vi "Cascade front panel.vi"() -> ()   [LabVIEW 2016]
uses:
  Cascade-lv16-64/Waterloo DAQ/sdi_12/SDI-12/Sonde Vertical Graph.ctl
  Cascade-lv16-64/Waterloo DAQ/controls/Vertical Chart.ctl
  Cascade-lv16-64/Waterloo DAQ/sdi_12/Groundwater header.ctl
  Cascade-lv16-64/Waterloo DAQ/controls/MCC DAQ Setup.ctl
  Cascade-lv16-64/Waterloo DAQ/controls/Aux Sensor.ctl
  Cascade-lv16-64/Waterloo DAQ/KPRO_2016 subvis/Control 2.ctl
  Cascade-lv16-64/Waterloo DAQ/KPRO_2016 subvis/Graph Controls 2.ctl
  Cascade-lv16-64/Waterloo DAQ/KPRO_2016 subvis/Ik control.ctl
  Cascade-lv16-64/Waterloo DAQ/controls/MCC DAQ Readings.ctl
  Cascade-lv16-64/Waterloo DAQ/controls/Kpro pressure measurement cluster.ctl
  Cascade-lv16-64/Waterloo DAQ/controls/Kpro hydraulic measurement cluster.ctl
  Cascade-lv16-64/Waterloo DAQ/sdi_12/Sonde Value Percent Tol.ctl
  Cascade-lv16-64/Waterloo DAQ/activeXtest/activeXtest 2015 Folder/sample data row cluster.ctl
  Cascade-lv16-64/Waterloo DAQ/activeXtest/activeXtest 2015 Folder/sonde cluster.ctl
  Cascade-lv16-64/Waterloo DAQ/KPRO_2016 subvis/Sensor Physical Measurements.ctl
  Cascade-lv16-64/Waterloo DAQ/KPRO_2016 subvis/SS Control 7.ctl
  <vilib>/Utility/NIReport.llb/NI_report.lvclass
  Cascade-lv16-64/Waterloo DAQ/controls/Action Control 1.ctl
  Cascade-lv16-64/Waterloo DAQ/activeXtest/activeXtest 2015 Folder/sonde cluster from excel.ctl
  <extravilib>/ChannelInstances/One Element Stream-t'Action Control 1.ctl'/Instantiate.vi
  <extravilib>/ChannelInstances/One Element Stream-t'Action Control 1.ctl'/Endpoint.vi
  Cascade-lv16-64/Waterloo DAQ/KPRO_2016 subvis/Kpro Globals.vi
  <vilib>/Utility/file.llb/Write Delimited Spreadsheet (string).vi
  <vilib>/Utility/file.llb/Write Delimited Spreadsheet (DBL).vi
  <vilib>/ULx/Create Channel.llb/ULx Create Channel (AI-Voltage-Basic).vi
  <userlib>/_OpenG.lib/file/file.llb/Build Path - Traditional__ogtk.vi
  <userlib>/_OpenG.lib/file/file.llb/Strip Path - Traditional__ogtk.vi
  Cascade-lv16-64/Waterloo DAQ/KPRO_2016 subvis/Global_SIM_switch.vi
  C:/Program Files (x86)/National Instruments/LabVIEW 2016/vi.lib/ULx/ULx_LV.dll
  Program Files (x86)/National Instruments/LabVIEW 2016/vi.lib/ULx/ULx_LV.dll
  <vilib>/Utility/config.llb/NI_LVConfig.lvlib
  <extravilib>/ChannelInstances/One Element Stream-t'Action Control 1.ctl'.lvlib
panel:
  out "Column of Volume":i32
  in  "Input Variables and Slopes 2":T1={"Total Volume"=0.0, "String Pot Slope"=1.6619999408721924, "Flow Slope"=39.040000915527344, "Up Hole Pressure Slope"=48.27000045776367, "Depth to Water Table"=-0.0, "Atmospheric Pressure"=32.22022530555725, "Reservoir Pressure"=-0.004827000045779073, "Height of Sample Box"=0.0, "DH Pressure Trans Slope"=42.0, "DH Pressure Offset"=0.0, "Up Hole  Pressure Offset"=0.0, "Aux 1 Slope"=1.0, "Aux 2 Slope"=1.0, "Aux 3 Slope"=1.0} {"Aux 3 Slope" format="%.2f"; "Aux 2 Slope" format="%.2f"; "Aux 1 Slope" format="%.2f"; "Up Hole  Pressure Offset" format="%.2f"; "DH Pressure Offset" format="%.2f"; "DH Pressure Trans Slope" format="%.2f"; "Height of Sample Box" format="%.2f"; "Reservoir Pressure" format="%.2f"; "Atmospheric Pressure" format="%.2f"; "Depth to Water Table" format="%.2f"; "Up Hole Pressure Slope" format="%.2f"; "Flow Slope" format="%.2f"; "String Pot Slope" format="%.2f"; "Total Volume" format="%.2f"}
  out "Select Worksheet Index":i32
  out "Number of Sample Sheets":i32
  out "NI_report out":refnum<class "NI_report.lvclass">
  out "Sonde":bool
  out "DAQ":bool
  in  "Create Excel Files":bool
  in  "Depth mode":bool caption="Use \nIncrement"
  in  "Sample Sheet Data Row Cluster 2":T2={"Head\nPressure"=0.0, "Depth"=0.0, "comment "="", "Sonde Data Cluster"={"Cumulative\nVolume (ml)"=100.0, "Specific\nCond (mS)"=2.0, "Dissolved\nOxygen mg/L"=3.0, "pH"=4.0, "ORP"=5.0, "Temp deg C"=26.0, "Salinity"=7.0}, "Aux1"=0.0, "Aux2"=0.0, "Aux3"=0.0} {"Sonde Data Cluster"."Salinity" format="%_3g"; "Sonde Data Cluster"."Temp deg C" format="%_2g"; "Sonde Data Cluster"."ORP" format="%_4g"; "Sonde Data Cluster"."pH" format="%_4g"; "Sonde Data Cluster"."Dissolved\nOxygen mg/L" format="%_4g"; "Sonde Data Cluster"."Specific\nCond (mS)" format="%_4g"; "Sonde Data Cluster"."Cumulative\nVolume (ml)" format="%#_4g"; "Depth" format="%#.3g"; "Head\nPressure" format="%#.4g"}
  in  "Increment Depth":bool
  in  "Finish Tests":bool
  in  "Start KPRO":bool
  out "Current Time (s)":dbl
  in  "stop":bool
  in  "Write Data to Spreadsheet":bool
  in  "Sample Not Collected":bool
  in  "Record Single Sample":bool
  in  "Tab Control":T4(tab)
  out "12V Voltage Monitor":dbl format="%_3f"
  out "Found Quanta Sonde Com Port":refnum<visa-resource-name>
  in  "Data File Directory":path=path "C:/Cascade/Data/Excel Reports"
  out "Quanta Sonde found?":bool
  in  "template file path":path=path "C:/Cascade/templates/Groundwater Profiling Log_empty_labview_template.xlsx"
  in  "Config File Path":path=path "C:/Cascade/Data/config files/DAQ Setup Config.ini"
  in  "Read Configuration File?":bool
  out "H-4191 Adapter found":bool
  in  "Save Configuration File?":bool
  out "Sonde Communication Error Out":errorcluster
  in  "Search for Comm Ports?":bool=TRUE
  in  "USB Serial Port Manual Entry":refnum<visa-resource-name>="COM13"
  in  "Sonde Parameters \nTolerance Limits":T5={"SC %"=10.0, "DO %"=10.0, "pH % "=10.0, "ORP % "=10.0, "Temp % "=10.0, "Salinity %"=10.0} {"Salinity %" format="%_2f%%"; "Temp %" format="%_2f%%"; "ORP %" format="%_2f%%"; "pH %" format="%_2f%%"; "DO %" format="%_2f%%"; "SC %" format="%_2f%%"}
  in  "Sonde Parameters \nInitial Values":T6 {"Salinity Initial" format="%_2f"; "Temp Initial" format="%_2f"; "ORP  Initial" format="%_2f"; "pH Initial" format="%_2f"; "DO Initial" format="%_2f"; "SC Initial" format="%_2f"}
  in  "Header path":path=path "C:/Cascade/templates/Fields for Excel sheets.xlsx"
  out "Sensor  Real \nMeasurements":T7 {"9V Monitor" format="%#.3g"; "Aux 3" format="%#.3g"; "Aux 2" format="%#.3g"; "Aux 1" format="%#.3g"; "String Pot" format="%#.3g"; "Top String Pot" format="%#_4g"; "Downhole Pressure" format="%#_4g"; "Flow" format="%#_4g"; "Uphole Pressure" format="%#_4g"}
  in  "MCC USB-DAQ Setup":T8={"Device Name in InstaCal"="Dev0", "Omega Pressure Sensor"={"DAQ Channel"=2.0, "Input Voltage Range"=1, "Enabled"=TRUE, "Description"="Uphole Pressure"}, "McMillian 102 Flowmeter"={"DAQ Channel"=11.0, "Input Voltage Range"=0, "Enabled"=TRUE, "Description"="Flow"}, "DHT Pressure Sensor"={"DAQ Channel"=3.0, "Input Voltage Range"=1, "Enabled"=TRUE, "Description"="Downhole Pressure"}, "Top String Pot"={"DAQ Channel"=0.0, "Input Voltage Range"=0, "Enabled"=TRUE, "Description"="Top String Pot"}, "String Pot Signal"={"DAQ Channel"=1.0, "Input Voltage Range"=0, "Enabled"=TRUE, "Description"="String Pot"}, "Aux Sensor 1"={"DAQ Channel"=5.0, "Input Voltage Range"=1, "Enabled"=TRUE, "Description"="Aux 1"}, "Aux Sensor 2"={"DAQ Channel"=6.0, "Input Voltage Range"=1, "Enabled"=TRUE, "Description"="Aux 2"}, "Aux Sensor 3"={"DAQ Channel"=7.0, "Input Voltage Range"=1, "Enabled"=TRUE, "Description"="Aux 3"}, "Voltage Monitor"={"DAQ Channel"=8.0, "Input Voltage Range"=0, "Enabled"=TRUE, "Description"="9V Monitor"}} {"Voltage Monitor"."Input Voltage Range" items=["+/-10 V Range", "+/-5 V Range", "+/-2.5V Range", "+/-1.25 V Range", "+/-0.625 V Range", "+/-0.3125 V Range", "+/-0.1562V Range", "+/-0.078125 V Range"]; "Aux Sensor 3"."Input Voltage Range" items=["+/-10 V Range", "+/-5 V Range", "+/-2.5V Range", "+/-1.25 V Range", "+/-0.625 V Range", "+/-0.3125 V Range", "+/-0.1562V Range", "+/-0.078125 V Range"]; "Aux Sensor 2"."Input Voltage Range" items=["+/-10 V Range", "+/-5 V Range", "+/-2.5V Range", "+/-1.25 V Range", "+/-0.625 V Range", "+/-0.3125 V Range", "+/-0.1562V Range", "+/-0.078125 V Range"]; "Aux Sensor 1"."Input Voltage Range" items=["+/-10 V Range", "+/-5 V Range", "+/-2.5V Range", "+/-1.25 V Range", "+/-0.625 V Range", "+/-0.3125 V Range", "+/-0.1562V Range", "+/-0.078125 V Range"]; "String Pot Signal"."Input Voltage Range" items=["+/-10 V Range", "+/-5 V Range", "+/-2.5V Range", "+/-1.25 V Range", "+/-0.625 V Range", "+/-0.3125 V Range", "+/-0.1562V Range", "+/-0.078125 V Range"]; "Top String Pot"."Input Voltage Range" items=["+/-10 V Range", "+/-5 V Range", "+/-2.5V Range", "+/-1.25 V Range", "+/-0.625 V Range", "+/-0.3125 V Range", "+/-0.1562V Range", "+/-0.078125 V Range"]; "DHT Pressure Sensor"."Input Voltage Range" items=["+/-10 V Range", "+/-5 V Range", "+/-2.5V Range", "+/-1.25 V Range", "+/-0.625 V Range", "+/-0.3125 V Range", "+/-0.1562V Range", "+/-0.078125 V Range"]; "McMillian 102 Flowmeter"."Input Voltage Range" items=["+/-10 V Range", "+/-5 V Range", "+/-2.5V Range", "+/-1.25 V Range", "+/-0.625 V Range", "+/-0.3125 V Range", "+/-0.1562V Range", "+/-0.078125 V Range"]; "Omega Pressure Sensor"."Input Voltage Range" items=["+/-10 V Range", "+/-5 V Range", "+/-2.5V Range", "+/-1.25 V Range", "+/-0.625 V Range", "+/-0.3125 V Range", "+/-0.1562V Range", "+/-0.078125 V Range"]}
  out "Rate":dbl=1000.0 caption="Channel\nSample Rate (Hz)"
  out "Number \nof Channels":u16
  in  "DAQ \nData Rate S/s":dbl=3720.0 format="%#_13g"
  out "Descriptions":string[](array[string])
  out "Raw Voltages":dbl[](array[numeric])
  out "9V Voltage Monitor":dbl format="%#_3g"
  in  "Record DAQ Raw Voltages":bool
  out "Sensor Voltage Cluster":T10 {"9V Monitor" format="%#.3g"; "Aux 3" format="%#_3g"; "Aux 2" format="%#.3g"; "Aux 1" format="%#.3g"; "String Pot" format="%#.3g"; "Top String Pot" format="%#_3g"; "Downhole Pressure" format="%#.3g"; "Flow" format="%#_3g"; "Uphole Pressure" format="%-#1.3g"}
  out "Worksheet Names":string[](array[string])
  out "row max value":i32
  out "last occupied cell's name":string
  out "column max value":i32
  in  "Current Sheet":i32=1
  out "Current Sample Sheet":string="Sample 1"
  out "Columns":i32[](array[numeric])
  in  "Clear Groundwater Header Values":bool
  in  "Groundwater Header":T11
  in  "Excel report file path":path=path "C:/Cascade/Data/Excel Reports/Groundwater Profiling Log_ara1.xlsx"
  out "Data Setup Indicator":string
  in  "Start Initialization":bool
  in  "Input Variables and Slopes":T1={"Total Volume"=0.0, "String Pot Slope"=1.6619999408721924, "Flow Slope"=39.040000915527344, "Up Hole Pressure Slope"=48.27000045776367, "Depth to Water Table"=-0.0, "Atmospheric Pressure"=32.22022530555725, "Reservoir Pressure"=-0.004827000045779073, "Height of Sample Box"=0.0, "DH Pressure Trans Slope"=42.0, "DH Pressure Offset"=0.0, "Up Hole  Pressure Offset"=0.0, "Aux 1 Slope"=1.0, "Aux 2 Slope"=1.0, "Aux 3 Slope"=1.0} {"Aux 3 Slope" format="%.2f"; "Aux 2 Slope" format="%.2f"; "Aux 1 Slope" format="%.2f"; "Up Hole  Pressure Offset" format="%.2f"; "DH Pressure Offset" format="%.2f"; "DH Pressure Trans Slope" format="%.2f"; "Height of Sample Box" format="%.2f"; "Reservoir Pressure" format="%.2f"; "Atmospheric Pressure" format="%.2f"; "Depth to Water Table" format="%.2f"; "Up Hole Pressure Slope" format="%.2f"; "Flow Slope" format="%.2f"; "String Pot Slope" format="%.2f"; "Total Volume" format="%.2f"}
  out "Up Hole Pressure Offset":dbl
  out "appended path":path
  out "Down hole Pressure Transducer CSV data  path":path
  in  "Static IK path":path
  in  "Slopes File Path":path=path "C:/Cascade/Data/Output Files/slopes.csv"
  out "Output File Path":path
  out "KPRO SessionOutput File Path":path
  in  "Slopes History File Path":path=path "C:/Cascade/Data/Output Files/slopes.csv"
  out "Sonde Recording Error file":path
  out "IK Recording Error file":path
  out "Sonde Output File Path":path
  out "KPRO Cumulative Output File Path":path
  in  "Temporary Data Files Directory":path=path "C:/Cascade/Data/Output Files"
  in  "Update Sonde":bool
  in  "Sonde Data Array":T13(array[cluster]) {"Salinity"."%" format="%_2f%%"; "Salinity"."Value" format="%_4g"; "Temperature"."%" format="%_2f%%"; "Temperature"."Value" format="%_4g"; "ORP"."%" format="%_2f%%"; "ORP"."Value" format="%_4g"; "pH"."%" format="%_2f%%"; "pH"."Value" format="%_4g"; "Dissolved Oxygen"."%" format="%_2f%%"; "Dissolved Oxygen"."Value" format="%_4g"; "Sp. Conductance"."%" format="%_2f%%"; "Sp. Conductance"."Value" format="%_4g"; "Cumulative\nVolume" format="%#_4g"}
  out "Table Label":string="Data from Sample Sheet %d from Excel File"
  out "Sonde Array Size":i32
  out "Sonde Data Display":T14
  out "Temperature":cluster{"Y":dbl[], "Y":dbl[]}[](graph)
  in  "Record  Sonde Reason":bool
  in  "Select Reasons to Record Data":u16(ring) items=["Per Client Request", "Timed Out", "Sample stopped flowing", "Equipment Issue"]
  out "Sonde Recording Failure Path":path
  in  "Sonde IK Recording Failure Path":path
  out "Recording Reason Sonde array":string[][](array[string])
  out "IK Reason array":string[][](array[string])
  out "SC Reference Calibration Response":T16
  out "DO Reference Calibration Response":T16
  out "Salinity Reference Calibration Response":T16
  out "ORP Reference Calibration Response":T16
  out "pH Reference Calibration Response":T16
  out "pH Zero Calibration Response":T16
  in  "Salinity \nReference":dbl
  in  "SC \nReference":dbl
  in  "DO \nReference":dbl
  in  "ORP Reference":dbl
  in  "pH Reference":dbl
  in  "pH Zero":dbl
  in  "Record  SC Calibration":bool
  in  "Record DO Calibration":bool
  in  "Record Salinity Calibration":bool
  in  "Record ORP Calibration":bool
  in  "Record pH Calibration Reference":bool
  in  "Record pH Calibration Zero":bool
  out "KPRO Finish\nIndicator":bool
  in  "Input Depths \nand Parameters Cluster":T17={"Flow"=0.21081600494384767, "Zeroed \nPressure"=74.74207969932556, "Ik"=0.003788962123473114, "Current Depth"=-100.6, "Feet of Stainless"=40, "Start Depth"=0.0, "Abs Start Depth"=0.0} {"Abs Start Depth" format="%.2f"; "Start Depth" format="%.2f"; "Current Depth" format="%.2f"; "Ik" format="%.2f"; "Zeroed \nPressure" format="%.2f"; "Flow" format="%.2f"}
  out "Zero Pressure\nIndicator":bool
  in  "Zero\nPressure":bool caption="Zero Pressure"
  in  "enable_IKMGS_file":bool
  in  "enable_slug_file":bool
  in  "enable_kpro_file":bool=TRUE
  in  "Simulate AD6B":bool
  out "KPRO Test\nIndicator":bool
  in  "Record DTW File":bool
  in  "Zero In-Line Pressure\n(F = leave as is)":bool=TRUE
  out "Current Session":sgl[][](array[numeric]) format="%.2f"
  in  "KPRO test report header":string[](array[string])=["Time(msecs)", "Uncorrected Depth", "Corrected Depth", "Drive_Rate", "Flow", "Feet_of Stainless", "Up Hole Pressure", "IK", "Corrected Pressure", "Atm Pressure", "Depth to water", "Height of box", "Res_Pressure", "Secs_since_1_JAN_1904", "Depth jumps more than 1_foot", "Down hole Pressure"]
  in  "Depth Cluster":T18
  out "Cumulative_data_from_file":sgl[][](array[numeric]) format="%.2f"
  in  "KPRO test report header 2":string[](array[string])=["Time(msecs)", "Uncorrected Depth", "Corrected Depth", "Drive_Rate", "Flow", "Feet_of Stainless", "Up Hole Pressure", "IK", "Corrected Pressure", "Atm Pressure", "Depth to water", "Height of box", "Res_Pressure", "Secs_since_1_JAN_1904", "Depth jumps more than 1_foot", "Down hole Pressure"]
  out "Cumulative_data_ready":bool
  out "Depth Rate\nft/min":dbl format="%#.2g"
  out "Ik":dbl=0.003788962123473114 caption="Real Time - Depth vs. lk" format="%.2f"
  out "Uphole Pressure":dbl format="%.2f"
  in  "New Depth":dbl
  in  "Update Depth":bool
  in  "Select Entry for IK Log":u16(ring) items=["IK Increase", "IK stayed the Same", "IK decreased"]
  out "Large Depth IK Graph Cluster":T19={[0.003788962123473114, 0.0037174584307500765, 0.0037174584307500765, 0.0037174584307500765, 0.0037174584307500765, 0.003788962123473114], [-100.1, -100.2, -100.3, -100.4, -100.5, -100.6]}
  in  "Culmulative Graph Cluster":T20={"Cumulative - Depth vs. Ik"={[], []}, "Real Time - Depth vs. lk "={[0.003788962123473114, 0.0037174584307500765, 0.0037174584307500765, 0.0037174584307500765, 0.0037174584307500765, 0.003788962123473114], [-100.1, -100.2, -100.3, -100.4, -100.5, -100.6]}, "Cumulative - Depth vs. Drive Rate"={[], []}, "Real Time - Depth vs. Drive Rate"={[0.02036245163917736, 0.125, 0.16666666666666674, 0.16666666666666663, 0.16666666666666663, 0.16666666666666663], [-100.1, -100.2, -100.3, -100.4, -100.5, -100.6]}}
  out "Down hole Pressure":dbl format="%.2f"
  in  "Record IK Reason":bool
  in  "Corrected\n Pressure \nCluster":T21
  out "Flow":dbl format="%#.2g"
  out "Current Depth":sgl=-100.6 format="%.2f"
  out "Current \nDepth (m)":sgl=-30.661383 format="%.2f"
  in  "Read String Pot":bool
  out "Large Depth IK Graph":dbl(graph)
  out "DAQ Error":errorcluster
  out "Initialization Finished":bool=TRUE
  out "Stop":bool
  out "error out":errorcluster
  in  "error in (no error)":errorcluster
  out "producer loop":i32
  out "consumer loop":i32
  out "Active Channel Array":string[](array[string])
  out "delimited string":string
  out "Voltage Range":dbl[](array[numeric])
  out "Stop 2":bool
  out "output cluster":T3 caption="Cluster" {"Salinity" format="%_3g"; "Temp deg C" format="%_2g"; "ORP" format="%_4g"; "pH" format="%_4g"; "Dissolved\nOxygen mg/L" format="%_3g"; "Specific\nCond (mS)" format="%_4g"; "Cumulative\nVolume (ml)" format="%#_4g"}
  out "Serial Number/MISC":string
  out "subarray":string[][](array[string])
  out "Initialization":i32
  in  "Record Continuous Samples":bool
  # "ft. water"
  # "mL/min."
  # "ft. water"
  # "ft."
  # "ft."
  # "Instructions for Sonde Calibration:\n1.  Use the Record Single Point to Record the Data prior to start of\ncalibration procedure to record the initial points to the excel worksheet.\n2.  pH Calibration is a 2 step process:  A pH standard between 6.8 and 7.2 is treated as the “zero”\nand all other values are treated as the “slope”. First calibrate “zero”, then  add a second to calibrate “slope”. \n3.  Specific Conductance:  Wait for the specific conductance readings to stabilize in the calibration solution, which may\nrequire one or two minutes."
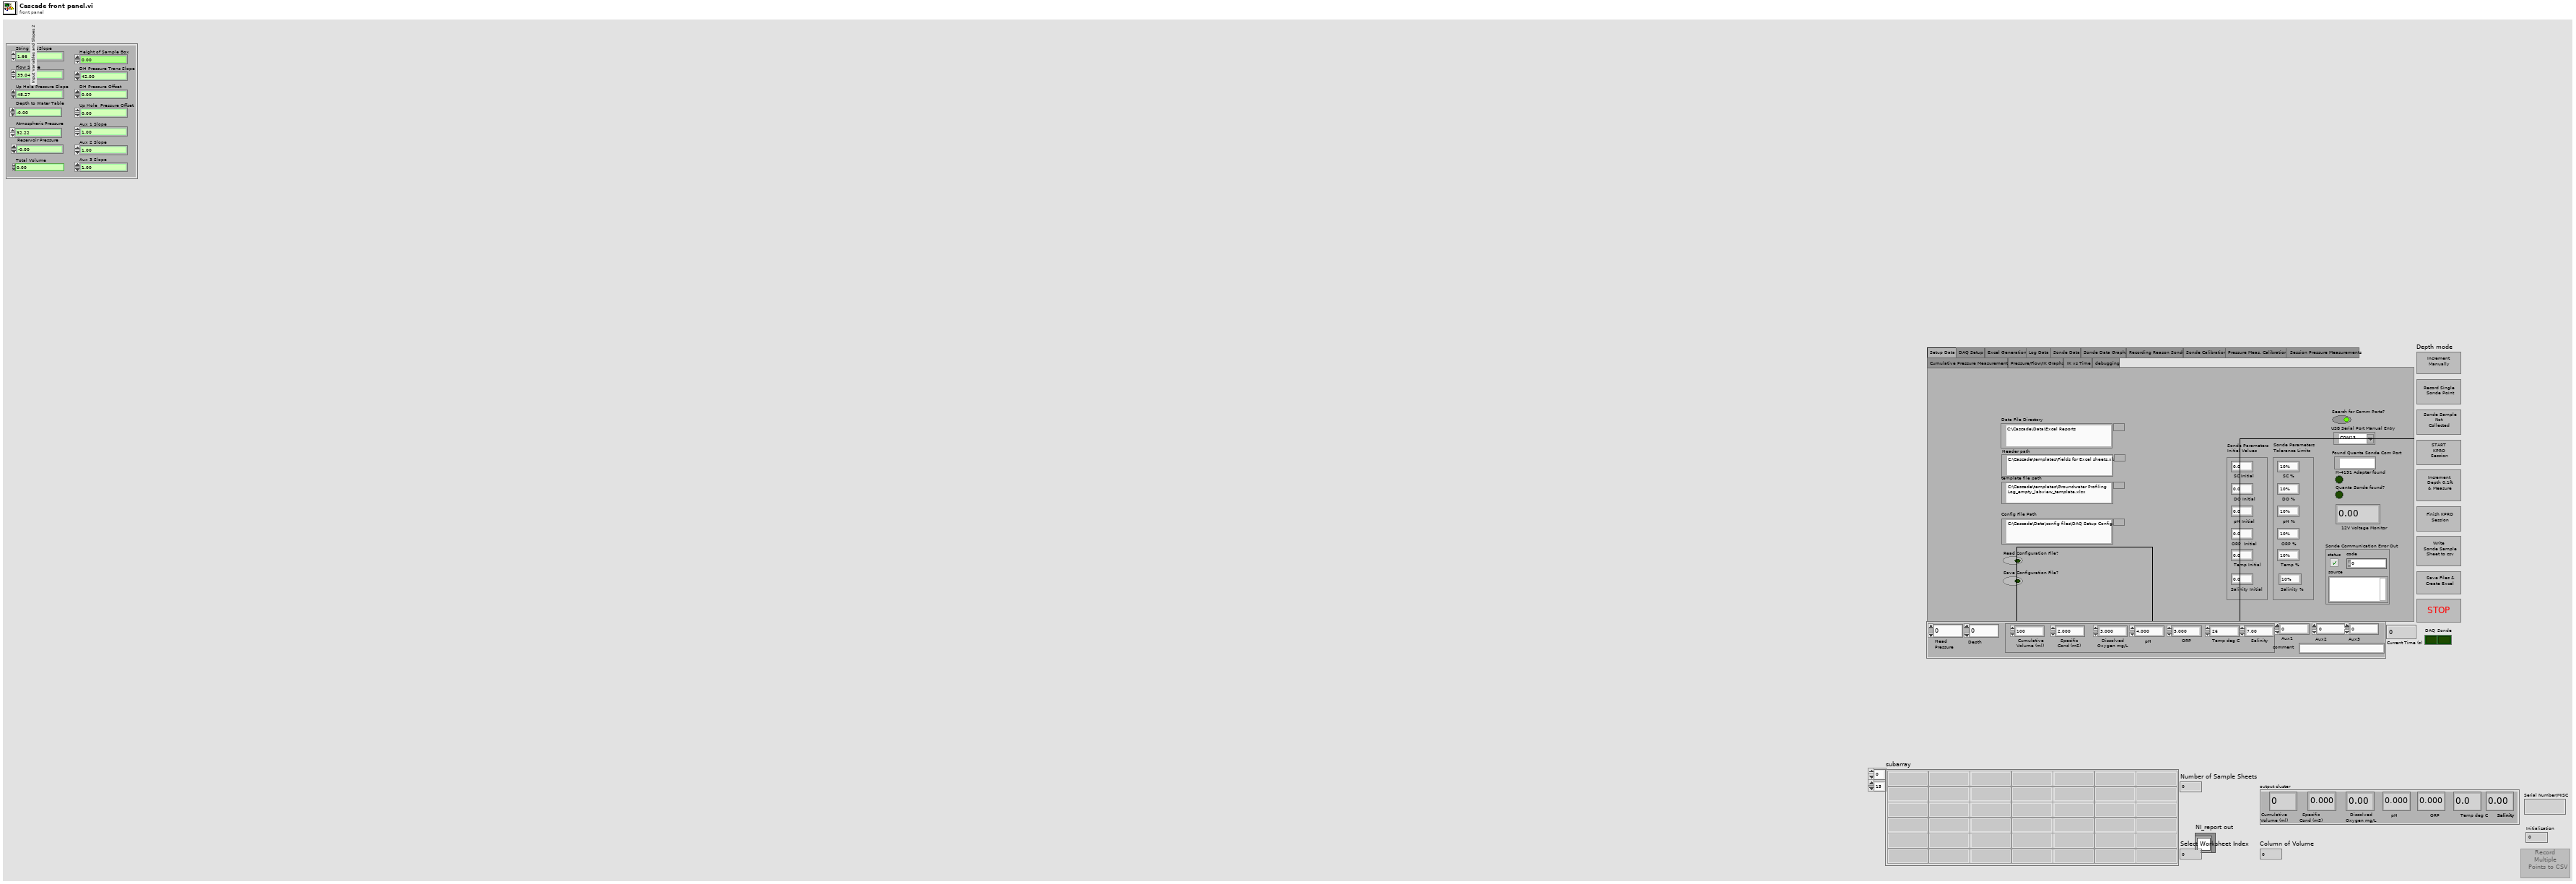
[diagram p1: front panel]
types:
  T1 = typedef "Control 2.ctl" = cluster{"Total Volume":dbl, "String Pot Slope":dbl, "Flow Slope":dbl, "Up Hole Pressure Slope":dbl, "Depth to Water Table":dbl, "Atmospheric Pressure":dbl, "Reservoir Pressure":dbl, "Height of Sample Box":dbl, "DH Pressure Trans Slope":dbl, "DH Pressure Offset":dbl, "Up Hole  Pressure Offset":dbl, "Aux 1 Slope":dbl, "Aux 2 Slope":dbl, "Aux 3 Slope":dbl}
  T2 = typedef "sample data row cluster.ctl" = cluster{"Head\nPressure":dbl, "Depth":dbl, "comment ":string, "Sonde Data Cluster":T3, "Aux1":dbl, "Aux2":dbl, "Aux3":dbl}
  T3 = typedef "sonde cluster.ctl" = cluster{"Cumulative\nVolume (ml)":dbl, "Specific\nCond (mS)":dbl, "Dissolved\nOxygen mg/L":dbl, "pH":dbl, "ORP":dbl, "Temp deg C":dbl, "Salinity":dbl}
  T4 = enum32{"Setup Data", "DAQ Setup", "Excel Generation", "Log Data", "Sonde Data", "Sonde Data Graphs", "Recording Reason Sonde", "Sonde Calibration", "Pressure Meas. Calibration", " Session Pressure Measurements", "Cumulative Pressure Measurements", "Pressure/Flow/IK Graphs", "IK vs Time ", "debugging"}
  T5 = cluster{"SC %":dbl, "DO %":dbl, "pH % ":dbl, "ORP % ":dbl, "Temp % ":dbl, "Salinity %":dbl}
  T6 = cluster{"SC Initial ":dbl, "DO Initial ":dbl, "pH Initial  ":dbl, "ORP  Initial":dbl, "Temp Initial":dbl, "Salinity Initial ":dbl}
  T7 = typedef "Sensor Physical Measurements.ctl" = cluster{"Uphole Pressure":dbl, "Flow":dbl, "Downhole Pressure":dbl, "Top String Pot":dbl, "String Pot":dbl, "Aux 1":dbl, "Aux 2":dbl, "Aux 3":dbl, "9V Monitor":dbl}
  T8 = typedef "MCC DAQ Setup.ctl" = cluster{"Device Name in InstaCal":string, "Omega Pressure Sensor":T9, "McMillian 102 Flowmeter":T9, "DHT Pressure Sensor":T9, "Top String Pot":T9, "String Pot Signal":T9, "Aux Sensor 1":T9, "Aux Sensor 2":T9, "Aux Sensor 3":T9, "Voltage Monitor":T9}
  T9 = typedef "Aux Sensor.ctl" = cluster{"DAQ Channel":dbl, "Input Voltage Range":u16, "Enabled":bool, "Description":string}
  T10 = typedef "MCC DAQ Readings.ctl" = cluster{"Uphole Pressure":dbl, "Flow":dbl, "Downhole Pressure":dbl, "Top String Pot":dbl, "String Pot":dbl, "Aux 1":dbl, "Aux 2":dbl, "Aux 3":dbl, "9V Monitor":dbl}
  T11 = typedef "Groundwater header.ctl" = cluster{"Location":string, "Date Finished":string, "CTS":string, "sampler":string, "Kpro box Serial ":string, "Sonde Serial":string, "Drilling Contractor":string, "Ave Depth to Water":string, "Gas/Peri Pump":string, "Atmospheric Pressure":string, "KPRO N2 Pressure":string, "Gas Drive N2 Pressure":string, "Profile ID":string}
  T12 = typedef "Sonde Value Percent Tol.ctl" = cluster{"Value":dbl, "%":dbl, "Tol.":bool}
  T13 = cluster{"Head":dbl, "Depth":dbl, "Time":string, "Cumulative\nVolume":dbl, "Sp. Conductance":T12, "Dissolved Oxygen":T12, "pH":T12, "ORP":T12, "Temperature":T12, "Salinity":T12, "Final Tol.":bool, "Final":bool, "Time 2":timestamp, "Aux 1":dbl, "Aux 2":dbl, "Aux 3":dbl}[]
  T14 = typedef "Sonde Vertical Graph.ctl" = cluster{"pH":T15, "Conductance":T15, "Salinity":T15, "DO % Saturation":T15, "DO mg/L":T15, "ORP":T15}
  T15 = typedef "Vertical Chart.ctl" = cluster{"Y":dbl[], "Y":dbl[]}[]
  T16 = cluster{"Valid":bool, "Value":dbl, "\nString ":string}
  T17 = typedef "SS Control 7.ctl" = cluster{"Flow":dbl, "Zeroed \nPressure":dbl, "Ik":dbl, "Current Depth":sgl, "Feet of Stainless":i32, "Start Depth":sgl, "Abs Start Depth":sgl}
  T18 = typedef "Kpro hydraulic measurement cluster.ctl" = cluster{"Absolute Depth In":dbl, "Current Absolute Depth":dbl, "First Absolute Depth":dbl, "Previous Relative Depth":dbl, "Current Relative Depth":dbl, "First Relative Depth":dbl, "Last Filed Depth":dbl, "Total Volume In":dbl, "Total Volume Out":dbl, "Current Measurement Time":dbl, "Previous Measurement Time":dbl}
  T19 = typedef "Ik control.ctl" = cluster{dbl[], dbl[]}
  T20 = typedef "Graph Controls 2.ctl" = cluster{"Cumulative - Depth vs. Ik":cluster{dbl[], dbl[]}, "Real Time - Depth vs. lk ":cluster{dbl[], dbl[]}, "Cumulative - Depth vs. Drive Rate":cluster{dbl[], dbl[]}, "Real Time - Depth vs. Drive Rate":cluster{dbl[], dbl[]}}
  T21 = typedef "Kpro pressure measurement cluster.ctl" = cluster{"Up hole Corrected Pressure":dbl, "Down hole Corrected Pressure":dbl}
  T22 = typedef "NI_LVConfig.lvlib/Config Data RefNum.ctl" = refnum<k1>
  T23 = enum8{"Enabled", "Disabled", "Disabled and Grayed Out"}
  T24 = typedef "Action Control 1.ctl" = enum16{"TimeOut", "Continuous  Sonde Data", "Init", "Exit", "Acq. Single Sonde Point", "Write Sonde Sample Sheet", "Acq. DAQ data", "Sample Not Collected", "Record Sonde Reason", "pH Calibration Zero", "pH Calibration Standard", "ORP Calibration Standard", "Salinity Calibration Standard", "DO Calibration Standard", "SC Calibration Standard", "Increment Depth Manually", "Start KPRO Measurements", "Finish KPRO Measurements", "Update Depth", "IK vs Time", "Record IK Reason", "Create Excel Files"}
  T25 = typedef "One Element Stream-t'Action Control 1.ctl'.lvlib/)Channel.ctl" = refnum<queue>
  T26 = typedef "sonde cluster from excel.ctl" = cluster{"Head":dbl, "Depth":dbl, "Time":string, "Cumulative\nVolume":dbl, "Sp. Conductance":T12, "Dissolved Oxygen":T12, "pH":T12, "ORP":T12, "Temperature":T12, "Salinity":T12, "Final Tol.":bool, "Final":bool, "Time 2":timestamp, "Aux 1":dbl, "Aux 2":dbl, "Aux 3":dbl}
  T27 = cluster{"Head":dbl, "Depth":dbl, "Time":string, "Cumulative\nVolume":dbl, "Sp. Conductance":T12, "Dissolved Oxygen":T12, "pH":T12, "ORP":T12, "Temperature":T12, "Salinity":T12, "Final Tol.":bool, "Final":bool, "Time 2":timestamp, "Aux 1":dbl, "Aux 2":dbl, "Aux 3":dbl}
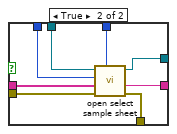
[diagram p2: hidden frame]
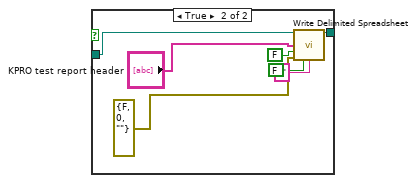
[diagram p9: hidden frame]
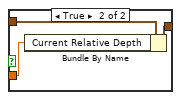
[diagram p11: hidden frame]
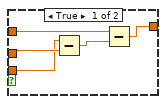
[diagram p12: hidden frame]
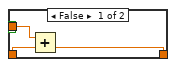
[diagram p18: hidden frame]
diagram:
  # "For calibrate command (XC) on SDI-12 address ‘a’, P is pH, C is specific conductance, S is\nsalinity or TDS, % is DO %Saturation, O is DO mg/L, R is ORP, D is depth, B is\nbarometric pressure, and t is TDS scale factor."
  n1 = flat-sequence {
    tunnel: [w20] -> w5
    tunnel: [w52] -> w7
    tunnel: w5 -> [w52]
    tunnel: [w48] -> w3
    tunnel: [w54] -> w14
    tunnel: w7 -> [w58]
    tunnel: [w54] -> w6
    tunnel: w14 -> [w108]
    tunnel: [w99] -> w12
    tunnel: [w103] -> w11
    tunnel: [w102] -> w8
    tunnel: [w100] -> w9
    tunnel: [w101] -> w10
    tunnel: [w104] -> _
    tunnel: [w106] -> w13
    tunnel: [w109] -> w2
    tunnel: [w110] -> w1
    frame #0 {
      n2 = invoke on="error out" class="Clust (strict)" method="Reinit To Default"(error in="error in (no error)") -> (error out=w18:errorcluster)  [unwired: 2 in, 2 out]
      n3 = flat-sequence {
        tunnel: [w24] -> w20
        tunnel: w18 -> [w23]
        frame #0 {
          n4 = case shown="False" "Read Configuration File?" {
            selector: "Read Configuration File?" -> [_ w31]
            tunnel: [w25 w36] -> w24
            tunnel: w23 -> [w25 w33]
            tunnel: "Config File Path" -> [_ w32]
            frame False {
            }
            frame True {
              n5 = call <vilib>:"Check if File or Folder Exists.vi"("error in (no error)"=w33, "path"=w32) -> ("error out"=w28:errorcluster, "file or folder exists?"=w29:bool, "dup path"=w27:path)  [unwired: 7 in]
              n6 = And(x=w31, y=w29) -> (x .and. y?=w30:bool)
              n7 = control-ref of="This VI"() -> (w34:refnum<vi>)
              n8 = case shown="True" w30 {
                selector: w30 -> [w37 _]
                tunnel: w27 -> [_ w42]
                tunnel: w28 -> [w38 w46]
                tunnel: [w38 w39] -> w35
                tunnel: w34 -> [_ w47]
                frame False {
                  n9 = local write "Read Configuration File?"(w37) -> ()
                }
                frame True {
                  n10 = call <vilib>:"Open Config Data.vi"("error in (no error)"=w46, "create file if necessary (T)"=FALSE, "configuration file path"=w42) -> ("error out"=w44:errorcluster, "refnum"=w45:T22)  [unwired: 6 in, 1 out]
                  n11 = call <userlib>:"Read Panel from INI__ogtk.vi"("error in (no error)"=w44, "VI ref"=w47, "refnum"=w45) -> ("error out"=w40:errorcluster, "refnum out"=w41:T22)  [unwired: 7 in]
                  n12 = call <vilib>:"Close Config Data.vi"("error in (no error)"=w40, "refnum"=w41) -> ("error out"=w39:errorcluster)  [unwired: 8 in, 1 out]
                }
              }
              n13 = call <vilib>:"Clear Errors.vi"("error in (no error)"=w35) -> ("error out"=w26:errorcluster)  [unwired: 5 in, 1 out]
              n14 = Merge Errors(w26) -> (w36:errorcluster)
            }
          }
        }
      }
    }
    frame #1 {
      n15 = invoke on="Current Session" class="Arr (strict)" method="Reinit To Default"() -> ()  [unwired: 3 in, 3 out]
      n16 = control-ref of="Sonde Data Display"() -> ()  [unwired: 1 out]
      n17 = local write "Current Sheet"(1 ("Current Sheet")) -> ()
      n18 = Get Date/Time In Seconds() -> (seconds since 1Jan1904=w48:timestamp)
      n19 = Get Date/Time In Seconds() -> (seconds since 1Jan1904=w49:timestamp)
      n20 = Subtract(x=w48, y=w49) -> (x-y=w50:dbl)
      n21 = To Double Precision Float(number=w50) -> (double precision float=→"Current Time (s)":dbl)
    }
    frame #2 {
      w66 = T23."Enabled" ("Disabled")
      w84 = T23."Disabled and Grayed Out" ("Disabled")
      n22 = invoke on="Current Sheet" class="DigNum (strict)" method="Reinit To Default"(error in=w58) -> (error out=w78:errorcluster)  [unwired: 2 in, 2 out]
      n23 = local write "Initialization Finished"(FALSE ("Initialization Finished")) -> ()
      n24 = invoke on="Sample Not Collected" class="Bool" method="Reinit To Default"(error in=w78) -> (error out=w81:errorcluster)  [unwired: 2 in, 2 out]
      n25 = invoke on="Record Continuous Samples" class="Bool" method="Reinit To Default"(error in=w81) -> (error out=w80:errorcluster)  [unwired: 2 in, 2 out]
      n26 = invoke on="Write Data to Spreadsheet" class="Bool" method="Reinit To Default"(error in=w80) -> (error out=w79:errorcluster)  [unwired: 2 in, 2 out]
      n27 = call "search for Quanta Sonde devices.vi"("VISA resource name"="USB Serial Port Manual Entry", "Search for Comm Ports?"="Search for Comm Ports?", "error in (no error)"=w58) -> ("12V monitor"=w65:dbl, "Com Port with Quanta Sonde devices"=w90:refnum<visa-resource-name>[], "Number of Quanta Sonde devices"=w89:i32, "Serial Number/MISC"=w68:string, "Number of Quanta Sonde devices > 0?"=→"Quanta Sonde found?":bool, "H-4191 Adapter found"=→"H-4191 Adapter found":bool, "Error Out"=w73:errorcluster)  [unwired: 4 in, 2 out]
      "12V Voltage Monitor" <- w65
      "Sonde Communication Error Out" <- w73
      "Serial Number/MISC" <- w68
      n28 = invoke on="Record Single Sample" class="Bool" method="Reinit To Default"(error in=w79) -> (error out=w57:errorcluster)  [unwired: 2 in, 2 out]
      n29 = property on="Record Continuous Samples" class="Bool"(error in=w57, "DisabledEnum"=w84) -> (error out=w85:errorcluster)  [unwired: 1 in, 1 out]
      n30 = local read "Groundwater Header"() -> (w67:T11)
      n31 = Greater Or Equal?(x=w65, y=11.75) -> (x >= y?=→"Sonde":bool)
      n32 = case shown="1" w89 {
        tunnel: w90 -> [_ w97]
        tunnel: [refnum<visa-resource-name> refnum ("RS232 Port Out") w95] -> w88
        frame 0, Default {
        }
        frame 1 {
          n33 = Index Array(array=w97, index=0) -> (element=w95:refnum<visa-resource-name>)
        }
      }
      "Found Quanta Sonde Com Port" <- w88
      n34 = property on="Record Single Sample" class="Bool"(error in=w85, "DisabledEnum"=w84) -> (error out=w86:errorcluster)  [unwired: 1 in, 1 out]
      n35 = invoke on="stop" class="Bool (strict)" method="Reinit To Default"(error in=w57) -> (error out=w83:errorcluster)  [unwired: 2 in, 2 out]
      n36 = Bundle By Name(cluster=w67, "Sonde Serial"=w68) -> (w69:T11)
      n37 = invoke on="Stop" class="Bool (strict)" method="Reinit To Default"(error in=w57) -> (error out=w75:errorcluster)  [unwired: 2 in, 2 out]
      n38 = property on="Sample Not Collected" class="Bool"(error in=w86, "DisabledEnum"=w84) -> (error out=w82:errorcluster)  [unwired: 1 in, 1 out]
      n39 = local write "Groundwater Header"(w69) -> ()
      n40 = property on="Write Data to Spreadsheet" class="Bool"(error in=w83, "DisabledEnum"=w84) -> (error out=w76:errorcluster)  [unwired: 1 in, 1 out]
      n41 = invoke on="Stop 2" class="Bool (strict)" method="Reinit To Default"(error in=w75) -> (error out=w74:errorcluster)  [unwired: 2 in, 2 out]
      n42 = call <vilib>:"Clear Errors.vi"("error in (no error)"=w73) -> ("error out"=w72:errorcluster)  [unwired: 5 in, 1 out]
      n43 = Merge Errors(w72, w74, w76, w82) -> (w55:errorcluster)
      n44 = flat-sequence {
        tunnel: [w93] -> w62
        tunnel: w55 -> [w93]
        frame #0 {
          n45 = local write "Tab Control"(T4."Log Data" ("Tab Control")) -> ()
        }
      }
      n46 = invoke on="Sonde Data Array" class="Arr (strict)" method="Reinit To Default"(error in=w62) -> (error out=w61:errorcluster)  [unwired: 2 in, 2 out]
      n47 = invoke on="Data Setup Indicator" class="Str" method="Reinit To Default"(error in=w61) -> (error out=w59:errorcluster)  [unwired: 2 in, 2 out]
      n48 = property on="Clear Groundwater Header Values" class="Bool"(error in=w59, "DisabledEnum"=w66) -> (error out=w60:errorcluster)  [unwired: 1 in, 1 out]
      n49 = property on="Start Initialization" class="Bool"(error in=w60, "DisabledEnum"=w66) -> (error out=w56:errorcluster)  [unwired: 1 in, 1 out]
      n50 = invoke on="Clear Groundwater Header Values" class="Bool" method="Reinit To Default"(error in=w56) -> (error out=w54:errorcluster)  [unwired: 2 in, 2 out]
    }
    frame #3 {
      n51 = while {
        tunnel: w108 -> [w118]
        tunnel: [w119] -> w105
        tunnel: [w124] -> _
        i -> [w124]
        stop <- w120 stop-if-true
        n52 = event shown="[3] \"Stop\": Value Change" {
          selector: _ -> [_ _ _ _ _]
          dyn-events: _ -> [_ _ _ _ _]
          timeout: 100 -> [_ _ _ _ _]
          tunnel: [FALSE w134 TRUE ("Stop") w139 _] -> w126
          tunnel: w118 -> [_ _ _ _ w142]
          event Timeout {
            n53 = event-data() -> ()  [unwired: 1 in, 3 out]
          }
          event "Start Initialization": Value Change {
            n54 = event-data() -> ()  [unwired: 1 in, 3 out]
            n55 = case shown="True" "Start Initialization" {
              tunnel: [FALSE ("Stop") TRUE ("Stop")] -> w134
              frame False {
              }
              frame True {
                n56 = invoke on="Data Setup Indicator" class="Str" method="Reinit To Default"() -> ()  [unwired: 3 in, 3 out]
                n57 = invoke on="Start Initialization" class="Bool" method="Reinit To Default"() -> ()  [unwired: 3 in, 3 out]
              }
            }
          }
          event Panel Close? {
            n58 = event-data() -> ()  [unwired: 1 in, 4 out]
            n59 = event-data() -> ()  [unwired: 2 in, 1 out]
          }
          event "Stop": Value Change {
            n60 = event-data() -> ()  [unwired: 1 in, 6 out]
            n61 = local read "stop"() -> (w138:bool)
            n62 = case shown="True" w138 {
              selector: w138 -> [w140 _]
              tunnel: [w140 TRUE] -> w139
              tunnel: w138 -> [_ _]
              frame False {
              }
              frame True {
              }
            }
          }
          event "Clear Groundwater Header Values": Value Change {
            n63 = event-data() -> ()  [unwired: 1 in, 6 out]
            n64 = case shown="True" "Clear Groundwater Header Values" {
              tunnel: w142 -> [_ w144]
              frame False {
              }
              frame True {
                n65 = invoke on="Groundwater Header" class="Clust (strict)" method="Reinit To Default"(error in=w144) -> (error out=w145:errorcluster)  [unwired: 2 in, 2 out]
                n66 = flat-sequence {
                  tunnel: w145 -> [_]
                  frame #0 {
                    n67 = local read "Groundwater Header"() -> (w146:T11)
                    n68 = local read "Serial Number/MISC"() -> (w147:string)
                    n69 = Bundle By Name(cluster=w146, "Sonde Serial"=w147) -> (w148:T11)
                    n70 = local write "Groundwater Header"(w148) -> ()
                  }
                }
              }
            }
          }
        }
        n71 = call <userlib>:"Wait (ms)__ogtk.vi"("error in (no error)"=w118, "milliseconds to wait"=u32 100) -> ("error out"=w119:errorcluster)  [unwired: 8 in, 1 out]
        n72 = Quotient & Remainder(x=w124, y=100) -> (floor(x/y)=w121:i32)  [unwired: 1 out]
        n73 = case shown="1, Default" w121 {
          tunnel: w119 -> [w129 w131]
          frame 1, Default {
            n74 = property on="Data Setup Indicator" class="Str"(error in=w129, "Text.TextColor"=u32 0) -> ()  [unwired: 1 in, 2 out]
          }
          frame 0 {
            n75 = property on="Data Setup Indicator" class="Str"(error in=w131, "Text.TextColor"=u32 16716800) -> ()  [unwired: 1 in, 2 out]
          }
        }
        n76 = local read "stop"() -> (w117:bool)
        n77 = Compound Arithmetic op=OR(w119, w126, w117) -> (w120:bool)
        "Data Setup Indicator" <- "Hit the Start Key after Data Entry of Log Parameters and File Names." ("Data Setup Indicator")
      }
      n78 = invoke on="stop" class="Bool (strict)" method="Reinit To Default"(error in=w105) -> (error out=w98:errorcluster)  [unwired: 2 in, 2 out]
      n79 = flat-sequence {
        tunnel: w98 -> [w155]
        tunnel: [w149] -> w107
        frame #0 {
          w156 = T23."Disabled and Grayed Out" ("Disabled")
          n80 = local write "KPRO Finish\nIndicator"(FALSE ("KPRO Finish\nIndicator")) -> ()
          n81 = invoke on="Start KPRO" class="Bool" method="Reinit To Default"(error in=w155) -> (error out=w154:errorcluster)  [unwired: 2 in, 2 out]
          n82 = invoke on="Finish Tests" class="Bool" method="Reinit To Default"(error in=w154) -> (error out=w153:errorcluster)  [unwired: 2 in, 2 out]
          n83 = invoke on="Sonde Array Size" class="DigNum (strict)" method="Reinit To Default"() -> ()  [unwired: 3 in, 3 out]
          n84 = invoke on="Increment Depth" class="Bool" method="Reinit To Default"(error in=w153) -> (error out=w152:errorcluster)  [unwired: 2 in, 2 out]
          n85 = property on="Clear Groundwater Header Values" class="Bool"(error in=w152, "DisabledEnum"=w156) -> (error out=w151:errorcluster)  [unwired: 1 in, 1 out]
          n86 = property on="Start Initialization" class="Bool"(error in=w151, "DisabledEnum"=w156) -> (error out=w150:errorcluster)  [unwired: 1 in, 1 out]
          n87 = invoke on="Update Sonde" class="Bool (strict)" method="Reinit To Default"(error in=w150) -> (error out=w149:errorcluster)  [unwired: 2 in, 2 out]
        }
      }
      n88 = flat-sequence {
        tunnel: [w159] -> w110
        tunnel: [w159] -> w109
        tunnel: [w164] -> w106
        tunnel: w107 -> [w163]
        frame #0 {
          n89 = Unbundle By Name("Input Variables and Slopes") -> ("Depth to Water Table"=w169:dbl)
          n90 = local read "Input Depths \nand Parameters Cluster"() -> (w161:T17)
          n91 = Bundle By Name(cluster="Input Variables and Slopes", "Depth to Water Table"=w169) -> (w166:T1)
          n92 = call <vilib>:"Check if File or Folder Exists.vi"("error in (no error)"=w163, "path"="Slopes File Path") -> ("error out"=w162:errorcluster, "file or folder exists?"=w158:bool, "dup path"=w167:path)  [unwired: 7 in]
          n93 = case shown="True" w158 {
            tunnel: w167 -> [_ w185]
            tunnel: w166 -> [w173 w184]
            tunnel: [w173 w183] -> w165
            tunnel: w162 -> [w172 w179]
            tunnel: [w172 w179] -> w164
            frame False {
              n94 = local write "Data Setup Indicator"("Slope file not found." ("Data Setup Indicator")) -> ()
            }
            frame True {
              n95 = call "Get_SLOPE_data_from_file 2016.vi"("Slopes File Path"=w185) -> ("Last Aux 1 Slope"=w178:dbl, "Last_String_Pot_Slope"=w182:dbl, "DHT Offset"=w174:dbl, "DHT Slope"=w175:dbl, "Last_Flow_Slope"=w181:dbl, "Last Aux 2 Slope"=w177:dbl, "Last Aux 3 Slope"=w176:dbl, "Last_Pressure_Slope"=w180:dbl)  [unwired: 6 in, 1 out]
              n96 = Bundle By Name(cluster=w184, "String Pot Slope"=w182, "Flow Slope"=w181, "Up Hole Pressure Slope"=w180, "Aux 1 Slope"=w178, "Aux 2 Slope"=w177, "Aux 3 Slope"=w176, "DH Pressure Trans Slope"=w175, "DH Pressure Offset"=w174) -> (w183:T1)
            }
          }
          n97 = Unbundle By Name(w161) -> ("Feet of Stainless"=w159:i32)
          n98 = Bundle By Name(cluster=w161, "Feet of Stainless"=w159) -> (w160:T17)
          n99 = local write "Input Depths \nand Parameters Cluster"(w160) -> ()
          n100 = local write "Input Variables and Slopes"(w165) -> ()
        }
      }
      n101 = flat-sequence {
        tunnel: [w116] -> w104
        tunnel: [w115] -> w103
        tunnel: [w114] -> w102
        tunnel: [w113] -> w101
        tunnel: [w112] -> w100
        tunnel: [w111] -> w99
        frame #0 {
          n102 = local read "Column of Volume"() -> (w112:i32)
          n103 = local read "NI_report out"() -> (w111:refnum<class "NI_report.lvclass">)
          n104 = local read "Select Worksheet Index"() -> (w116:i32)
          n105 = local read "Number of Sample Sheets"() -> (w114:i32)
          n106 = local read "Columns"() -> (w113:i32[])
          n107 = local read "Worksheet Names"() -> (w115:string[])
        }
      }
    }
  }
  n108 = flat-sequence {
    tunnel: [w189] -> w17
    tunnel: w13 -> [w188]
    tunnel: [w187] -> w4
    frame #0 {
      w186 = Action_Control_1."Init"  # Event
      n109 = while {
        shift-right: [w197] -> w189
        shift-left: w188 -> [w197]
        shift-right: [w192] -> _
        shift-left: w186 -> [w190]
        tunnel: [w198] -> w187
        i -> [w196]
        stop <- w194 stop-if-true
        # "User Interface Producer Loop"
        n110 = First Call?() -> (First Call?: T/F=w191:bool)
        n111 = case shown="False" w191 {
          tunnel: w197 -> [w203 _]
          tunnel: [w201 FALSE ("Boolean")] -> w194
          tunnel: [w200 w395] -> w192
          tunnel: w190 -> [_ w395]
          frame False {
            w199 = Action_Control_1."TimeOut"  # Event
            n112 = event shown="[0] Timeout" {
              selector: _ -> [_ _ _ _ _ _ _ _ _ _ _ _ _ _ _ _ _ _ _ _]
              dyn-events: _ -> [_ _ _ _ _ _ _ _ _ _ _ _ _ _ _ _ _ _ _ _]
              timeout: 100 -> [_ _ _ _ _ _ _ _ _ _ _ _ _ _ _ _ _ _ _ _]
              tunnel: [w204 w210 w216 w229 w239 w248 w260 w272 w284 w296 w308 w321 w332 w342 w350 w358 w366 w375 w383 _] -> w200
              tunnel: [FALSE w209 w217 w230 w240 w249 w261 w273 w285 w297 w309 w320 w331 w343 w351 w359 w367 w376 w384 _] -> w201
              tunnel: w203 -> [_ w207 w219 w232 _ w251 w263 w275 w287 w299 w311 _ w328 _ _ _ _ _ _ _]
              tunnel: [_ w207 w218 w231 _ w250 w262 w274 w286 w298 w310 _ _ _ _ _ _ _ _ _] -> _
              tunnel: w199 -> [w204 w206 w215 w228 _ w247 w259 w271 w283 w295 w307 w319 w326 w340 w348 w357 w365 w374 w382 _]
              event Timeout {
                n113 = event-data() -> ()  [unwired: 1 in, 3 out]
              }
              event "stop": Value Change {
                n114 = event-data() -> ()  [unwired: 1 in, 6 out]
                n115 = case shown="False" "stop" {
                  tunnel: [w211 w213] -> w210
                  tunnel: [FALSE TRUE] -> w209
                  tunnel: w206 -> [w211 _]
                  frame False {
                  }
                  frame True {
                    w213 = Action_Control_1."Exit"  # Event
                  }
                }
              }
              event "Record DAQ Raw Voltages": Value Change {
                n116 = event-data() -> ()  [unwired: 1 in, 6 out]
                n117 = case shown="False" "Record DAQ Raw Voltages" {
                  tunnel: [w221 w224] -> w216
                  tunnel: [FALSE FALSE ("Boolean")] -> w217
                  tunnel: [w222 w225] -> w218
                  tunnel: w219 -> [w222 w225]
                  tunnel: w215 -> [w221 _]
                  frame False {
                  }
                  frame True {
                    w224 = Action_Control_1."Acq. DAQ data"  # Event
                  }
                }
              }
              event "Record pH Calibration Zero": Value Change {
                n118 = event-data() -> ()  [unwired: 1 in, 6 out]
                n119 = case shown="True" "Record pH Calibration Zero" {
                  tunnel: [w233 w236] -> w229
                  tunnel: [FALSE FALSE ("Boolean")] -> w230
                  tunnel: [w234 w237] -> w231
                  tunnel: w232 -> [w234 w237]
                  tunnel: w228 -> [w233 _]
                  frame False {
                  }
                  frame True {
                    w236 = Action_Control_1."pH Calibration Zero"  # Event
                  }
                }
              }
              event "Create Excel Files": Value Change {
                n120 = event-data() -> ()  [unwired: 1 in, 6 out]
                n121 = case shown="True" "Create Excel Files" {
                  selector: "Create Excel Files" -> [w243 _]
                  tunnel: [w243 TRUE] -> w240
                  tunnel: [w242 w244] -> w239
                  frame False {
                    w242 = Action_Control_1."TimeOut"  # Event
                  }
                  frame True {
                    w244 = Action_Control_1."Create Excel Files"  # Event
                  }
                }
              }
              event "Record pH Calibration Reference": Value Change {
                n122 = event-data() -> ()  [unwired: 1 in, 6 out]
                n123 = case shown="True" "Record pH Calibration Reference" {
                  tunnel: [w252 w255] -> w248
                  tunnel: [FALSE FALSE ("Boolean")] -> w249
                  tunnel: [w253 w256] -> w250
                  tunnel: w251 -> [w253 w256]
                  tunnel: w247 -> [w252 _]
                  frame False {
                  }
                  frame True {
                    w255 = Action_Control_1."pH Calibration Standard"  # Event
                  }
                }
              }
              event "Record ORP Calibration": Value Change {
                n124 = event-data() -> ()  [unwired: 1 in, 6 out]
                n125 = case shown="True" "Record ORP Calibration" {
                  tunnel: [w264 w267] -> w260
                  tunnel: [FALSE FALSE ("Boolean")] -> w261
                  tunnel: [w265 w268] -> w262
                  tunnel: w263 -> [w265 w268]
                  tunnel: w259 -> [w264 _]
                  frame False {
                  }
                  frame True {
                    w267 = Action_Control_1."ORP Calibration Standard"  # Event
                  }
                }
              }
              event "Record Salinity Calibration": Value Change {
                n126 = event-data() -> ()  [unwired: 1 in, 6 out]
                n127 = case shown="True" "Record Salinity Calibration" {
                  tunnel: [w276 w279] -> w272
                  tunnel: [FALSE FALSE ("Boolean")] -> w273
                  tunnel: [w277 w280] -> w274
                  tunnel: w275 -> [w277 w280]
                  tunnel: w271 -> [w276 _]
                  frame False {
                  }
                  frame True {
                    w279 = Action_Control_1."Salinity Calibration Standard"  # Event
                  }
                }
              }
              event "Record DO Calibration": Value Change {
                n128 = event-data() -> ()  [unwired: 1 in, 6 out]
                n129 = case shown="True" "Record DO Calibration" {
                  tunnel: [w288 w291] -> w284
                  tunnel: [FALSE FALSE ("Boolean")] -> w285
                  tunnel: [w289 w292] -> w286
                  tunnel: w287 -> [w289 w292]
                  tunnel: w283 -> [w288 _]
                  frame False {
                  }
                  frame True {
                    w291 = Action_Control_1."DO Calibration Standard"  # Event
                  }
                }
              }
              event "Record  SC Calibration": Value Change {
                n130 = event-data() -> ()  [unwired: 1 in, 6 out]
                n131 = case shown="True" "Record  SC Calibration" {
                  tunnel: [w300 w303] -> w296
                  tunnel: [FALSE FALSE ("Boolean")] -> w297
                  tunnel: [w301 w304] -> w298
                  tunnel: w299 -> [w301 w304]
                  tunnel: w295 -> [w300 _]
                  frame False {
                  }
                  frame True {
                    w303 = Action_Control_1."SC Calibration Standard"  # Event
                  }
                }
              }
              event "Increment Depth": Value Change {
                n132 = event-data() -> ()  [unwired: 1 in, 6 out]
                n133 = case shown="True" "Increment Depth" {
                  tunnel: [w312 w315] -> w308
                  tunnel: [FALSE FALSE ("Boolean")] -> w309
                  tunnel: [w313 w316] -> w310
                  tunnel: w311 -> [w313 w316]
                  tunnel: w307 -> [w312 _]
                  frame False {
                  }
                  frame True {
                    w315 = Action_Control_1."Increment Depth Manually"  # Event
                  }
                }
              }
              event "Record Single Sample": Value Change {
                n134 = event-data() -> ()  [unwired: 1 in, 6 out]
                n135 = case shown="True" "Record Single Sample" {
                  tunnel: [w322 w324] -> w321
                  tunnel: [FALSE FALSE] -> w320
                  tunnel: w319 -> [w322 _]
                  frame False {
                  }
                  frame True {
                    w324 = Action_Control_1."Acq. Single Sonde Point"  # Event
                  }
                }
              }
              event "Write Data to Spreadsheet": Value Change {
                n136 = event-data() -> ("OldVal"=w330:bool, "NewVal"=w333:bool)  [unwired: 1 in, 4 out]
                n137 = Not(x=w330) -> (.not. x?=w329:bool)
                n138 = And(x=w329, y=w333) -> (x .and. y?=w327:bool)
                n139 = case shown="True" w327 {
                  tunnel: [w334 w337] -> w332
                  tunnel: [FALSE FALSE ("Boolean")] -> w331
                  tunnel: [w335 w338] -> _
                  tunnel: w328 -> [w335 w338]
                  tunnel: w326 -> [w334 _]
                  frame False {
                  }
                  frame True {
                    w337 = Action_Control_1."Write Sonde Sample Sheet"  # Event
                  }
                }
              }
              event "Sample Not Collected": Value Change {
                n140 = event-data() -> ("NewVal"=w341:bool)  [unwired: 1 in, 5 out]
                n141 = case shown="True" w341 {
                  tunnel: [FALSE FALSE] -> w343
                  tunnel: [w344 w346] -> w342
                  tunnel: w340 -> [_ w346]
                  frame True {
                    w344 = Action_Control_1."Sample Not Collected"  # Event
                  }
                  frame False {
                  }
                }
              }
              event "Record  Sonde Reason": Value Change {
                n142 = event-data() -> ("NewVal"=w349:bool)  [unwired: 1 in, 5 out]
                n143 = case shown="True" w349 {
                  tunnel: [FALSE FALSE] -> w351
                  tunnel: [w352 w354] -> w350
                  tunnel: w348 -> [_ w354]
                  frame True {
                    w352 = Action_Control_1."Record Sonde Reason"  # Event
                  }
                  frame False {
                  }
                }
              }
              event "Start KPRO": Value Change {
                n144 = event-data() -> ()  [unwired: 1 in, 6 out]
                n145 = case shown="True" "Start KPRO" {
                  tunnel: [FALSE FALSE] -> w359
                  tunnel: [w361 w363] -> w358
                  tunnel: w357 -> [_ w363]
                  frame True {
                    w361 = Action_Control_1."Start KPRO Measurements"  # Event
                    n146 = local write "KPRO Finish\nIndicator"(FALSE ("KPRO Finish\nIndicator")) -> ()
                  }
                  frame False {
                  }
                }
              }
              event "Update Depth": Value Change {
                n147 = event-data() -> ()  [unwired: 1 in, 6 out]
                n148 = case shown="True" "Update Depth" {
                  tunnel: [FALSE FALSE] -> w367
                  tunnel: [w369 w371] -> w366
                  tunnel: w365 -> [_ w371]
                  frame True {
                    w369 = Action_Control_1."Update Depth"  # Event
                  }
                  frame False {
                  }
                }
              }
              event "Record IK Reason": Value Change {
                n149 = event-data() -> ()  [unwired: 1 in, 6 out]
                n150 = case shown="True" "Record IK Reason" {
                  tunnel: [FALSE FALSE] -> w376
                  tunnel: [w377 w379] -> w375
                  tunnel: w374 -> [_ w379]
                  frame True {
                    w377 = Action_Control_1."Record IK Reason"  # Event
                  }
                  frame False {
                  }
                }
              }
              event "Finish Tests": Value Change {
                n151 = event-data() -> ()  [unwired: 1 in, 6 out]
                n152 = case shown="True" "Finish Tests" {
                  tunnel: [FALSE FALSE] -> w384
                  tunnel: [w386 w388] -> w383
                  tunnel: w382 -> [_ w388]
                  frame True {
                    w386 = Action_Control_1."Finish KPRO Measurements"  # Event
                    "KPRO Finish\nIndicator" <- TRUE ("KPRO Finish\nIndicator")
                  }
                  frame False {
                  }
                }
              }
              event "Depth mode": Value Change {
                n153 = event-data() -> ()  [unwired: 1 in, 6 out]
                n154 = case shown="True" "Depth mode" {
                  tunnel: [FALSE ("Read String Pot") TRUE ("Read String Pot")] -> w390
                  frame False {
                  }
                  frame True {
                  }
                }
                n155 = local write "Read String Pot"(w390) -> ()
              }
            }
          }
          frame True {
          }
        }
        "Stop" <- w194
        n156 = local read "Stop"() -> (w195:bool)
        n157 = Or(x=w195, y=w194) -> ()  [unwired: 1 out]
        n158 = call <extravilib>:"Write With Abort.vi"("abort"=FALSE, "last element? (F)"=w194, "element"=w192) -> ("channel"=w198:T25)  [unwired: 6 in, 2 out]
        "producer loop" <- w196
      }
    }
  }
  n159 = flat-sequence {
    tunnel: [w421] -> w16
    tunnel: w13 -> [w420]
    tunnel: w12 -> [w396]
    tunnel: w11 -> [w418]
    tunnel: w10 -> [w416]
    tunnel: w9 -> [w415]
    tunnel: w8 -> [w413]
    tunnel: w6 -> [w412]
    tunnel: w4 -> [w411]
    tunnel: w3 -> [w409]
    tunnel: w2 -> [w408]
    tunnel: w1 -> [w407]
    frame #0 {
      w397 = dbl[][] []  # Cumulative Data over 1 string pot
      w398 = dbl[][] []  # Cumulative Sonde  Data Out
      w401 = T6 {"SC Initial "=0.0, "DO Initial "=0.0, "pH Initial  "=0.0, "ORP  Initial"=0.0, "Temp Initial"=0.0, "Salinity Initial "=0.0}  # Sonde Parameters  Initial Values
      w402 = FALSE  # Read String Pot
      w403 = T17 {"Flow"=0.21081600494384767, "Zeroed \nPressure"=74.74207969932556, "Ik"=0.003788962123473114, "Current Depth"=-100.6, "Feet of Stainless"=40, "Start Depth"=0.0, "Abs Start Depth"=0.0}  # Input Depths  and Parameters Cluster
      w404 = T18 {"Absolute Depth In"=0.0, "Current Absolute Depth"=0.0, "First Absolute Depth"=0.0, "Previous Relative Depth"=0.0, "Current Relative Depth"=0.0, "First Relative Depth"=0.0, "Last Filed Depth"=0.0, "Total Volume In"=0.0, "Total Volume Out"=0.0, "Current Measurement Time"=0.0, "Previous Measurement Time"=0.0}  # Depth Cluster
      w405 = dbl[][] []  # Cumulative Data From File
      w406 = dbl[] []  # Time Array
      w414 = cluster{"row":i32, "column":i32} {"row"=0, "column"=0}  # start of last occupied row
      w417 = 0  # row index
      n160 = Get Date/Time In Seconds() -> (seconds since 1Jan1904=w400:timestamp)
      n161 = To Double Precision Float(number=w400) -> (double precision float=w399:dbl)
      n162 = while {
        tunnel: w420 -> [w473]
        tunnel: [w474] -> w421
        tunnel: w411 -> [w451]
        shift-right: [w464] -> _
        shift-left: "Current Sheet" -> [w425]
        tunnel: w418 -> [w466]
        tunnel: w416 -> [w472]
        tunnel: w415 -> [w471]
        shift-right: [w465] -> _
        shift-left: w417 -> [w470]
        shift-right: [w468] -> _
        shift-left: w414 -> [w467]
        tunnel: w413 -> [w463]
        shift-right: [w457] -> _
        shift-left: w406 -> [w458]
        shift-right: [w456] -> _
        shift-left: w405 -> [w455]
        tunnel: w399 -> [w454]
        tunnel: [w453] -> _
        tunnel: w412 -> [w439]
        shift-right: [w449] -> _
        shift-left: refnum<k24>[] [] -> [w438]
        tunnel: w409 -> [w426]
        shift-right: [w427] -> _
        shift-left: w408 -> [w428]
        shift-right: [w447] -> _
        shift-left: w407 -> [w447]
        shift-right: [w444] -> _
        shift-left: w402 -> [w443]
        shift-right: [w431] -> _
        shift-left: w404 -> [w442]
        shift-right: [w441] -> _
        shift-left: w403 -> [w440]
        shift-right: [w435] -> _
        shift-left: w401 -> [_]
        shift-right: [w433] -> _
        shift-left: w398 -> [w432]
        shift-right: [w430] -> _
        shift-left: w397 -> [w429]
        shift-right: [w469] -> _
        shift-left: w396 -> [w423]
        i -> [w436]
        stop <- w452 stop-if-true
        (unwired) FALSE
        # "Consumer Data Handling Loop"
        n163 = flat-sequence {
          tunnel: [w493] -> w460
          tunnel: [w492] -> w459
          tunnel: w451 -> [w491]
          tunnel: [w490] -> w450
          frame #0 {
            n164 = call <extravilib>:"Read With Abort.vi"("abort"=FALSE, "channel"=w491) -> ("last element?"=w490:bool, "element"=w493:T24)  [unwired: 5 in, 3 out]
            n165 = feedback #1() -> (w492:T24)  [unwired: 1 in]
            n166 = feedback-in #1(w493) -> ()
          }
        }
        n167 = call <userlib>:"Wait (ms)__ogtk.vi"("error in (no error)"=w473, "milliseconds to wait"=u32 50) -> ("error out"=w462:errorcluster)  [unwired: 8 in, 1 out]
        n168 = case shown="False" FALSE {
          tunnel: w466 -> [_ w489]
          tunnel: w463 -> [_ w488]
          tunnel: w462 -> [w477 w487]
          tunnel: [w478 w486] -> w448
          tunnel: [w475 w485] -> w446
          tunnel: w425 -> [w480 w484]
          tunnel: [w481 w483] -> w424
          tunnel: w423 -> [w481 w482]
          frame False {
            n169 = call <vilib>:"Clear Errors.vi"("error in (no error)"=w477) -> ("error out"=w476:errorcluster)  [unwired: 5 in, 1 out]
            n170 = Format Into String(format string="Sample %d", error in=w476, w480) -> (resulting string=w478:string, error out=w475:errorcluster)  [unwired: 1 in]
          }
          frame True {
            n171 = call "open select sample sheet.vi"("Number of Sample Sheets"=w488, "error in (no error)"=w487, "Worksheet Names"=w489, "input 1"=w484, "NI_report in"=w482) -> ("error out"=w485:errorcluster, "Current Sample Sheet"=w486:string, "NI_report out"=w483:refnum<class "NI_report.lvclass">)  [unwired: 4 in]
          }
        }
        n172 = flat-sequence {
          tunnel: w426 -> [w506]
          frame #0 {
            n173 = Get Date/Time In Seconds() -> (seconds since 1Jan1904=w507:timestamp)
            n174 = Subtract(x=w507, y=w506) -> (x-y=w508:dbl)
            n175 = local write "Current Time (s)"(w508) -> ()
          }
        }
        n176 = flat-sequence {
          tunnel: w448 -> [w513]
          tunnel: w446 -> [w510]
          tunnel: [w512] -> w445
          tunnel: w425 -> [w511]
          frame #0 {
            n177 = call <vilib>:"Clear Errors.vi"("error in (no error)"=w510) -> ("error out"=w509:errorcluster)  [unwired: 5 in, 1 out]
            n178 = Format Into String(format string="Data from Sample %d ", error in=w509, w511) -> (resulting string=→"Table Label":string, error out=w512:errorcluster)  [unwired: 1 in]
            "Current Sample Sheet" <- w513
          }
        }
        n179 = flat-sequence {
          tunnel: w439 -> [w498]
          tunnel: w438 -> [w497]
          tunnel: [w496] -> w437
          tunnel: w436 -> [w495]
          frame #0 {
            n180 = case shown="1, Default" w495 {
              tunnel: w497 -> [w499 w505]
              tunnel: w498 -> [_ w504]
              tunnel: [w499 w502] -> w496
              frame 0 {
              }
              frame 1, Default {
                n181 = local read "Descriptions"() -> (w503:string[])
                n182 = call "Measure DAQ Voltages.vi"("error in (no error)"=w504, "Descriptions"=w503, "Array in"=w505) -> ("Raw Voltages"=w501:dbl[], "Array out"=w502:refnum<k24>[], "Sensor Cluster"=w500:T10)  [unwired: 6 in]
                n183 = local write "Sensor Voltage Cluster"(w500) -> ()
                n184 = local write "Raw Voltages"(w501) -> ()
              }
            }
            "consumer loop" <- w495
          }
        }
        n185 = case shown="\"Init\"" w460 {
          selector: w460 -> [_ _ _ _ _ _ _ _ _ _ _ _ _ _ _ _ _ w2117 _ _ _ _]
          tunnel: w445 -> [w529 w684 w728 w771 w794 w927 w1092 w1109 w1145 w1188 w1220 w1337 w1459 w1595 w1731 w1865 w1993 w2123 w2254 w2650 w2661 w2730]
          tunnel: [w529 w684 w728 w771 w790 w926 w1092 w1109 w1145 w1187 w1218 w1335 w1457 w1593 w1729 w1863 w1991 w2107 w2254 w2650 w2674 w2742] -> w474
          tunnel: w450 -> [_ _ _ _ _ _ _ _ _ _ _ _ _ _ _ _ _ _ _ _ _ _]
          tunnel: w424 -> [w545 w673 w727 w770 w811 w948 w1091 w1108 w1144 w1182 w1227 w1352 w1473 w1609 w1745 w1878 w2006 w2124 w2261 w2649 w2660 _]
          tunnel: [w544 w683 w726 w769 w810 w947 w1090 w1107 w1143 w1181 w1216 w1332 w1454 w1590 w1726 w1860 w1988 w2112 w2260 w2648 w2679 w2747] -> w465
          tunnel: w472 -> [_ _ _ _ _ _ _ _ _ _ w1225 w1350 w1471 w1607 w1743 w1876 w2004 _ _ _ _ _]
          tunnel: w471 -> [_ _ _ _ _ _ _ _ _ _ w1224 w1349 w1470 w1606 w1742 w1875 w2003 _ _ _ _ _]
          tunnel: w470 -> [w544 w683 w726 w769 w810 w947 w1090 w1107 w1143 w1181 w1192 w1333 w1455 w1591 w1727 w1861 w1989 w2101 w2260 w2648 w2679 w2747]
          tunnel: [w545 w673 w727 w770 w811 w948 w1091 w1108 w1144 w1182 w1221 w1338 w1460 w1596 w1732 w1866 w1994 w2122 w2261 w2649 w2680 w2748] -> w469
          tunnel: w425 -> [w543 w682 w725 w768 w798 w932 w1089 w1106 w1142 w1180 w1202 w1346 w1467 w1603 w1739 w1872 w2000 w2119 w2259 w2647 w2678 w2746]
          tunnel: [w543 w682 w725 w768 w798 w932 w1089 w1106 w1142 w1180 w1202 w1346 w1467 w1603 w1739 w1872 w2000 w2118 w2259 w2647 w2678 w2746] -> w464
          tunnel: [w542 w681 w724 w767 w809 w946 w1088 w1105 w1141 w1179 w1217 w1334 w1456 w1592 w1728 w1862 w1990 w2115 w2258 w2646 w2677 w2745] -> w468
          tunnel: w467 -> [w542 w681 w724 w767 w809 w946 w1088 w1105 w1141 w1179 w1194 w1314 w1436 w1570 w1706 w1842 w1970 w2098 w2258 w2646 w2677 w2745]
          tunnel: w466 -> [_ _ _ _ _ _ _ _ _ _ _ _ _ _ _ _ _ w2121 _ _ _ _]
          tunnel: w463 -> [_ _ _ _ _ _ _ _ _ _ _ _ _ _ _ _ _ w2120 _ _ _ _]
          tunnel: w459 -> [_ _ _ _ _ _ _ _ _ _ _ _ _ _ _ _ _ w2116 _ _ _ _]
          tunnel: w458 -> [w528 w680 w723 w766 w808 w945 w1087 w1104 w1140 w1178 w1215 w1331 w1453 w1589 w1725 w1859 w1987 w2111 w2257 w2645 w2676 w2744]
          tunnel: [w527 w680 w723 w766 w808 w945 w1087 w1104 w1140 w1178 w1214 w1330 w1452 w1588 w1724 w1858 w1986 w2111 w2257 w2645 w2676 w2744] -> w457
          tunnel: [w522 w674 w722 w765 w796 w930 w1086 w1103 w1139 w1177 w1213 w1329 w1451 w1578 w1723 w1857 w1985 w2110 w2246 w2644 w2675 w2743] -> w456
          tunnel: w455 -> [w523 w674 w722 w765 w802 w937 w1086 w1103 w1139 w1177 w1212 w1328 w1450 w1578 w1722 w1856 w1984 w2110 w2247 w2644 w2675 w2743]
          tunnel: w454 -> [_ _ _ _ _ _ _ _ _ _ w1201 w1327 w1449 w1587 w1721 w1855 w1983 _ _ _ _ _]
          tunnel: w437 -> [w537 w679 w721 w764 w805 w942 w1085 w1102 w1138 w1176 w1210 w1325 w1447 w1585 w1719 w1853 w1981 w2109 _ w2642 w2669 w2739]
          tunnel: [w541 w678 w720 w763 w784 w925 w1084 w1093 w1137 w1175 w1211 w1326 w1448 w1586 w1720 w1854 w1982 w2108 w2253 _ w2670 w2740] -> w453
          tunnel: w439 -> [w541 w678 w720 w763 w785 w925 w1084 w1094 w1137 w1175 w1211 w1326 w1448 w1586 w1720 w1854 w1982 w2108 w2255 w2641 w2673 w2731]
          tunnel: [_ _ _ _ _ _ _ _ _ _ _ _ _ _ _ _ _ _ FALSE ("aborted?") FALSE ("aborted?") w2672 w2741] -> w452
          tunnel: [w533 w679 w721 w764 w805 w942 w1085 w1102 w1138 w1176 w1210 w1325 w1447 w1585 w1719 w1853 w1981 w2109 w2244 w2640 w2669 w2739] -> w449
          tunnel: [w540 w677 w719 w762 w807 w944 w1083 w1101 w1136 w1174 w1208 w1323 w1445 w1583 w1717 w1851 w1979 w2106 "Read String Pot" w2639 w2668 w2738] -> w444
          tunnel: w443 -> [w540 w677 w719 w762 w807 w944 w1083 w1101 w1136 w1174 w1208 w1323 w1445 w1583 w1717 w1851 w1979 w2106 _ w2639 w2668 w2738]
          tunnel: [w520 w667 w714 w758 w800 w934 w1082 w1100 w1135 w1173 w1207 w1322 w1444 w1582 w1716 w1850 w1978 w2105 w2250 w2638 w2667 w2737] -> w431
          tunnel: w442 -> [w521 w667 w715 w758 w777 w935 w1082 w1100 w1135 w1173 w1207 w1322 w1444 w1582 w1716 w1850 w1978 w2105 w2236 w2638 w2667 w2737]
          tunnel: [w539 w676 w718 w761 w806 w943 w1081 w1099 w1134 w1172 w1206 w1321 w1443 w1581 w1715 w1849 w1977 w2104 w2249 w2637 w2666 w2736] -> w441
          tunnel: w440 -> [w539 w676 w718 w761 w806 w943 w1081 w1099 w1134 w1172 w1206 w1321 w1443 w1581 w1715 w1849 w1977 w2104 _ w2637 w2666 w2736]
          tunnel: [w538 w675 w717 w760 w795 w929 w1080 w1098 w1133 w1171 w1199 w1320 w1442 w1580 w1714 w1848 w1976 w2103 w2240 w2636 w2665 w2735] -> w435
          tunnel: "Sonde Parameters \nInitial Values" -> [w538 w675 w717 w760 w795 w929 w1080 w1098 w1133 w1171 w1204 w1320 w1442 w1580 w1714 w1848 w1976 w2103 w2240 w2636 w2665 w2735]
          tunnel: w428 -> [w517 w669 w716 w759 w793 w919 w1079 w1097 w1132 w1170 w1203 w1319 w1441 w1579 w1713 w1847 w1975 w2102 w2239 w2635 w2664 w2734]
          tunnel: [w516 w668 w716 w759 w772 w920 w1079 w1097 w1132 w1170 w1203 w1319 w1441 w1579 w1713 w1847 w1975 w2102 w2239 w2635 w2664 w2734] -> w427
          tunnel: [w526 w672 w713 w757 w778 w923 w1078 w1096 w1131 w1169 w1200 w1318 w1440 w1577 w1712 w1846 w1974 w2100 w2237 w2634 w2663 w2733] -> w433
          tunnel: w432 -> [w525 w672 w713 w757 w778 w923 w1078 w1096 w1131 w1169 w1200 w1318 w1440 w1576 w1712 w1846 w1974 w2100 w2237 w2634 w2663 w2733]
          tunnel: [w518 w671 w712 w756 w774 w922 w1077 w1095 w1130 w1168 w1198 w1317 w1439 w1575 w1711 w1845 w1973 w2099 w2234 w2633 w2662 w2732] -> w430
          tunnel: w429 -> [w519 w671 w712 w756 w775 w921 w1077 w1095 w1130 w1168 w1198 w1317 w1439 w1575 w1711 w1845 w1973 w2099 w2234 w2633 w2662 w2732]
          frame "TimeOut", Default {
            n186 = flat-sequence {
              tunnel: [w654] -> _
              tunnel: [w658] -> w530
              tunnel: [w666] -> _
              tunnel: [w665] -> _
              tunnel: w537 -> [w664]
              tunnel: [w663] -> _
              frame #0 {
                n187 = local read "Input Variables and Slopes"() -> (w656:T1)
                n188 = local read "Input Variables and Slopes"() -> (w660:T1)
                n189 = local read "Sample Sheet Data Row Cluster 2"() -> (w653:T2)
                n190 = local read "Zero In-Line Pressure\n(F = leave as is)"() -> (w659:bool)
                n191 = Unbundle By Name(w660) -> ("DH Pressure Trans Slope"=w666:dbl, "DH Pressure Offset"=w665:dbl)
                n192 = local read "Sensor Voltage Cluster"() -> (w661:T10)
                n193 = local read "Descriptions"() -> (w662:string[])
                n194 = local read "Sensor  Real \nMeasurements"() -> (w657:T7)
                n195 = global read "Kpro Globals.vi" "Current Depth"() -> (w654:sgl)
                n196 = call "DHT Pressure 2016.vi"("Sensor Cluster"=w661, "DHT Pressure Offset"=w665, "Array in"=w664, "DHT Pressure \nSlope"=w666, "Descriptions"=w662, "Zero Pressure\n(F = leave as is)"=w659) -> ("Array out"=w663:refnum<k24>[], "DHT Pressure"=w658:dbl, "Sensor Cluster 2"=w655:T10)  [unwired: 7 in]
                n197 = local write "Sensor Voltage Cluster"(w655) -> ()
                n198 = call "convert sensor voltage to real measurements.vi"("Input Variables and Slopes"=w656, "Sensor  Real Measurements in"=w657, "Sensor Cluster"=w655) -> ("Sensor  Real Measurements out"=w651:T10)  [unwired: 8 in]
                n199 = Unbundle By Name(w651) -> ("Aux 1"=w650:dbl, "Aux 2"=w649:dbl, "Aux 3"=w648:dbl)
                n200 = Bundle By Name(cluster=w653, "Aux1"=w650, "Aux2"=w649, "Aux3"=w648) -> (w652:T2)
                n201 = local write "Sensor  Real \nMeasurements"(w651) -> ()
                n202 = local write "Down hole Pressure"(w658) -> ()
                n203 = local write "Sample Sheet Data Row Cluster 2"(w652) -> ()
                n204 = Add(x=w658, y=w654) -> ()  [unwired: 1 out]
              }
            }
            n205 = case shown="True" "Update Sonde" {
              tunnel: w528 -> [w547 w554]
              tunnel: [w547 w553] -> w527
              tunnel: [w546 w552] -> w526
              tunnel: w525 -> [w546 w551]
              frame False {
              }
              frame True {
                n206 = local read "Sonde Communication Error Out"() -> (w550:errorcluster)
                n207 = local read "Current Time (s)"() -> (w548:dbl)
                n208 = flat-sequence {
                  tunnel: w550 -> [w572]
                  tunnel: [w571] -> w549
                  tunnel: w554 -> [w570]
                  tunnel: [w569] -> w553
                  tunnel: [w568] -> w552
                  tunnel: w551 -> [w567]
                  tunnel: [w557] -> _
                  tunnel: [w566] -> _
                  tunnel: w548 -> [w565]
                  frame #0 {
                    n209 = local read "Sample Sheet Data Row Cluster 2"() -> (w558:T2)
                    n210 = control-ref of="Found Quanta Sonde Com Port"() -> (w564:refnum<vi>)
                    n211 = control-ref of="Current Time (s)"() -> (w560:refnum<vi>)
                    n212 = control-ref of="Temperature"() -> (w561:refnum<vi>)
                    n213 = control-ref of="Sonde Data Display"() -> (w563:refnum<vi>)
                    n214 = control-ref of="Sonde Data Display"() -> (w562:refnum<vi>)
                    n215 = Unbundle By Name(w558) -> ("Sonde Data Cluster.Cumulative\nVolume (ml)"=w555:dbl)
                    n216 = call "Sonde Single Measurement Subvi.vi"("VISAResourceName in"=w564, "Time Array"=w570, "Cumulative Sonde Data"=w567, "Previous time"=w565, "Sonde Data Display"=w563, "Sonde Graph in"=w562, "Temp Graph 3"=w561, "error in (no error)"=w572, "Row Cluster Input"=w558, "reference 5"=w560) -> ("seconds since 1Jan1904"=w566:timestamp, "Cumulative Sonde \nData Out"=w568:dbl[][], "Sample Sheet Data Row Cluster 2"=w557:T2, "output cluster"=w559:T3, "time array out"=w569:dbl[], "error out"=w571:errorcluster)
                    n217 = Bundle By Name(cluster=w557, "Sonde Data Cluster.Cumulative\nVolume (ml)"=w555) -> (w556:T2)
                    n218 = local write "Sample Sheet Data Row Cluster 2"(w556) -> ()
                    n219 = local write "output cluster"(w559) -> ()
                  }
                }
                n220 = local write "Sonde Communication Error Out"(w549) -> ()
              }
            }
            n221 = flat-sequence {
              tunnel: w537 -> [w642]
              tunnel: [w638] -> w536
              tunnel: [w637] -> w535
              frame #0 {
                n222 = local read "Input Variables and Slopes"() -> (w645:T1)
                n223 = Unbundle By Name(w645) -> ("Up Hole Pressure Slope"=w644:dbl, "Up Hole  Pressure Offset"=w641:dbl)
                n224 = local write "Input Variables and Slopes"(w645) -> ()
                n225 = local read "Sensor Voltage Cluster"() -> (w646:T10)
                n226 = local read "Descriptions"() -> (w638:string[])
                n227 = local read "Corrected\n Pressure \nCluster"() -> (w640:T21)
                n228 = call "up hole Pressure 2016.vi"("Sensor Cluster"=w646, "Pressure Offset"=w641, "Array in"=w642, "Pressure \nSlope"=w644, "Descriptions"=w638, "Zero Pressure\n(F = leave as is)"=TRUE) -> ("Array out"=w637:refnum<k24>[], "Uphole Pressure"=w636:dbl, "Sensor Cluster 2"=w643:T10)  [unwired: 6 in, 1 out]
                n229 = local write "Uphole Pressure"(w636) -> ()
                n230 = Bundle By Name(cluster=w640, "Up hole Corrected Pressure"=w636) -> (w639:T21)
                n231 = local write "Sensor Voltage Cluster"(w643) -> ()
                n232 = local write "Corrected\n Pressure \nCluster"(w639) -> ()
              }
            }
            n233 = flat-sequence {
              tunnel: w536 -> [w629]
              tunnel: w535 -> [w632]
              tunnel: [w628] -> w532
              tunnel: [w629] -> w534
              tunnel: [w625] -> w531
              tunnel: [w627] -> w533
              frame #0 {
                w633 = 0.0  # Offset
                n234 = local read "Input Variables and Slopes"() -> (w631:T1)
                n235 = local read "Input Depths \nand Parameters Cluster"() -> (w624:T17)
                n236 = Unbundle By Name(w631) -> ("Flow Slope"=w630:dbl)
                n237 = local read "Input Depths \nand Parameters Cluster"() -> (w635:T17)
                n238 = Unbundle By Name(w624) -> ("Feet of Stainless"=w623:i32)
                n239 = call "Flow 2016.vi"("Descriptions"=w629, "Array in"=w632, "Flow Slope"=w630, "Offset"=w633) -> ("Sensor Cluster"=w628:T10, "Flow (ml/min)"=w625:dbl, "Array out"=w627:refnum<k24>[])  [unwired: 4 in]
                n240 = local write "Sensor Voltage Cluster"(w628) -> ()
                n241 = call "pressure and IK2 2016.vi"("Ft. of SS"=w623, "flow"=w625) -> ("IK"=→"Large Depth IK Graph":dbl)  [unwired: 1 in, 1 out]
                n242 = Bundle By Name(cluster=w635, "Flow"=w625) -> (w634:T17)
                n243 = local write "Input Depths \nand Parameters Cluster"(w634) -> ()
              }
            }
            n244 = flat-sequence {
              tunnel: w534 -> [w611]
              tunnel: w523 -> [w589]
              tunnel: w532 -> [w610]
              tunnel: w521 -> [w594]
              tunnel: [w609] -> w520
              tunnel: w531 -> [w608]
              tunnel: w533 -> [w602]
              tunnel: [w601] -> _
              tunnel: [w581] -> w522
              tunnel: [w595] -> _
              tunnel: w530 -> [w586]
              tunnel: w529 -> [w583]
              tunnel: w519 -> [w582]
              tunnel: [w579] -> w518
              tunnel: w517 -> [w575]
              tunnel: [w574] -> w516
              frame #0 {
                # "Timeout"
                n245 = Unbundle By Name(w594) -> ("Current Relative Depth"=w593:dbl)
                n246 = local read "Input Depths \nand Parameters Cluster"() -> (w605:T17)
                n247 = local read "Culmulative Graph Cluster"() -> (w600:T20)
                n248 = local read "Depth mode"() -> (w591:bool)
                n249 = local read "Input Variables and Slopes"() -> (w607:T1)
                n250 = local read "KPRO Finish\nIndicator"() -> (w588:bool)
                n251 = local read "KPRO SessionOutput File Path"() -> (w595:path)
                n252 = Unbundle By Name(w607) -> ("String Pot Slope"=w606:dbl)
                n253 = Unbundle By Name(w605) -> ()  [unwired: 1 out]
                n254 = local read "Uphole Pressure"() -> (w576:dbl)
                n255 = call "Kpro Read String Pot 2016.vi"("Read String Pot"=w591, "Feet of\nStainless to be\nUsed (Count) in"=w575, "Session Array in"=w582, "Flow"=w608, "Manual Depth In"=w593, "Finished In"=w588, "Depth Cluster in"=w594, "error in (no error)"=w583, "String Pot \nSlope in"=w606, "Sensor Cluster In in"=w610, "Descriptions"=w611, "Pressure in"=w576, "Array in"=w602, "Downhole Pressure Sensor"=w586, "Initial Measurement Input"=FALSE) -> ("Sensor Cluster 2"=w603:T10, "IK"=w585:dbl, "Array out"=w601:refnum<k24>[], "Generate Array Calc IK"=w590:bool, "Feet of\nStainless to be\nUsed (Count) out"=w574:i32, "Depth Cluster out"=w609:T18, "Single String Pot Session Array out"=w579:dbl[][])  [unwired: 4 in, 2 out]
                n256 = local write "Ik"(w585) -> ()
                n257 = local write "Sensor Voltage Cluster"(w603) -> ()
                n258 = Unbundle By Name(w609) -> ("Current Absolute Depth"=w592:dbl)
                n259 = And(x=w590, y=w591) -> ()  [unwired: 1 out]
                n260 = Bundle By Name(cluster=w605, "Feet of Stainless"=w574) -> (w604:T17)
                n261 = local write "Input Depths \nand Parameters Cluster"(w604) -> ()
                n262 = flat-sequence {
                  tunnel: w592 -> [w617]
                  frame #0 {
                    n263 = global write "Kpro Globals.vi" "Current Depth"(w617) -> ()
                    n264 = local write "Current Depth"(w617) -> ()
                    n265 = Divide(x=w617, y=3.281) -> (x/y=w618:dbl)
                    n266 = local read "Sample Sheet Data Row Cluster 2"() -> (w621:T2)
                    n267 = local read "Corrected\n Pressure \nCluster"() -> (w619:T21)
                    n268 = Unbundle By Name(w619) -> ("Up hole Corrected Pressure"=w616:dbl)
                    "Uphole Pressure" <- w616
                    n269 = Bundle By Name(cluster=w621, "Depth"=w617, "Head\nPressure"=w616) -> (w620:T2)
                    n270 = local write "Sample Sheet Data Row Cluster 2"(w620) -> ()
                    n271 = local write "Current \nDepth (m)"(w618) -> ()
                  }
                }
                n272 = case shown="True" FALSE {
                  tunnel: w589 -> [w612 w615]
                  tunnel: w579 -> [_ w613]
                  tunnel: [w612 w614] -> w581
                  frame False {
                  }
                  frame True {
                    n273 = Build Array (concatenate)(w615, w613) -> (w614:dbl[][])
                  }
                }
                n274 = call "Array to Plot 2016.vi"("Input Cumulative Array"=w581, "Input Real Time Array"=w579) -> ("Cumulative - Depth vs.Drive Rate"=w577:cluster{dbl[], dbl[]}, "Cumulative - Depth vs. Ik"=w598:cluster{dbl[], dbl[]}, "Real Time - Depth vs. Drive Rate"=w578:cluster{dbl[], dbl[]}, "Real Time - Depth vs. Ik"=w587:cluster{dbl[], dbl[]}, "Depth Rate"=w584:dbl)  [unwired: 2 in, 1 out]
                n275 = Bundle By Name(cluster=w600, "Cumulative - Depth vs. Ik"=w598, "Real Time - Depth vs. lk"=w587, "Cumulative - Depth vs. Drive Rate"=w577, "Real Time - Depth vs. Drive Rate"=w578) -> (w599:T20)
                n276 = local write "Large Depth IK Graph Cluster"(w587) -> ()
                n277 = local write "Culmulative Graph Cluster"(w599) -> ()
                n278 = local write "Depth Rate\nft/min"(w584) -> ()
                n279 = local write "Current Session"(w579) -> ()
                n280 = local read "Input Depths \nand Parameters Cluster"() -> (w597:T17)
                n281 = local write "Cumulative_data_from_file"(w581) -> ()
                n282 = Unbundle By Name(w597) -> ("Flow"=→"Flow":dbl)
              }
            }
          }
          frame "Finish KPRO Measurements" {
            n283 = flat-sequence {
              tunnel: w667 -> [w693]
              tunnel: [w703] -> w670
              tunnel: w674 -> [w700]
              tunnel: w671 -> [w695]
              tunnel: w669 -> [w694]
              tunnel: [w692] -> _
              tunnel: [w691] -> w668
              frame #0 {
                n284 = local read "Input Depths \nand Parameters Cluster"() -> (w702:T17)
                n285 = local read "KPRO SessionOutput File Path"() -> (w699:path)
                n286 = Unbundle By Name(w702) -> ()  [unwired: 1 out]
                n287 = Build Array (concatenate)(w700, w695) -> (w696:dbl[][])
                n288 = case shown="False" TRUE {
                  tunnel: w699 -> [w704 w711]
                  tunnel: [w704 w706] -> w698
                  frame False {
                  }
                  frame True {
                    n289 = call-poly <vilib>:"Write Delimited Spreadsheet.vi"("file path (dialog if empty)"=w711, "1D data"="KPRO test report header", "append to file? (new file:F)"=FALSE, "error in (no error)"=errorcluster {"status"=FALSE, "code"=0, "source"=""} ("error constant"), "transpose? (no:F)"=FALSE, "delimiter (\\t)"="," ("delimiter (\\t)")) -> ("new file path (Not A Path if cancelled)"=w706:path)  [unwired: 8 in, 1 out]
                  }
                }
                n290 = call "Finished Collection Write File.vi"("Cluster in"=w693, "Corrected Array in"=w696, "Feet of\nStainless to be\nUsed (Count) in"=w694, "Output KPRO"=w698) -> ("Corrected Array out"=w703:dbl[][], "Depth to \nbe Used \n(Feet)"=w692:sgl, "Feet of\nStainless to be\nUsed (Count) out"=w691:i32)  [unwired: 5 in]
                n291 = Bundle By Name(cluster=w702, "Feet of Stainless"=w691) -> (w701:T17)
                n292 = local write "Current Depth"(w692) -> ()
                n293 = local write "Input Depths \nand Parameters Cluster"(w701) -> ()
              }
            }
            n294 = flat-sequence {
              tunnel: w670 -> [w689]
              frame #0 {
                n295 = control-ref of="KPRO SessionOutput File Path"() -> (w687:refnum<vi>)
                n296 = call "write KPRO file.vi"("Corrected Array in"=w689, "Generate Array Calc IK"=TRUE, "Path in"=w687) -> ("paths ok"=w686:bool, "appended path"=w685:path)  [unwired: 7 in]
                n297 = case shown="True" w686 {
                  tunnel: w685 -> [_ w690]
                  frame False {
                  }
                  frame True {
                    n298 = local write "KPRO SessionOutput File Path"(w690) -> ()
                  }
                }
              }
            }
          }
          frame "Update Depth" {
            n299 = flat-sequence {
              tunnel: w715 -> [w740]
              tunnel: [w737] -> w714
              frame #0 {
                n300 = Unbundle By Name(w740) -> ("First Absolute Depth"=w738:dbl)
                n301 = local read "Current Depth"() -> (w734:sgl)
                n302 = local read "Sensor  Real \nMeasurements"() -> (w741:T7)
                n303 = Greater?(x="New Depth", y=w734) -> (0:w733:bool)
                n304 = case shown="False" w733 {
                  tunnel: [w750 w755] -> w739
                  tunnel: w738 -> [w749 w754]
                  tunnel: "New Depth" -> [w747 w752]
                  tunnel: w734 -> [w746 w751]
                  frame True {
                    n305 = Subtract(x=w746, y=w747) -> (x-y=w748:dbl)
                    n306 = Subtract(x=w749, y=w748) -> (x-y=w750:dbl)
                  }
                  frame False {
                    # "Reverse inputs \non Subtraction"
                    n307 = Subtract(x=w752, y=w751) -> (x-y=w753:dbl)
                    n308 = Subtract(x=w754, y=w753) -> (x-y=w755:dbl)
                  }
                }
                n309 = Unbundle By Name(w741) -> ("String Pot"=w730:dbl)
                n310 = Bundle By Name(cluster=w740, "Absolute Depth In"="New Depth", "Current Absolute Depth"="New Depth", "First Absolute Depth"=w739) -> (w732:T18)
                n311 = local read "Read String Pot"() -> (w729:bool)
                n312 = case shown="False" w729 {
                  tunnel: w732 -> [w742 w745]
                  tunnel: [w742 w744] -> w731
                  tunnel: w730 -> [_ w743]
                  frame False {
                  }
                  frame True {
                    n313 = Bundle By Name(cluster=w745, "Current Relative Depth"=w743) -> (w744:T18)
                  }
                }
                n314 = call "calculate current depth.vi"("Cluster in"=w731) -> ("Cluster out"=w737:T18)  [unwired: 10 in]
                n315 = Unbundle By Name(w737) -> ("Current Absolute Depth"=w736:dbl)
                n316 = local write "Current Depth"(w736) -> ()
                n317 = global write "Kpro Globals.vi" "Current Depth"(w736) -> ()
              }
            }
          }
          frame "IK vs Time" {
          }
          frame "Start KPRO Measurements" {
            n318 = flat-sequence {
              tunnel: w794 -> [w822]
              tunnel: w793 -> [w821]
              tunnel: [w820] -> w792
              tunnel: [w819] -> w791
              tunnel: [w816] -> w773
              frame #0 {
                n319 = local read "Input Variables and Slopes"() -> (w814:T1)
                n320 = Unbundle By Name(w814) -> ("Depth to Water Table"=w815:dbl)
                n321 = local read "Input Depths \nand Parameters Cluster"() -> (w818:T17)
                n322 = call <vilib>:"Clear Errors.vi"("error in (no error)"=w822) -> ("error out"=w812:errorcluster)  [unwired: 5 in, 1 out]
                n323 = call "New Stainless Correction Pop Up 2016.vi"("error in (no error)"=w812, "New Feet\n of Stainless\n(Count)"=w821, "Depth to \nWater Table\nInput"=w815) -> ("error in (no error) 2"=w819:errorcluster, "Feet of\nStainless to be\nUsed (Count)"=w816:i32, "Depth to \nWater Table\nOutput"=w813:dbl)  [unwired: 6 in]
                n324 = Bundle By Name(cluster=w814, "Depth to Water Table"=w813) -> (w820:T1)
                n325 = Bundle By Name(cluster=w818, "Feet of Stainless"=w816) -> (w817:T17)
                n326 = local write "Input Depths \nand Parameters Cluster"(w817) -> ()
              }
            }
            n327 = flat-sequence {
              tunnel: w805 -> [w849]
              tunnel: [w848] -> w804
              tunnel: w792 -> [w847]
              tunnel: w791 -> [w846]
              tunnel: [w845] -> w790
              tunnel: [w836] -> w789
              frame #0 {
                n328 = control-ref of="Input Variables and Slopes"() -> (w842:refnum<vi>)
                n329 = control-ref of="Sensor Voltage Cluster"() -> (w840:refnum<vi>)
                n330 = control-ref of="Zero In-Line Pressure\n(F = leave as is)"() -> (w839:refnum<vi>)
                n331 = control-ref of="Output File Path"() -> (w843:refnum<vi>)
                n332 = control-ref of="Descriptions"() -> (w841:refnum<vi>)
                n333 = call "measure down hole pressure and save to csv file.vi"("Path in"=w843, "reference 3"=w841, "reference in"=w842, "reference 4"=w840, "reference 5"=w839, "Record DTW File"="Record DTW File", "error in (no error)"=w846, "Array in"=w849, "Input Variables and Slopes"=w847) -> ("Array out"=w848:refnum<k24>[], "In-Line Pressure"=w836:dbl, "error out"=w845:errorcluster)  [unwired: 3 in, 1 out]
                "Down hole Pressure" <- w836
                n334 = local read "Corrected\n Pressure \nCluster"() -> (w838:T21)
                n335 = Bundle By Name(cluster=w838, "Down hole Corrected Pressure"=w836) -> (w837:T21)
                n336 = local write "Corrected\n Pressure \nCluster"(w837) -> ()
                n337 = invoke on="Update Sonde" class="Bool (strict)" method="Reinit To Default"() -> ()  [unwired: 3 in, 3 out]
                n338 = property on="Large Depth IK Graph" class="WFChart (strict)"("History Data"=dbl[] []) -> ()  [unwired: 2 in, 2 out]
              }
            }
            n339 = flat-sequence {
              tunnel: w804 -> [w913]
              tunnel: [w909] -> w788
              tunnel: [w908] -> w787
              frame #0 {
                n340 = local read "Input Variables and Slopes"() -> (w916:T1)
                n341 = Unbundle By Name(w916) -> ("Up Hole Pressure Slope"=w915:dbl, "Up Hole  Pressure Offset"=w912:dbl)
                n342 = local write "Input Variables and Slopes"(w916) -> ()
                n343 = local read "Sensor Voltage Cluster"() -> (w917:T10)
                n344 = local read "Descriptions"() -> (w909:string[])
                n345 = local read "Corrected\n Pressure \nCluster"() -> (w911:T21)
                n346 = call "up hole Pressure 2016.vi"("Sensor Cluster"=w917, "Pressure Offset"=w912, "Array in"=w913, "Pressure \nSlope"=w915, "Descriptions"=w909, "Zero Pressure\n(F = leave as is)"=TRUE) -> ("Array out"=w908:refnum<k24>[], "Uphole Pressure"=w907:dbl, "Sensor Cluster 2"=w914:T10)  [unwired: 6 in, 1 out]
                n347 = Bundle By Name(cluster=w911, "Up hole Corrected Pressure"=w907) -> (w910:T21)
                n348 = local write "Sensor Voltage Cluster"(w914) -> ()
                n349 = local write "Corrected\n Pressure \nCluster"(w910) -> ()
                n350 = local write "Uphole Pressure"(w907) -> ()
              }
            }
            n351 = local read "Input Variables and Slopes"() -> (w783:T1)
            n352 = Unbundle By Name(w783) -> ("String Pot Slope"=w782:dbl)
            n353 = call "depth read from string pot 2016.vi"("Descriptions"=w788, "error in (no error)"=w785, "String Pot \nSlope"=w782, "Array in"=w787) -> ("Array out"=w786:refnum<k24>[], "Depth"=w780:dbl, "error out"=w784:errorcluster)  [unwired: 12 in, 1 out]
            n354 = flat-sequence {
              tunnel: w780 -> [w824]
              tunnel: [w823] -> w779
              frame #0 {
                w825 = 15  # Filter Size
                # "Functional Global in \nBoxcar Integrator\nInitialize filter array to \ncurrent string pot value"
                n355 = call "Boxcar filter2016.vi"("Initialize"=TRUE, "Filter Size"=w825, "Filter Input"=w824) -> ("Filter Output"=w823:dbl)
              }
            }
            n356 = flat-sequence {
              tunnel: [w827] -> w781
              frame #0 {
                n357 = Tick Count (ms)() -> (millisecond timer value=w829:u32)
                n358 = Divide(x=w829, y=u32 1000) -> (x/y=w827:dbl)
              }
            }
            n359 = flat-sequence {
              tunnel: [w834] -> w776
              tunnel: w779 -> [w831]
              tunnel: w781 -> [w833]
              tunnel: w777 -> [w832]
              frame #0 {
                n360 = local read "Current Depth"() -> (w830:sgl)
                n361 = Bundle By Name(cluster=w832, "Previous Relative Depth"=w831, "Current Relative Depth"=w831, "First Relative Depth"=w831, "Current Measurement Time"=w833, "Previous Measurement Time"=w833, "Absolute Depth In"=w830, "Current Absolute Depth"=w830, "First Absolute Depth"=w830) -> (w834:T18)
              }
            }
            n362 = flat-sequence {
              tunnel: w788 -> [w900]
              tunnel: w786 -> [w903]
              tunnel: [w898] -> w801
              tunnel: [w900] -> w803
              tunnel: [w899] -> w799
              tunnel: [w897] -> w797
              frame #0 {
                w904 = 0.0  # Offset
                n363 = local read "Input Variables and Slopes"() -> (w902:T1)
                n364 = Unbundle By Name(w902) -> ("Flow Slope"=w901:dbl)
                n365 = local read "Input Depths \nand Parameters Cluster"() -> (w906:T17)
                n366 = call "Flow 2016.vi"("Descriptions"=w900, "Array in"=w903, "Flow Slope"=w901, "Offset"=w904) -> ("Sensor Cluster"=w898:T10, "Flow (ml/min)"=w899:dbl, "Array out"=w897:refnum<k24>[])  [unwired: 4 in]
                n367 = local write "Sensor Voltage Cluster"(w898) -> ()
                n368 = Bundle By Name(cluster=w906, "Flow"=w899) -> (w905:T17)
                n369 = local write "Input Depths \nand Parameters Cluster"(w905) -> ()
              }
            }
            n370 = flat-sequence {
              tunnel: w803 -> [w885]
              tunnel: w802 -> [w865]
              tunnel: w801 -> [w884]
              tunnel: w776 -> [w883]
              tunnel: [w882] -> w800
              tunnel: w799 -> [w881]
              tunnel: w797 -> [w875]
              tunnel: [w874] -> _
              tunnel: [w856] -> w796
              tunnel: w789 -> [w869]
              tunnel: w775 -> [w860]
              tunnel: [w857] -> w774
              tunnel: w773 -> [w853]
              tunnel: [w851] -> w772
              frame #0 {
                n371 = local read "Culmulative Graph Cluster"() -> (w873:T20)
                n372 = local read "Input Depths \nand Parameters Cluster"() -> (w878:T17)
                n373 = local read "Input Variables and Slopes"() -> (w880:T1)
                n374 = local read "Uphole Pressure"() -> (w852:dbl)
                n375 = local read "KPRO Finish\nIndicator"() -> (w870:bool)
                n376 = local read "Depth mode"() -> (w866:bool)
                n377 = Unbundle By Name(w880) -> ("String Pot Slope"=w879:dbl)
                n378 = Unbundle By Name(w878) -> ()  [unwired: 1 out]
                n379 = call "Kpro Read String Pot 2016.vi"("Read String Pot"=w866, "Feet of\nStainless to be\nUsed (Count) in"=w853, "Session Array in"=dbl[][] [], "Flow"=w881, "Finished In"=w870, "Depth Cluster in"=w883, "String Pot \nSlope in"=w879, "Sensor Cluster In in"=w884, "Descriptions"=w885, "Pressure in"=w852, "Array in"=w875, "Downhole Pressure Sensor"=w869, "Initial Measurement Input"=TRUE) -> ("Sensor Cluster 2"=w876:T10, "Array out"=w874:refnum<k24>[], "Generate Array Calc IK"=w858:bool, "Feet of\nStainless to be\nUsed (Count) out"=w851:i32, "Depth Cluster out"=w882:T18, "Single String Pot Session Array out"=w857:dbl[][])  [unwired: 6 in, 3 out]
                n380 = local write "Current Session"(w857) -> ()
                n381 = Build Array (concatenate)(w865, w860) -> (w861:dbl[][])
                n382 = local write "Sensor Voltage Cluster"(w876) -> ()
                n383 = Unbundle By Name(w882) -> ("Current Absolute Depth"=w864:dbl)
                n384 = Bundle By Name(cluster=w878, "Feet of Stainless"=w851) -> (w877:T17)
                n385 = local write "Input Depths \nand Parameters Cluster"(w877) -> ()
                n386 = flat-sequence {
                  tunnel: w864 -> [w890]
                  frame #0 {
                    n387 = global write "Kpro Globals.vi" "Current Depth"(w890) -> ()
                    n388 = local write "Current Depth"(w890) -> ()
                    n389 = Divide(x=w890, y=3.281) -> (x/y=w891:dbl)
                    n390 = local read "Sample Sheet Data Row Cluster 2"() -> (w895:T2)
                    n391 = local read "Corrected\n Pressure \nCluster"() -> (w893:T21)
                    n392 = Unbundle By Name(w893) -> ("Up hole Corrected Pressure"=w892:dbl)
                    n393 = Bundle By Name(cluster=w895, "Depth"=w890, "Head\nPressure"=w892) -> (w894:T2)
                    n394 = local write "Sample Sheet Data Row Cluster 2"(w894) -> ()
                    n395 = local write "Current \nDepth (m)"(w891) -> ()
                  }
                }
                n396 = case shown="True" FALSE {
                  tunnel: w857 -> [_ w889]
                  tunnel: [w886 w888] -> w856
                  tunnel: w861 -> [w886 w887]
                  frame False {
                  }
                  frame True {
                    n397 = Build Array (concatenate)(w887, w889) -> (w888:dbl[][])
                  }
                }
                n398 = call "Array to Plot 2016.vi"("Input Cumulative Array"=w856, "Input Real Time Array"=w857) -> ("Cumulative - Depth vs.Drive Rate"=w855:cluster{dbl[], dbl[]}, "Cumulative - Depth vs. Ik"=w871:cluster{dbl[], dbl[]}, "Real Time - Depth vs. Drive Rate"=w854:cluster{dbl[], dbl[]}, "Real Time - Depth vs. Ik"=w867:cluster{dbl[], dbl[]}, "Depth Rate"=w863:dbl)  [unwired: 2 in, 1 out]
                n399 = Bundle By Name(cluster=w873, "Cumulative - Depth vs. Ik"=w871, "Real Time - Depth vs. lk"=w867, "Cumulative - Depth vs. Drive Rate"=w855, "Real Time - Depth vs. Drive Rate"=w854) -> (w872:T20)
                n400 = local write "Culmulative Graph Cluster"(w872) -> ()
                n401 = local write "Large Depth IK Graph Cluster"(w867) -> ()
                n402 = local write "Depth Rate\nft/min"(w863) -> ()
                n403 = local write "Cumulative_data_from_file"(w856) -> ()
                n404 = control-ref of="KPRO SessionOutput File Path"() -> (w868:refnum<vi>)
                n405 = call "write KPRO file.vi"("Corrected Array in"=w856, "Generate Array Calc IK"=w858, "Path in"=w868) -> ()  [unwired: 7 in, 2 out]
              }
            }
          }
          frame "Increment Depth Manually" {
            n406 = local read "Input Variables and Slopes"() -> (w928:T1)
            n407 = flat-sequence {
              tunnel: w942 -> [w1044]
              tunnel: [w1043] -> w941
              tunnel: w928 -> [w1042]
              tunnel: w927 -> [w1041]
              tunnel: [w1040] -> w926
              tunnel: [w1036] -> w924
              frame #0 {
                n408 = flat-sequence {
                  tunnel: [w1061] -> w1049
                  tunnel: [w1050] -> w1048
                  tunnel: [w1060] -> w1047
                  tunnel: [w1059] -> w1046
                  tunnel: [w1058] -> w1045
                  tunnel: w1044 -> [w1057]
                  tunnel: [w1056] -> w1043
                  tunnel: w1042 -> [w1052]
                  tunnel: [w1050] -> w1036
                  frame #0 {
                    n409 = local read "Zero In-Line Pressure\n(F = leave as is)"() -> (w1051:bool)
                    n410 = Unbundle By Name(w1052) -> ("DH Pressure Trans Slope"=w1059:dbl, "DH Pressure Offset"=w1058:dbl)
                    n411 = local read "Sensor Voltage Cluster"() -> (w1054:T10)
                    n412 = local write "Input Variables and Slopes"(w1052) -> ()
                    n413 = local read "Descriptions"() -> (w1055:string[])
                    n414 = global read "Kpro Globals.vi" "Current Depth"() -> (w1061:sgl)
                    n415 = call "DHT Pressure 2016.vi"("Sensor Cluster"=w1054, "DHT Pressure Offset"=w1058, "Array in"=w1057, "DHT Pressure \nSlope"=w1059, "Descriptions"=w1055, "Zero Pressure\n(F = leave as is)"=w1051) -> ("Array out"=w1056:refnum<k24>[], "DHT Pressure"=w1060:dbl, "Sensor Cluster 2"=w1053:T10)  [unwired: 7 in]
                    n416 = local write "Sensor Voltage Cluster"(w1053) -> ()
                    n417 = Add(x=w1060, y=w1061) -> (x+y=w1050:dbl)
                    n418 = local write "Down hole Pressure"(w1050) -> ()
                  }
                }
                n419 = local read "Record DTW File"() -> (w1039:bool)
                n420 = case shown="True" w1039 {
                  selector: w1039 -> [w1063 _]
                  tunnel: [w1063 FALSE ("Boolean")] -> _
                  tunnel: w1048 -> [_ w1071]
                  tunnel: w1049 -> [_ w1072]
                  tunnel: w1045 -> [_ w1069]
                  tunnel: w1047 -> [_ w1070]
                  tunnel: w1046 -> [_ w1068]
                  tunnel: w1041 -> [w1062 w1067]
                  tunnel: [w1062 w1066] -> w1040
                  frame False {
                  }
                  frame True {
                    n421 = Build Array(w1072, w1071, w1070, w1069, w1068) -> (w1075:dbl[])
                    n422 = local read "Down hole Pressure Transducer CSV data  path"() -> (w1064:path)
                    n423 = call-poly <vilib>:"Write Delimited Spreadsheet.vi"("file path (dialog if empty)"=w1064, "1D data"=w1075, "append to file? (new file:F)"=TRUE, "error in (no error)"=w1067, "delimiter (\\t)"="," ("delimiter (\\t)")) -> ("error out"=w1066:errorcluster)  [unwired: 9 in, 1 out]
                  }
                }
                n424 = local read "Corrected\n Pressure \nCluster"() -> (w1037:T21)
                n425 = Bundle By Name(cluster=w1037, "Down hole Corrected Pressure"=w1036) -> (w1038:T21)
                n426 = local write "Corrected\n Pressure \nCluster"(w1038) -> ()
              }
            }
            n427 = flat-sequence {
              tunnel: w941 -> [w1030]
              tunnel: [w1026] -> w940
              tunnel: [w1025] -> w939
              frame #0 {
                n428 = local read "Input Variables and Slopes"() -> (w1033:T1)
                n429 = Unbundle By Name(w1033) -> ("Up Hole Pressure Slope"=w1032:dbl, "Up Hole  Pressure Offset"=w1029:dbl)
                n430 = local write "Input Variables and Slopes"(w1033) -> ()
                n431 = local read "Sensor Voltage Cluster"() -> (w1034:T10)
                n432 = local read "Descriptions"() -> (w1026:string[])
                n433 = local read "Corrected\n Pressure \nCluster"() -> (w1028:T21)
                n434 = call "up hole Pressure 2016.vi"("Sensor Cluster"=w1034, "Pressure Offset"=w1029, "Array in"=w1030, "Pressure \nSlope"=w1032, "Descriptions"=w1026, "Zero Pressure\n(F = leave as is)"=TRUE) -> ("Array out"=w1025:refnum<k24>[], "Uphole Pressure"=w1024:dbl, "Sensor Cluster 2"=w1031:T10)  [unwired: 6 in, 1 out]
                n435 = Bundle By Name(cluster=w1028, "Up hole Corrected Pressure"=w1024) -> (w1027:T21)
                n436 = local write "Sensor Voltage Cluster"(w1031) -> ()
                n437 = local write "Corrected\n Pressure \nCluster"(w1027) -> ()
                n438 = local write "Uphole Pressure"(w1024) -> ()
              }
            }
            n439 = flat-sequence {
              tunnel: w940 -> [w1017]
              tunnel: w939 -> [w1020]
              tunnel: [w1015] -> w936
              tunnel: [w1017] -> w938
              tunnel: [w1016] -> w933
              tunnel: [w1014] -> w931
              frame #0 {
                w1021 = 0.0  # Offset
                n440 = local read "Input Variables and Slopes"() -> (w1019:T1)
                n441 = Unbundle By Name(w1019) -> ("Flow Slope"=w1018:dbl)
                n442 = local read "Input Depths \nand Parameters Cluster"() -> (w1023:T17)
                n443 = call "Flow 2016.vi"("Descriptions"=w1017, "Array in"=w1020, "Flow Slope"=w1018, "Offset"=w1021) -> ("Sensor Cluster"=w1015:T10, "Flow (ml/min)"=w1016:dbl, "Array out"=w1014:refnum<k24>[])  [unwired: 4 in]
                n444 = local write "Sensor Voltage Cluster"(w1015) -> ()
                n445 = Bundle By Name(cluster=w1023, "Flow"=w1016) -> (w1022:T17)
                n446 = local write "Input Depths \nand Parameters Cluster"(w1022) -> ()
              }
            }
            n447 = flat-sequence {
              tunnel: w938 -> [w997]
              tunnel: w937 -> [w967]
              tunnel: w936 -> [w996]
              tunnel: w935 -> [w953]
              tunnel: [w995] -> w934
              tunnel: w933 -> [w994]
              tunnel: w931 -> [w988]
              tunnel: [w987] -> _
              tunnel: [w960] -> w930
              tunnel: w925 -> [w983]
              tunnel: w924 -> [w976]
              tunnel: [w959] -> w922
              tunnel: w921 -> [w965]
              tunnel: w919 -> [w955]
              tunnel: [w954] -> w920
              frame #0 {
                n448 = Unbundle By Name(w953) -> ("Current Relative Depth"=w977:dbl)
                n449 = Unbundle By Name(w953) -> ("Current Absolute Depth"=w952:dbl)
                n450 = local read "Input Depths \nand Parameters Cluster"() -> (w979:T17)
                n451 = Unbundle By Name(w979) -> ("Start Depth"=w978:sgl)
                n452 = global read "Kpro Globals.vi" "increment_amount"() -> (w981:dbl)
                n453 = local read "Culmulative Graph Cluster"() -> (w986:T20)
                n454 = local read "Input Depths \nand Parameters Cluster"() -> (w991:T17)
                n455 = Equal?(x=w952, y=w978) -> (x = y?=w973:bool)
                n456 = And(x=w973, y=FALSE) -> (x .and. y?=w974:bool)
                n457 = First Call?() -> ()  [unwired: 1 out]
                n458 = local read "Input Variables and Slopes"() -> (w993:T1)
                n459 = local read "Uphole Pressure"() -> (w956:dbl)
                n460 = local read "KPRO Finish\nIndicator"() -> (w980:bool)
                n461 = local read "Depth mode"() -> (w964:bool)
                n462 = case shown="True" w974 {
                  tunnel: w977 -> [w1001 w1002]
                  tunnel: [w1000 w1002] -> w982
                  tunnel: w981 -> [w999 _]
                  frame False {
                    n463 = Add(x=w999, y=w1001) -> (x+y=w1000:dbl)
                  }
                  frame True {
                  }
                }
                n464 = Unbundle By Name(w991) -> ()  [unwired: 2 out]
                n465 = Unbundle By Name(w993) -> ("String Pot Slope"=w992:dbl)
                n466 = call "Kpro Read String Pot 2016.vi"("Read String Pot"=w964, "Feet of\nStainless to be\nUsed (Count) in"=w955, "Session Array in"=w965, "Flow"=w994, "Manual Depth In"=w982, "Finished In"=w980, "Depth Cluster in"=w953, "error in (no error)"=w983, "String Pot \nSlope in"=w992, "Sensor Cluster In in"=w996, "Descriptions"=w997, "Pressure in"=w956, "Array in"=w988, "Downhole Pressure Sensor"=w976, "Initial Measurement Input"=FALSE) -> ("Sensor Cluster 2"=w989:T10, "IK"=w966:dbl, "Array out"=w987:refnum<k24>[], "Generate Array Calc IK"=w949:bool, "Depth Rate"=→"Depth Rate\nft/min":dbl, "Feet of\nStainless to be\nUsed (Count) out"=w954:i32, "Depth Cluster out"=w995:T18, "Single String Pot Session Array out"=w959:dbl[][])  [unwired: 4 in, 1 out]
                "Ik" <- w966
                n467 = And(x=w964, y=w949) -> ()  [unwired: 1 out]
                n468 = local write "Sensor Voltage Cluster"(w989) -> ()
                n469 = Unbundle By Name(w995) -> ("Current Absolute Depth"=w969:dbl)
                n470 = Bundle By Name(cluster=w991, "Feet of Stainless"=w954) -> (w990:T17)
                n471 = local write "Ik"(w966) -> ()
                n472 = local write "Input Depths \nand Parameters Cluster"(w990) -> ()
                n473 = flat-sequence {
                  tunnel: w969 -> [w1007]
                  frame #0 {
                    n474 = local read "Corrected\n Pressure \nCluster"() -> (w1010:T21)
                    n475 = global write "Kpro Globals.vi" "Current Depth"(w1007) -> ()
                    n476 = local write "Current Depth"(w1007) -> ()
                    n477 = Divide(x=w1007, y=3.281) -> (x/y=w1008:dbl)
                    n478 = local read "Sample Sheet Data Row Cluster 2"() -> (w1012:T2)
                    n479 = local write "Current \nDepth (m)"(w1008) -> ()
                    n480 = Unbundle By Name(w1010) -> ("Up hole Corrected Pressure"=w1009:dbl)
                    n481 = Bundle By Name(cluster=w1012, "Depth"=w1007, "Head\nPressure"=w1009) -> (w1011:T2)
                    n482 = local write "Sample Sheet Data Row Cluster 2"(w1011) -> ()
                  }
                }
                n483 = case shown="True" FALSE {
                  tunnel: w959 -> [_ w1004]
                  tunnel: [w1003 w1005] -> w960
                  tunnel: w967 -> [w1003 w1006]
                  frame False {
                  }
                  frame True {
                    n484 = Build Array (concatenate)(w1006, w1004) -> (w1005:dbl[][])
                  }
                }
                n485 = call "Array to Plot 2016.vi"("Input Cumulative Array"=w960, "Input Real Time Array"=w959) -> ("Cumulative - Depth vs.Drive Rate"=w957:cluster{dbl[], dbl[]}, "Cumulative - Depth vs. Ik"=w984:cluster{dbl[], dbl[]}, "Real Time - Depth vs. Drive Rate"=w958:cluster{dbl[], dbl[]}, "Real Time - Depth vs. Ik"=w971:cluster{dbl[], dbl[]}, "Depth Rate"=w968:dbl)  [unwired: 2 in, 1 out]
                n486 = Bundle By Name(cluster=w986, "Cumulative - Depth vs. Ik"=w984, "Real Time - Depth vs. lk"=w971, "Cumulative - Depth vs. Drive Rate"=w957, "Real Time - Depth vs. Drive Rate"=w958) -> (w985:T20)
                n487 = local write "Culmulative Graph Cluster"(w985) -> ()
                n488 = local write "Large Depth IK Graph Cluster"(w971) -> ()
                n489 = local write "Depth Rate\nft/min"(w968) -> ()
                n490 = control-ref of="KPRO Cumulative Output File Path"() -> (w950:refnum<vi>)
                n491 = control-ref of="KPRO SessionOutput File Path"() -> (w961:refnum<vi>)
                n492 = call "write KPRO file.vi"("Corrected Array in"=w959, "Generate Array Calc IK"=w949, "Path in"=w961) -> ("paths ok"=w972:bool, "appended path"=w975:path)  [unwired: 7 in]
                n493 = case shown="True" w972 {
                  tunnel: w975 -> [_ w998]
                  frame False {
                  }
                  frame True {
                    n494 = local write "KPRO SessionOutput File Path"(w998) -> ()
                  }
                }
                n495 = call "write KPRO file.vi"("Corrected Array in"=w960, "Generate Array Calc IK"=w949, "Path in"=w950) -> ()  [unwired: 7 in, 2 out]
                n496 = local write "Current Session"(w959) -> ()
                n497 = local write "Cumulative_data_from_file"(w960) -> ()
              }
            }
          }
          frame "Sample Not Collected" {
            n498 = local write "Tab Control"(T4."Sonde Data Graphs" ("Tab Control")) -> ()
          }
          frame "Record Sonde Reason" {
            n499 = flat-sequence {
              tunnel: w1094 -> [w1112]
              tunnel: [w1111] -> w1093
              frame #0 {
                n500 = local read "Sample Sheet Data Row Cluster 2"() -> (w1129:T2)
                n501 = local write "Tab Control"(T4."Recording Reason Sonde" ("Tab Control")) -> ()
                n502 = property on="Select Reasons to Record Data" class="Ring (strict)"() -> ("Strings []"=w1121:string[])  [unwired: 2 in, 2 out]
                n503 = Get Date/Time In Seconds() -> (seconds since 1Jan1904=w1128:timestamp)
                n504 = Unbundle By Name(w1129) -> ("Head\nPressure"=w1127:dbl, "Depth"=w1126:dbl)
                n505 = local read "Recording Reason Sonde array"() -> (w1116:string[][])
                n506 = local read "Sonde Recording Error file"() -> (w1113:path)
                n507 = Index Array(array=w1121, index="Select Reasons to Record Data") -> (element=w1119:string)
                n508 = Format Date/Time String(seconds (now)=w1128) -> (date/time string=w1125:string)  [unwired: 2 in]
                n509 = Format Into String(w1127) -> (resulting string=w1124:string)  [unwired: 3 in, 1 out]
                n510 = Format Into String(w1126) -> (resulting string=w1123:string)  [unwired: 3 in, 1 out]
                n511 = Format Into String("Select Reasons to Record Data") -> (resulting string=w1122:string)  [unwired: 3 in, 1 out]
                n512 = Build Array(w1125, w1124, w1123, w1122, w1119) -> (w1114:string[])
                n513 = Build Array (concatenate)(w1116, w1114) -> (→"Recording Reason Sonde array":string[][])
                n514 = call-poly <vilib>:"Write Delimited Spreadsheet.vi"("file path (dialog if empty)"=w1113, "1D data"=w1114, "append to file? (new file:F)"=TRUE, "error in (no error)"=w1112, "delimiter (\\t)"="," ("delimiter (\\t)")) -> ("error out"=w1111:errorcluster)  [unwired: 9 in, 1 out]
              }
            }
          }
          frame "Record IK Reason" {
            n515 = flat-sequence {
              frame #0 {
                n516 = local read "Select Entry for IK Log"() -> (w1151:u16)
                n517 = property on="Select Entry for IK Log" class="Ring (strict)"() -> ("Strings []"=w1150:string[])  [unwired: 2 in, 2 out]
                n518 = local read "Sample Sheet Data Row Cluster 2"() -> (w1163:T2)
                n519 = local write "Tab Control"(T4."Pressure/Flow/IK Graphs" ("Tab Control")) -> ()
                n520 = Get Date/Time In Seconds() -> (seconds since 1Jan1904=w1162:timestamp)
                n521 = Unbundle By Name(w1163) -> ("Head\nPressure"=w1161:dbl, "Depth"=w1160:dbl)
                n522 = Index Array(array=w1150, index=w1151) -> (element=w1154:string)
                n523 = Format Date/Time String(seconds (now)=w1162) -> (date/time string=w1158:string)  [unwired: 2 in]
                n524 = local read "IK Reason array"() -> (w1147:string[][])
                n525 = Format Into String(w1161) -> (resulting string=w1157:string)  [unwired: 3 in, 1 out]
                n526 = Format Into String(w1160) -> (resulting string=w1156:string)  [unwired: 3 in, 1 out]
                n527 = Format Into String(w1151) -> (resulting string=w1155:string)  [unwired: 3 in, 1 out]
                n528 = Build Array(w1158, w1157, w1156, w1155, w1154) -> (w1153:string[])
                n529 = Build Array (concatenate)(w1147, w1153) -> (→"IK Reason array":string[][])
                n530 = call-poly <vilib>:"Write Delimited Spreadsheet.vi"("file path (dialog if empty)"="Sonde IK Recording Failure Path", "1D data"=w1153, "append to file? (new file:F)"=TRUE, "delimiter (\\t)"="," ("delimiter (\\t)")) -> ()  [unwired: 10 in, 2 out]
              }
            }
          }
          frame "Continuous  Sonde Data" {
            n531 = local read "Found Quanta Sonde Com Port"() -> (w1186:refnum<visa-resource-name>)
            n532 = control-ref of="Sonde Data Display"() -> (w1189:refnum<vi>)
            n533 = local read "Sample Sheet Data Row Cluster 2"() -> (w1167:T2)
            n534 = Unbundle By Name(w1167) -> ("Sonde Data Cluster.Cumulative\nVolume (ml)"=w1166:dbl)
            n535 = call "SDI-12 Continuous Operations.vi"("RS232 Port In"=w1186, "Sensor Address In"="0", "Sonde Data Ctl Refnum"=w1189, "Error In (No Error)"=w1188) -> ("output cluster"=w1165:T3, "Temperature"=w1184:cluster{"Y":dbl[], "Y":dbl[]}[], "Sonde Data Display"=w1183:T14, "Error Out"=w1187:errorcluster)  [unwired: 8 in, 4 out]
            n536 = Bundle By Name(cluster=w1165, "Cumulative\nVolume (ml)"=w1166) -> (w1164:T3)
            n537 = Bundle By Name(cluster=w1167, "Sonde Data Cluster"=w1164) -> (w1185:T2)
            n538 = local write "Temperature"(w1184) -> ()
            n539 = local write "Sonde Data Display"(w1183) -> ()
            n540 = local write "Sample Sheet Data Row Cluster 2"(w1185) -> ()
          }
          frame "Acq. Single Sonde Point" {
            n541 = invoke on="Record Single Sample" class="Bool" method="Reinit To Default"(error in=w1220) -> (error out=w1219:errorcluster)  [unwired: 2 in, 2 out]
            n542 = call <vilib>:"Clear Errors.vi"("error in (no error)"=w1219) -> ("error out"=w1209:errorcluster)  [unwired: 5 in, 1 out]
            n543 = case shown="False" FALSE {
              tunnel: w1227 -> [w1230 w1238]
              tunnel: [w1229 w1234] -> w1226
              tunnel: [w1230 w1233] -> w1223
              tunnel: [w1228 w1232] -> w1222
              tunnel: w1209 -> [w1229 w1231]
              tunnel: w1194 -> [w1228 _]
              frame False {
              }
              frame True {
                n544 = call "get sample sheet data cells.vi"("error in (no error)"=w1231, "NI_report in"=w1238) -> ("error out"=w1235:errorcluster, "data"=w1237:string[][], "NI_report out"=w1233:refnum<class "NI_report.lvclass">, "left edge output cluster"=w1236:cluster{"row":i32, "column":i32})  [unwired: 5 in, 1 out]
                n545 = flat-sequence {
                  tunnel: w1235 -> [w1250]
                  tunnel: [w1243] -> _
                  tunnel: w1236 -> [w1248]
                  tunnel: [w1247] -> w1234
                  tunnel: [w1246] -> _
                  tunnel: [w1245] -> w1232
                  tunnel: w1237 -> [w1243]
                  frame #0 {
                    n546 = Array Subset(array=w1243, index (col)=2 ("index")) -> (w1239:string[][])  [unwired: 3 in]
                    n547 = local write "subarray"(w1239) -> ()
                    n548 = local read "Current Sample Sheet"() -> (w1242:string)
                    n549 = call "find last occupied cell.vi"("data"=w1243, "Active Sheet"=w1242, "Header Rows to remove"=3, "sub array start"=w1248, "error in (no error)"=w1250) -> ("row max value"=w1246:i32, "column max value"=w1241:i32, 13:"start of last occupied row"=w1245:cluster{"row":i32, "column":i32}, 14:"start of last occupied row"=w1240:string, "error out"=w1247:errorcluster)  [unwired: 4 in, 2 out]
                    n550 = local write "last occupied cell's name"(w1240) -> ()
                    n551 = local write "row max value"(w1241) -> ()
                  }
                }
              }
            }
            n552 = flat-sequence {
              tunnel: w1226 -> [w1313]
              tunnel: [w1312] -> w1197
              tunnel: w1215 -> [w1311]
              tunnel: [w1310] -> w1214
              tunnel: [w1309] -> w1213
              tunnel: w1212 -> [w1308]
              tunnel: [w1300] -> w1205
              tunnel: [w1297] -> _
              tunnel: w1201 -> [w1307]
              tunnel: [w1296] -> _
              frame #0 {
                n553 = local read "Sample Sheet Data Row Cluster 2"() -> (w1299:T2)
                n554 = control-ref of="Found Quanta Sonde Com Port"() -> (w1306:refnum<vi>)
                n555 = control-ref of="Current Time (s)"() -> (w1302:refnum<vi>)
                n556 = control-ref of="Sonde Data Display"() -> (w1305:refnum<vi>)
                n557 = control-ref of="Sonde Data Display"() -> (w1304:refnum<vi>)
                n558 = local write "Tab Control"(T4."Sonde Data" ("Tab Control")) -> ()
                n559 = control-ref of="Temperature"() -> (w1303:refnum<vi>)
                n560 = call "Sonde Single Measurement Subvi.vi"("VISAResourceName in"=w1306, "Time Array"=w1311, "Cumulative Sonde Data"=w1308, "Previous time"=w1307, "Sonde Data Display"=w1305, "Sonde Graph in"=w1304, "Temp Graph 3"=w1303, "error in (no error)"=w1313, "Row Cluster Input"=w1299, "reference 5"=w1302) -> ("seconds since 1Jan1904"=w1297:timestamp, "Cumulative Sonde \nData Out"=w1309:dbl[][], "Sample Sheet Data Row Cluster 2"=w1300:T2, "output cluster"=→"output cluster":T3, "time array out"=w1310:dbl[], "error out"=w1312:errorcluster)
                n561 = local write "Sample Sheet Data Row Cluster 2"(w1300) -> ()
                n562 = To Double Precision Float(number=w1297) -> (double precision float=w1296:dbl)
              }
            }
            n563 = flat-sequence {
              tunnel: w1205 -> [w1295]
              tunnel: w1204 -> [w1292]
              tunnel: w1192 -> [w1283]
              tunnel: [w1289] -> w1199
              tunnel: w1197 -> [w1288]
              tunnel: [w1287] -> w1196
              tunnel: [w1286] -> w1191
              frame #0 {
                n564 = Increment(x=w1283) -> (x+1=w1286:i32)
                n565 = local read "Sonde Data Array"() -> (w1291:T13)
                n566 = call "populate sonde row cluster from sonde data cluster.vi"("Initialize \nInitial Value \nCluster"=TRUE ("Initialize \nInitial Value \nCluster"), "error in (no error)"=w1288, "Sonde Parameters \nInitial Values"=w1292, "Sample Sheet Data Row Cluster"=w1295, "Sonde Parameters \nTolerance Limits"="Sonde Parameters \nTolerance Limits") -> ("error out"=w1287:errorcluster, "Cluster"=w1284:T26, "Sonde Parameters \nInitial Values Out"=w1289:T6)  [unwired: 4 in]
                n567 = local write "Sonde Parameters \nInitial Values"(w1289) -> ()
                n568 = Array Subset(array=w1291, length=w1283) -> (w1285:T13)  [unwired: 1 in]
                n569 = local write "Sonde Array Size"(w1283) -> ()
                n570 = Build Array (concatenate)(w1285, w1284) -> (w1290:T26[])
                n571 = local write "Sonde Data Array"(w1290) -> ()
              }
            }
            n572 = case shown="False" FALSE {
              tunnel: w1225 -> [_ w1267]
              tunnel: w1224 -> [_ w1266]
              tunnel: w1223 -> [w1253 w1265]
              tunnel: w1222 -> [w1254 w1264]
              tunnel: [w1253 w1262] -> w1221
              tunnel: [w1252 w1261] -> w1218
              tunnel: [w1254 w1260] -> w1217
              tunnel: [w1251 w1259] -> w1216
              tunnel: w1205 -> [_ w1258]
              tunnel: w1191 -> [w1251 w1257]
              tunnel: w1196 -> [w1252 w1256]
              frame False {
              }
              frame True {
                n573 = call "write out sonde row.vi"("NI_report in"=w1265, "Columns"=w1267, "Column of Volume"=w1266, "Sample Sheet Data Row Cluster"=w1258, "row index"=w1257, "error in (no error)"=w1256, "start of last occupied row"=w1264) -> ("NI_report out"=w1263:refnum<class "NI_report.lvclass">, "row index out"=w1259:i32, "error out"=w1255:errorcluster)  [unwired: 6 in]
                n574 = flat-sequence {
                  tunnel: w1255 -> [w1282]
                  tunnel: w1263 -> [w1281]
                  tunnel: [w1280] -> w1262
                  tunnel: [w1275] -> w1261
                  tunnel: [w1273] -> w1260
                  frame #0 {
                    n575 = local read "Current Sample Sheet"() -> (w1271:string)
                    n576 = call <vilib>:"Clear Errors.vi"("error in (no error)"=w1282) -> ("error out"=w1269:errorcluster)  [unwired: 5 in, 1 out]
                    n577 = call "get sample sheet data cells.vi"("error in (no error)"=w1269, "NI_report in"=w1281) -> ("error out"=w1276:errorcluster, "data"=w1277:string[][], "NI_report out"=w1280:refnum<class "NI_report.lvclass">, "left edge output cluster"=w1274:cluster{"row":i32, "column":i32})  [unwired: 5 in, 1 out]
                    n578 = call "find last occupied cell.vi"("data"=w1277, "Active Sheet"=w1271, "Header Rows to remove"=3, "sub array start"=w1274, "error in (no error)"=w1276) -> ("row max value"=w1272:i32, 13:"start of last occupied row"=w1273:cluster{"row":i32, "column":i32}, 14:"start of last occupied row"=w1270:string, "error out"=w1275:errorcluster)  [unwired: 4 in, 3 out]
                    n579 = Array Subset(array=w1277, index (col)=2 ("index")) -> (w1268:string[][])  [unwired: 3 in]
                    n580 = local write "row max value"(w1272) -> ()
                    n581 = local write "last occupied cell's name"(w1270) -> ()
                    n582 = local write "subarray"(w1268) -> ()
                  }
                }
              }
            }
          }
          frame "pH Calibration Zero" {
            n583 = invoke on="Record Single Sample" class="Bool" method="Reinit To Default"(error in=w1337) -> (error out=w1336:errorcluster)  [unwired: 2 in, 2 out]
            n584 = call <vilib>:"Clear Errors.vi"("error in (no error)"=w1336) -> ("error out"=w1324:errorcluster)  [unwired: 5 in, 1 out]
            n585 = case shown="True" FALSE {
              tunnel: w1352 -> [w1355 w1363]
              tunnel: [w1354 w1359] -> w1351
              tunnel: [w1355 w1358] -> w1347
              tunnel: [w1353 w1357] -> w1345
              tunnel: w1324 -> [w1354 w1356]
              tunnel: w1314 -> [w1353 _]
              frame False {
              }
              frame True {
                n586 = call "get sample sheet data cells.vi"("error in (no error)"=w1356, "NI_report in"=w1363) -> ("error out"=w1360:errorcluster, "data"=w1362:string[][], "NI_report out"=w1358:refnum<class "NI_report.lvclass">, "left edge output cluster"=w1361:cluster{"row":i32, "column":i32})  [unwired: 5 in, 1 out]
                n587 = flat-sequence {
                  tunnel: w1360 -> [w1373]
                  tunnel: [w1367] -> _
                  tunnel: w1361 -> [w1371]
                  tunnel: [w1370] -> w1359
                  tunnel: [w1369] -> _
                  tunnel: [w1368] -> w1357
                  tunnel: w1362 -> [w1367]
                  frame #0 {
                    n588 = local read "Current Sample Sheet"() -> (w1366:string)
                    n589 = call "find last occupied cell.vi"("data"=w1367, "Active Sheet"=w1366, "Header Rows to remove"=3, "sub array start"=w1371, "error in (no error)"=w1373) -> ("row max value"=w1369:i32, "column max value"=w1365:i32, 13:"start of last occupied row"=w1368:cluster{"row":i32, "column":i32}, 14:"start of last occupied row"=w1364:string, "error out"=w1370:errorcluster)  [unwired: 4 in, 2 out]
                    n590 = local write "row max value"(w1365) -> ()
                    n591 = local write "last occupied cell's name"(w1364) -> ()
                  }
                }
              }
            }
            n592 = local read "Found Quanta Sonde Com Port"() -> (w1341:refnum<visa-resource-name>)
            n593 = Equal?(x=w1341, y=refnum<visa-resource-name> refnum ("RS232 Port Out")) -> (x = y?=w1343:bool)
            n594 = case shown="False" w1343 {
              tunnel: w1341 -> [w1399 _]
              tunnel: [w1407 w1430] -> w1344
              tunnel: w1351 -> [w1401 w1433]
              tunnel: [w1410 w1433] -> w1348
              tunnel: w1331 -> [w1406 w1432]
              tunnel: [w1405 w1420] -> w1330
              tunnel: [w1404 w1419] -> w1329
              tunnel: w1328 -> [w1403 w1431]
              tunnel: w1327 -> [_ w1416]
              frame False {
                w1402 = "0" ("Sensor Address In")
                n595 = control-ref of="Sonde Data Display"() -> (w1411:refnum<vi>)
                n596 = local read "Sample Sheet Data Row Cluster 2"() -> (w1408:T2)
                n597 = call "Calibrate pH Sensor.vi"("Calibration Standard"="pH Zero", "Error In (No Error)"=w1401, "Sensor Address In"=w1402, "RS232 Port In"=w1399) -> ("Error Out"=w1400:errorcluster, "RS232 Port Out"=w1398:refnum<visa-resource-name>, "Calibration Response"=→"pH Zero Calibration Response":T16)  [unwired: 2 in, 3 out]
                n598 = call "SDI-12 Single Operation with output cluster.vi"("RS232 Port In"=w1398, "Sensor Address In"=w1402, "Sonde Data Ctl Refnum"=w1411, "Error In (No Error)"=w1400, "Time Array In"=w1406, "Measurement Array In"=w1403) -> ("time array out"=w1405:dbl[], "Measurement  array Out"=w1404:dbl[][], "output cluster"=w1409:T3, "Temperature"=w1413:cluster{"Y":dbl[], "Y":dbl[]}[], "Sonde Data Display"=w1412:T14, "Error Out"=w1410:errorcluster)  [unwired: 12 in, 4 out]
                n599 = local write "Temperature"(w1413) -> ()
                n600 = local write "Sonde Data Display"(w1412) -> ()
                n601 = Bundle By Name(cluster=w1408, "Sonde Data Cluster"=w1409) -> (w1407:T2)
              }
              frame True {
                n602 = Get Date/Time In Seconds() -> (seconds since 1Jan1904=w1422:timestamp)
                n603 = To Double Precision Float(number=w1422) -> (double precision float=w1421:dbl)
                n604 = local read "Sample Sheet Data Row Cluster 2"() -> (w1430:T2)
                n605 = Subtract(x=w1421, y=w1416) -> (x-y=w1414:dbl)
                n606 = local write "Current Time (s)"(w1414) -> ()
                n607 = Unbundle By Name(w1430) -> ("Sonde Data Cluster.Temp deg C"=w1415:dbl, "Sonde Data Cluster.pH"=w1429:dbl, "Sonde Data Cluster.Specific\nCond (mS)"=w1428:dbl, "Sonde Data Cluster.Salinity"=w1427:dbl, "Sonde Data Cluster.Dissolved\nOxygen mg/L"=w1426:dbl, "Sonde Data Cluster.ORP"=w1425:dbl)  [unwired: 1 out]
                n608 = Build Array(w1415, w1429, w1428, w1427, w1426, 0.0 ("element"), w1425) -> (w1423:dbl[])
                n609 = Build Array (concatenate)(w1431, w1423) -> (w1419:dbl[][])
                n610 = Build Array (concatenate)(w1432, w1414) -> (w1420:dbl[])
                n611 = call "format into Sonde Vertical Graph Data Input.vi"("Sonde Measurement Array"=w1419, "Time Array"=w1420) -> ("Sonde Data Display"=w1418:T14, "Temperature"=w1417:cluster{"X":dbl[], "Y":dbl[]}[])  [unwired: 8 in]
                n612 = local write "Temperature"(w1417) -> ()
                n613 = local write "Sonde Data Display"(w1418) -> ()
              }
            }
            n614 = local write "Sample Sheet Data Row Cluster 2"(w1344) -> ()
            n615 = call "write out sonde row.vi"("NI_report in"=w1347, "Columns"=w1350, "Column of Volume"=w1349, "Sample Sheet Data Row Cluster"=w1344, "row index"=w1333, "error in (no error)"=w1348, "start of last occupied row"=w1345) -> ("NI_report out"=w1339:refnum<class "NI_report.lvclass">, "row index out"=w1332:i32, "error out"=w1340:errorcluster)  [unwired: 6 in]
            n616 = case shown="False" FALSE {
              tunnel: w1340 -> [w1375 w1381]
              tunnel: w1339 -> [w1376 w1380]
              tunnel: [w1376 w1379] -> w1338
              tunnel: [w1375 w1378] -> w1335
              tunnel: [w1374 w1377] -> w1334
              tunnel: w1314 -> [w1374 _]
              frame False {
              }
              frame True {
                n617 = flat-sequence {
                  tunnel: w1381 -> [w1395]
                  tunnel: w1380 -> [w1394]
                  tunnel: [w1393] -> w1379
                  tunnel: [w1388] -> w1378
                  tunnel: [w1386] -> w1377
                  frame #0 {
                    n618 = call <vilib>:"Clear Errors.vi"("error in (no error)"=w1395) -> ("error out"=w1382:errorcluster)  [unwired: 5 in, 1 out]
                    n619 = local read "Current Sample Sheet"() -> (w1384:string)
                    n620 = call "get sample sheet data cells.vi"("error in (no error)"=w1382, "NI_report in"=w1394) -> ("error out"=w1389:errorcluster, "data"=w1390:string[][], "NI_report out"=w1393:refnum<class "NI_report.lvclass">, "left edge output cluster"=w1387:cluster{"row":i32, "column":i32})  [unwired: 5 in, 1 out]
                    n621 = call "find last occupied cell.vi"("data"=w1390, "Active Sheet"=w1384, "Header Rows to remove"=3, "sub array start"=w1387, "error in (no error)"=w1389) -> ("row max value"=w1385:i32, 13:"start of last occupied row"=w1386:cluster{"row":i32, "column":i32}, 14:"start of last occupied row"=w1383:string, "error out"=w1388:errorcluster)  [unwired: 4 in, 3 out]
                    n622 = Array Subset(array=w1390, index (col)=2 ("index")) -> ()  [unwired: 3 in, 1 out]
                    n623 = local write "row max value"(w1385) -> ()
                    n624 = local write "last occupied cell's name"(w1383) -> ()
                  }
                }
              }
            }
          }
          frame "pH Calibration Standard" {
            n625 = invoke on="Record Single Sample" class="Bool" method="Reinit To Default"(error in=w1459) -> (error out=w1458:errorcluster)  [unwired: 2 in, 2 out]
            n626 = call <vilib>:"Clear Errors.vi"("error in (no error)"=w1458) -> ("error out"=w1446:errorcluster)  [unwired: 5 in, 1 out]
            n627 = case shown="True" FALSE {
              tunnel: w1473 -> [w1489 w1497]
              tunnel: [w1488 w1493] -> w1472
              tunnel: [w1489 w1492] -> w1468
              tunnel: [w1487 w1491] -> w1435
              tunnel: w1446 -> [w1488 w1490]
              tunnel: w1436 -> [w1487 _]
              frame False {
              }
              frame True {
                n628 = call "get sample sheet data cells.vi"("error in (no error)"=w1490, "NI_report in"=w1497) -> ("error out"=w1494:errorcluster, "data"=w1496:string[][], "NI_report out"=w1492:refnum<class "NI_report.lvclass">, "left edge output cluster"=w1495:cluster{"row":i32, "column":i32})  [unwired: 5 in, 1 out]
                n629 = flat-sequence {
                  tunnel: w1494 -> [w1508]
                  tunnel: [w1501] -> _
                  tunnel: w1495 -> [w1506]
                  tunnel: [w1505] -> w1493
                  tunnel: [w1504] -> _
                  tunnel: [w1503] -> w1491
                  tunnel: w1496 -> [w1501]
                  frame #0 {
                    n630 = local read "Current Sample Sheet"() -> (w1500:string)
                    n631 = Array Subset(array=w1501, index (col)=2 ("index")) -> ()  [unwired: 3 in, 1 out]
                    n632 = call "find last occupied cell.vi"("data"=w1501, "Active Sheet"=w1500, "Header Rows to remove"=3, "sub array start"=w1506, "error in (no error)"=w1508) -> ("row max value"=w1504:i32, "column max value"=w1499:i32, 13:"start of last occupied row"=w1503:cluster{"row":i32, "column":i32}, 14:"start of last occupied row"=w1498:string, "error out"=w1505:errorcluster)  [unwired: 4 in, 2 out]
                    n633 = local write "last occupied cell's name"(w1498) -> ()
                    n634 = local write "row max value"(w1499) -> ()
                  }
                }
              }
            }
            n635 = local read "Found Quanta Sonde Com Port"() -> (w1463:refnum<visa-resource-name>)
            n636 = Equal?(x=w1463, y=refnum<visa-resource-name> refnum ("RS232 Port Out")) -> (x = y?=w1465:bool)
            n637 = case shown="False" w1465 {
              tunnel: w1463 -> [w1533 _]
              tunnel: [w1542 w1566] -> w1466
              tunnel: w1472 -> [w1536 w1569]
              tunnel: [w1545 w1569] -> w1469
              tunnel: w1453 -> [w1541 w1568]
              tunnel: [w1540 w1556] -> w1452
              tunnel: [w1539 w1555] -> w1451
              tunnel: w1450 -> [w1538 w1567]
              tunnel: w1449 -> [_ w1552]
              frame False {
                n638 = control-ref of="Sonde Data Display"() -> (w1546:refnum<vi>)
                n639 = call "Calibrate pH Sensor.vi"("Calibration Standard"="pH Reference", "Error In (No Error)"=w1536, "Sensor Address In"="0", "RS232 Port In"=w1533) -> ("Error Out"=w1535:errorcluster, "RS232 Port Out"=w1532:refnum<visa-resource-name>, "Calibration Response"=→"pH Reference Calibration Response":T16)  [unwired: 2 in, 3 out]
                n640 = local read "Sample Sheet Data Row Cluster 2"() -> (w1543:T2)
                n641 = call "SDI-12 Single Operation with output cluster.vi"("RS232 Port In"=w1532, "Sensor Address In"="0", "Sonde Data Ctl Refnum"=w1546, "Error In (No Error)"=w1535, "Time Array In"=w1541, "Measurement Array In"=w1538) -> ("time array out"=w1540:dbl[], "Measurement  array Out"=w1539:dbl[][], "output cluster"=w1544:T3, "Temperature"=w1548:cluster{"Y":dbl[], "Y":dbl[]}[], "Sonde Data Display"=w1547:T14, "Error Out"=w1545:errorcluster)  [unwired: 12 in, 4 out]
                n642 = Bundle By Name(cluster=w1543, "Sonde Data Cluster"=w1544) -> (w1542:T2)
                n643 = local write "Temperature"(w1548) -> ()
                n644 = local write "Sonde Data Display"(w1547) -> ()
              }
              frame True {
                n645 = Get Date/Time In Seconds() -> (seconds since 1Jan1904=w1558:timestamp)
                n646 = To Double Precision Float(number=w1558) -> (double precision float=w1557:dbl)
                n647 = local read "Sample Sheet Data Row Cluster 2"() -> (w1566:T2)
                n648 = Subtract(x=w1557, y=w1552) -> (x-y=w1550:dbl)
                n649 = local write "Current Time (s)"(w1550) -> ()
                n650 = Unbundle By Name(w1566) -> ("Sonde Data Cluster.Temp deg C"=w1551:dbl, "Sonde Data Cluster.pH"=w1565:dbl, "Sonde Data Cluster.Specific\nCond (mS)"=w1564:dbl, "Sonde Data Cluster.Salinity"=w1563:dbl, "Sonde Data Cluster.Dissolved\nOxygen mg/L"=w1562:dbl, "Sonde Data Cluster.ORP"=w1561:dbl)  [unwired: 1 out]
                n651 = Build Array(w1551, w1565, w1564, w1563, w1562, 0.0 ("element"), w1561) -> (w1559:dbl[])
                n652 = Build Array (concatenate)(w1567, w1559) -> (w1555:dbl[][])
                n653 = Build Array (concatenate)(w1568, w1550) -> (w1556:dbl[])
                n654 = call "format into Sonde Vertical Graph Data Input.vi"("Sonde Measurement Array"=w1555, "Time Array"=w1556) -> ("Sonde Data Display"=w1554:T14, "Temperature"=w1553:cluster{"X":dbl[], "Y":dbl[]}[])  [unwired: 8 in]
                n655 = local write "Temperature"(w1553) -> ()
                n656 = local write "Sonde Data Display"(w1554) -> ()
              }
            }
            n657 = case shown="False" FALSE {
              tunnel: w1471 -> [_ w1486]
              tunnel: w1470 -> [_ w1485]
              tunnel: w1469 -> [w1476 w1484]
              tunnel: w1468 -> [w1475 w1483]
              tunnel: w1466 -> [_ w1482]
              tunnel: [w1476 w1481] -> w1462
              tunnel: [w1475 w1480] -> w1461
              tunnel: w1455 -> [w1474 w1479]
              tunnel: [w1474 w1478] -> w1454
              tunnel: w1435 -> [_ w1477]
              frame False {
              }
              frame True {
                n658 = call "write out sonde row.vi"("NI_report in"=w1483, "Columns"=w1486, "Column of Volume"=w1485, "Sample Sheet Data Row Cluster"=w1482, "row index"=w1479, "error in (no error)"=w1484, "start of last occupied row"=w1477) -> ("NI_report out"=w1480:refnum<class "NI_report.lvclass">, "row index out"=w1478:i32, "error out"=w1481:errorcluster)  [unwired: 6 in]
              }
            }
            n659 = local write "Sample Sheet Data Row Cluster 2"(w1466) -> ()
            n660 = case shown="False" FALSE {
              tunnel: w1462 -> [w1510 w1516]
              tunnel: w1461 -> [w1511 w1515]
              tunnel: [w1511 w1514] -> w1460
              tunnel: [w1510 w1513] -> w1457
              tunnel: [w1509 w1512] -> w1456
              tunnel: w1435 -> [w1509 _]
              frame False {
              }
              frame True {
                n661 = flat-sequence {
                  tunnel: w1516 -> [w1530]
                  tunnel: w1515 -> [w1529]
                  tunnel: [w1528] -> w1514
                  tunnel: [w1523] -> w1513
                  tunnel: [w1521] -> w1512
                  frame #0 {
                    n662 = call <vilib>:"Clear Errors.vi"("error in (no error)"=w1530) -> ("error out"=w1517:errorcluster)  [unwired: 5 in, 1 out]
                    n663 = local read "Current Sample Sheet"() -> (w1519:string)
                    n664 = call "get sample sheet data cells.vi"("error in (no error)"=w1517, "NI_report in"=w1529) -> ("error out"=w1524:errorcluster, "data"=w1525:string[][], "NI_report out"=w1528:refnum<class "NI_report.lvclass">, "left edge output cluster"=w1522:cluster{"row":i32, "column":i32})  [unwired: 5 in, 1 out]
                    n665 = call "find last occupied cell.vi"("data"=w1525, "Active Sheet"=w1519, "Header Rows to remove"=3, "sub array start"=w1522, "error in (no error)"=w1524) -> ("row max value"=w1520:i32, 13:"start of last occupied row"=w1521:cluster{"row":i32, "column":i32}, 14:"start of last occupied row"=w1518:string, "error out"=w1523:errorcluster)  [unwired: 4 in, 3 out]
                    n666 = Array Subset(array=w1525, index (col)=2 ("index")) -> ()  [unwired: 3 in, 1 out]
                    n667 = local write "row max value"(w1520) -> ()
                    n668 = local write "last occupied cell's name"(w1518) -> ()
                  }
                }
              }
            }
          }
          frame "ORP Calibration Standard" {
            n669 = invoke on="Record Single Sample" class="Bool" method="Reinit To Default"(error in=w1595) -> (error out=w1594:errorcluster)  [unwired: 2 in, 2 out]
            n670 = call <vilib>:"Clear Errors.vi"("error in (no error)"=w1594) -> ("error out"=w1584:errorcluster)  [unwired: 5 in, 1 out]
            n671 = case shown="True" FALSE {
              tunnel: w1609 -> [w1611 w1620]
              tunnel: [w1612 w1616] -> w1608
              tunnel: [w1611 w1615] -> w1604
              tunnel: w1584 -> [w1612 w1614]
              tunnel: [w1610 w1613] -> w1573
              tunnel: w1570 -> [w1610 _]
              frame False {
              }
              frame True {
                n672 = call "get sample sheet data cells.vi"("error in (no error)"=w1614, "NI_report in"=w1620) -> ("error out"=w1617:errorcluster, "data"=w1619:string[][], "NI_report out"=w1615:refnum<class "NI_report.lvclass">, "left edge output cluster"=w1618:cluster{"row":i32, "column":i32})  [unwired: 5 in, 1 out]
                n673 = flat-sequence {
                  tunnel: w1617 -> [w1631]
                  tunnel: [w1624] -> _
                  tunnel: w1618 -> [w1629]
                  tunnel: [w1628] -> w1616
                  tunnel: [w1627] -> _
                  tunnel: [w1626] -> w1613
                  tunnel: w1619 -> [w1624]
                  frame #0 {
                    n674 = local read "Current Sample Sheet"() -> (w1623:string)
                    n675 = Array Subset(array=w1624, index (col)=2 ("index")) -> ()  [unwired: 3 in, 1 out]
                    n676 = call "find last occupied cell.vi"("data"=w1624, "Active Sheet"=w1623, "Header Rows to remove"=3, "sub array start"=w1629, "error in (no error)"=w1631) -> ("row max value"=w1627:i32, "column max value"=w1622:i32, 13:"start of last occupied row"=w1626:cluster{"row":i32, "column":i32}, 14:"start of last occupied row"=w1621:string, "error out"=w1628:errorcluster)  [unwired: 4 in, 2 out]
                    n677 = local write "last occupied cell's name"(w1621) -> ()
                    n678 = local write "row max value"(w1622) -> ()
                  }
                }
              }
            }
            n679 = local read "Found Quanta Sonde Com Port"() -> (w1599:refnum<visa-resource-name>)
            n680 = Equal?(x=w1599, y=refnum<visa-resource-name> refnum ("RS232 Port Out")) -> (x = y?=w1601:bool)
            n681 = case shown="False" w1601 {
              tunnel: w1599 -> [w1669 _]
              tunnel: [w1678 w1702] -> w1602
              tunnel: w1608 -> [w1671 w1705]
              tunnel: [w1681 w1705] -> w1605
              tunnel: w1589 -> [w1677 w1704]
              tunnel: [w1676 w1692] -> w1588
              tunnel: [w1675 w1691] -> w1577
              tunnel: w1576 -> [w1674 w1703]
              tunnel: w1587 -> [_ w1688]
              frame False {
                n682 = control-ref of="Sonde Data Display"() -> (w1682:refnum<vi>)
                n683 = call "Calibrate ORP Sensor2.vi"("Calibration Standard"="ORP Reference", "Error In (No Error)"=w1671, "Sensor Address In"="0", "RS232 Port In"=w1669) -> ("Error Out"=w1670:errorcluster, "RS232 Port Out"=w1668:refnum<visa-resource-name>, "Calibration Response"=→"ORP Reference Calibration Response":T16)  [unwired: 2 in, 3 out]
                n684 = local read "Sample Sheet Data Row Cluster 2"() -> (w1679:T2)
                n685 = call "SDI-12 Single Operation with output cluster.vi"("RS232 Port In"=w1668, "Sensor Address In"="0", "Sonde Data Ctl Refnum"=w1682, "Error In (No Error)"=w1670, "Time Array In"=w1677, "Measurement Array In"=w1674) -> ("time array out"=w1676:dbl[], "Measurement  array Out"=w1675:dbl[][], "output cluster"=w1680:T3, "Temperature"=w1684:cluster{"Y":dbl[], "Y":dbl[]}[], "Sonde Data Display"=w1683:T14, "Error Out"=w1681:errorcluster)  [unwired: 12 in, 4 out]
                n686 = Bundle By Name(cluster=w1679, "Sonde Data Cluster"=w1680) -> (w1678:T2)
                n687 = local write "Temperature"(w1684) -> ()
                n688 = local write "Sonde Data Display"(w1683) -> ()
              }
              frame True {
                n689 = Get Date/Time In Seconds() -> (seconds since 1Jan1904=w1694:timestamp)
                n690 = To Double Precision Float(number=w1694) -> (double precision float=w1693:dbl)
                n691 = local read "Sample Sheet Data Row Cluster 2"() -> (w1702:T2)
                n692 = Subtract(x=w1693, y=w1688) -> (x-y=w1686:dbl)
                n693 = local write "Current Time (s)"(w1686) -> ()
                n694 = Unbundle By Name(w1702) -> ("Sonde Data Cluster.Temp deg C"=w1687:dbl, "Sonde Data Cluster.pH"=w1701:dbl, "Sonde Data Cluster.Specific\nCond (mS)"=w1700:dbl, "Sonde Data Cluster.Salinity"=w1699:dbl, "Sonde Data Cluster.Dissolved\nOxygen mg/L"=w1698:dbl, "Sonde Data Cluster.ORP"=w1697:dbl)  [unwired: 1 out]
                n695 = Build Array(w1687, w1701, w1700, w1699, w1698, 0.0 ("element"), w1697) -> (w1695:dbl[])
                n696 = Build Array (concatenate)(w1703, w1695) -> (w1691:dbl[][])
                n697 = Build Array (concatenate)(w1704, w1686) -> (w1692:dbl[])
                n698 = call "format into Sonde Vertical Graph Data Input.vi"("Sonde Measurement Array"=w1691, "Time Array"=w1692) -> ("Sonde Data Display"=w1690:T14, "Temperature"=w1689:cluster{"X":dbl[], "Y":dbl[]}[])  [unwired: 8 in]
                n699 = local write "Temperature"(w1689) -> ()
                n700 = local write "Sonde Data Display"(w1690) -> ()
              }
            }
            n701 = case shown="False" FALSE {
              tunnel: w1607 -> [_ w1644]
              tunnel: w1606 -> [_ w1643]
              tunnel: w1605 -> [w1634 w1642]
              tunnel: w1604 -> [w1633 w1641]
              tunnel: w1602 -> [_ w1640]
              tunnel: [w1634 w1639] -> w1598
              tunnel: [w1633 w1638] -> w1597
              tunnel: w1591 -> [w1632 w1637]
              tunnel: [w1632 w1636] -> w1590
              tunnel: w1573 -> [_ w1635]
              frame False {
              }
              frame True {
                n702 = call "write out sonde row.vi"("NI_report in"=w1641, "Columns"=w1644, "Column of Volume"=w1643, "Sample Sheet Data Row Cluster"=w1640, "row index"=w1637, "error in (no error)"=w1642, "start of last occupied row"=w1635) -> ("NI_report out"=w1638:refnum<class "NI_report.lvclass">, "row index out"=w1636:i32, "error out"=w1639:errorcluster)  [unwired: 6 in]
              }
            }
            n703 = local write "Sample Sheet Data Row Cluster 2"(w1602) -> ()
            n704 = case shown="False" FALSE {
              tunnel: w1598 -> [w1646 w1652]
              tunnel: w1597 -> [w1647 w1651]
              tunnel: [w1647 w1650] -> w1596
              tunnel: [w1646 w1649] -> w1593
              tunnel: [w1645 w1648] -> w1592
              tunnel: w1573 -> [w1645 _]
              frame False {
              }
              frame True {
                n705 = flat-sequence {
                  tunnel: w1652 -> [w1666]
                  tunnel: w1651 -> [w1665]
                  tunnel: [w1664] -> w1650
                  tunnel: [w1659] -> w1649
                  tunnel: [w1657] -> w1648
                  frame #0 {
                    n706 = call <vilib>:"Clear Errors.vi"("error in (no error)"=w1666) -> ("error out"=w1653:errorcluster)  [unwired: 5 in, 1 out]
                    n707 = local read "Current Sample Sheet"() -> (w1655:string)
                    n708 = call "get sample sheet data cells.vi"("error in (no error)"=w1653, "NI_report in"=w1665) -> ("error out"=w1660:errorcluster, "data"=w1661:string[][], "NI_report out"=w1664:refnum<class "NI_report.lvclass">, "left edge output cluster"=w1658:cluster{"row":i32, "column":i32})  [unwired: 5 in, 1 out]
                    n709 = call "find last occupied cell.vi"("data"=w1661, "Active Sheet"=w1655, "Header Rows to remove"=3, "sub array start"=w1658, "error in (no error)"=w1660) -> ("row max value"=w1656:i32, 13:"start of last occupied row"=w1657:cluster{"row":i32, "column":i32}, 14:"start of last occupied row"=w1654:string, "error out"=w1659:errorcluster)  [unwired: 4 in, 3 out]
                    n710 = Array Subset(array=w1661, index (col)=2 ("index")) -> ()  [unwired: 3 in, 1 out]
                    n711 = local write "row max value"(w1656) -> ()
                    n712 = local write "last occupied cell's name"(w1654) -> ()
                  }
                }
              }
            }
          }
          frame "Salinity Calibration Standard" {
            n713 = invoke on="Record Single Sample" class="Bool" method="Reinit To Default"(error in=w1731) -> (error out=w1730:errorcluster)  [unwired: 2 in, 2 out]
            n714 = call <vilib>:"Clear Errors.vi"("error in (no error)"=w1730) -> ("error out"=w1718:errorcluster)  [unwired: 5 in, 1 out]
            n715 = case shown="False" FALSE {
              tunnel: w1745 -> [w1748 w1756]
              tunnel: [w1747 w1752] -> w1744
              tunnel: [w1748 w1751] -> w1740
              tunnel: w1718 -> [w1747 w1750]
              tunnel: [w1746 w1749] -> w1708
              tunnel: w1706 -> [w1746 _]
              frame False {
              }
              frame True {
                n716 = call "get sample sheet data cells.vi"("error in (no error)"=w1750, "NI_report in"=w1756) -> ("error out"=w1753:errorcluster, "data"=w1755:string[][], "NI_report out"=w1751:refnum<class "NI_report.lvclass">, "left edge output cluster"=w1754:cluster{"row":i32, "column":i32})  [unwired: 5 in, 1 out]
                n717 = flat-sequence {
                  tunnel: w1753 -> [w1767]
                  tunnel: [w1760] -> _
                  tunnel: w1754 -> [w1765]
                  tunnel: [w1764] -> w1752
                  tunnel: [w1763] -> _
                  tunnel: [w1762] -> w1749
                  tunnel: w1755 -> [w1760]
                  frame #0 {
                    n718 = Array Subset(array=w1760, index (col)=2 ("index")) -> ()  [unwired: 3 in, 1 out]
                    n719 = local read "Current Sample Sheet"() -> (w1759:string)
                    n720 = call "find last occupied cell.vi"("data"=w1760, "Active Sheet"=w1759, "Header Rows to remove"=3, "sub array start"=w1765, "error in (no error)"=w1767) -> ("row max value"=w1763:i32, "column max value"=w1758:i32, 13:"start of last occupied row"=w1762:cluster{"row":i32, "column":i32}, 14:"start of last occupied row"=w1757:string, "error out"=w1764:errorcluster)  [unwired: 4 in, 2 out]
                    n721 = local write "last occupied cell's name"(w1757) -> ()
                    n722 = local write "row max value"(w1758) -> ()
                  }
                }
              }
            }
            n723 = local read "Found Quanta Sonde Com Port"() -> (w1735:refnum<visa-resource-name>)
            n724 = Equal?(x=w1735, y=refnum<visa-resource-name> refnum ("RS232 Port Out")) -> (x = y?=w1737:bool)
            n725 = case shown="False" w1737 {
              tunnel: w1735 -> [w1808 _]
              tunnel: [w1814 w1838] -> w1738
              tunnel: w1744 -> [w1806 w1841]
              tunnel: [w1817 w1841] -> w1741
              tunnel: w1725 -> [w1813 w1840]
              tunnel: [w1812 w1828] -> w1724
              tunnel: [w1811 w1827] -> w1723
              tunnel: w1722 -> [w1810 w1839]
              tunnel: w1721 -> [_ w1824]
              frame False {
                n726 = call "Calibrate Salinity Sensor2.vi"("Calibration Standard"="Salinity \nReference", "Error In (No Error)"=w1806, "Sensor Address In"="0", "RS232 Port In"=w1808) -> ("Error Out"=w1805:errorcluster, "RS232 Port Out"=w1807:refnum<visa-resource-name>, "Calibration Response"=→"Salinity Reference Calibration Response":T16)  [unwired: 2 in, 3 out]
                n727 = control-ref of="Sonde Data Display"() -> (w1818:refnum<vi>)
                n728 = local read "Sample Sheet Data Row Cluster 2"() -> (w1815:T2)
                n729 = call "SDI-12 Single Operation with output cluster.vi"("RS232 Port In"=w1807, "Sensor Address In"="0", "Sonde Data Ctl Refnum"=w1818, "Error In (No Error)"=w1805, "Time Array In"=w1813, "Measurement Array In"=w1810) -> ("time array out"=w1812:dbl[], "Measurement  array Out"=w1811:dbl[][], "output cluster"=w1816:T3, "Temperature"=w1820:cluster{"Y":dbl[], "Y":dbl[]}[], "Sonde Data Display"=w1819:T14, "Error Out"=w1817:errorcluster)  [unwired: 12 in, 4 out]
                n730 = local write "Temperature"(w1820) -> ()
                n731 = local write "Sonde Data Display"(w1819) -> ()
                n732 = Bundle By Name(cluster=w1815, "Sonde Data Cluster"=w1816) -> (w1814:T2)
              }
              frame True {
                n733 = Get Date/Time In Seconds() -> (seconds since 1Jan1904=w1830:timestamp)
                n734 = To Double Precision Float(number=w1830) -> (double precision float=w1829:dbl)
                n735 = local read "Sample Sheet Data Row Cluster 2"() -> (w1838:T2)
                n736 = Subtract(x=w1829, y=w1824) -> (x-y=w1822:dbl)
                n737 = local write "Current Time (s)"(w1822) -> ()
                n738 = Unbundle By Name(w1838) -> ("Sonde Data Cluster.Temp deg C"=w1823:dbl, "Sonde Data Cluster.pH"=w1837:dbl, "Sonde Data Cluster.Specific\nCond (mS)"=w1836:dbl, "Sonde Data Cluster.Salinity"=w1835:dbl, "Sonde Data Cluster.Dissolved\nOxygen mg/L"=w1834:dbl, "Sonde Data Cluster.ORP"=w1833:dbl)  [unwired: 1 out]
                n739 = Build Array(w1823, w1837, w1836, w1835, w1834, 0.0 ("element"), w1833) -> (w1831:dbl[])
                n740 = Build Array (concatenate)(w1839, w1831) -> (w1827:dbl[][])
                n741 = Build Array (concatenate)(w1840, w1822) -> (w1828:dbl[])
                n742 = call "format into Sonde Vertical Graph Data Input.vi"("Sonde Measurement Array"=w1827, "Time Array"=w1828) -> ("Sonde Data Display"=w1826:T14, "Temperature"=w1825:cluster{"X":dbl[], "Y":dbl[]}[])  [unwired: 8 in]
                n743 = local write "Temperature"(w1825) -> ()
                n744 = local write "Sonde Data Display"(w1826) -> ()
              }
            }
            n745 = local write "Sample Sheet Data Row Cluster 2"(w1738) -> ()
            n746 = case shown="False" FALSE {
              tunnel: w1743 -> [_ w1780]
              tunnel: w1742 -> [_ w1779]
              tunnel: w1741 -> [w1770 w1778]
              tunnel: w1740 -> [w1768 w1777]
              tunnel: w1708 -> [_ w1776]
              tunnel: w1738 -> [_ w1775]
              tunnel: [w1770 w1774] -> w1734
              tunnel: [w1768 w1773] -> w1733
              tunnel: w1727 -> [w1769 w1772]
              tunnel: [w1769 w1771] -> w1726
              frame False {
              }
              frame True {
                n747 = call "write out sonde row.vi"("NI_report in"=w1777, "Columns"=w1780, "Column of Volume"=w1779, "Sample Sheet Data Row Cluster"=w1775, "row index"=w1772, "error in (no error)"=w1778, "start of last occupied row"=w1776) -> ("NI_report out"=w1773:refnum<class "NI_report.lvclass">, "row index out"=w1771:i32, "error out"=w1774:errorcluster)  [unwired: 6 in]
              }
            }
            n748 = case shown="False" FALSE {
              tunnel: w1734 -> [w1783 w1788]
              tunnel: w1733 -> [w1782 w1787]
              tunnel: [w1782 w1786] -> w1732
              tunnel: [w1783 w1785] -> w1729
              tunnel: [w1781 w1784] -> w1728
              tunnel: w1708 -> [w1781 _]
              frame False {
              }
              frame True {
                n749 = flat-sequence {
                  tunnel: w1788 -> [w1802]
                  tunnel: w1787 -> [w1801]
                  tunnel: [w1800] -> w1786
                  tunnel: [w1795] -> w1785
                  tunnel: [w1793] -> w1784
                  frame #0 {
                    n750 = call <vilib>:"Clear Errors.vi"("error in (no error)"=w1802) -> ("error out"=w1789:errorcluster)  [unwired: 5 in, 1 out]
                    n751 = local read "Current Sample Sheet"() -> (w1791:string)
                    n752 = call "get sample sheet data cells.vi"("error in (no error)"=w1789, "NI_report in"=w1801) -> ("error out"=w1796:errorcluster, "data"=w1797:string[][], "NI_report out"=w1800:refnum<class "NI_report.lvclass">, "left edge output cluster"=w1794:cluster{"row":i32, "column":i32})  [unwired: 5 in, 1 out]
                    n753 = call "find last occupied cell.vi"("data"=w1797, "Active Sheet"=w1791, "Header Rows to remove"=3, "sub array start"=w1794, "error in (no error)"=w1796) -> ("row max value"=w1792:i32, 13:"start of last occupied row"=w1793:cluster{"row":i32, "column":i32}, 14:"start of last occupied row"=w1790:string, "error out"=w1795:errorcluster)  [unwired: 4 in, 3 out]
                    n754 = Array Subset(array=w1797, index (col)=2 ("index")) -> ()  [unwired: 3 in, 1 out]
                    n755 = local write "row max value"(w1792) -> ()
                    n756 = local write "last occupied cell's name"(w1790) -> ()
                  }
                }
              }
            }
          }
          frame "DO Calibration Standard" {
            n757 = invoke on="Record Single Sample" class="Bool" method="Reinit To Default"(error in=w1865) -> (error out=w1864:errorcluster)  [unwired: 2 in, 2 out]
            n758 = call <vilib>:"Clear Errors.vi"("error in (no error)"=w1864) -> ("error out"=w1852:errorcluster)  [unwired: 5 in, 1 out]
            n759 = case shown="True" FALSE {
              tunnel: w1878 -> [w1880 w1889]
              tunnel: [w1881 w1885] -> w1877
              tunnel: [w1880 w1884] -> w1873
              tunnel: [w1879 w1883] -> w1871
              tunnel: w1852 -> [w1881 w1882]
              tunnel: w1842 -> [w1879 _]
              frame False {
              }
              frame True {
                n760 = call "get sample sheet data cells.vi"("error in (no error)"=w1882, "NI_report in"=w1889) -> ("error out"=w1886:errorcluster, "data"=w1888:string[][], "NI_report out"=w1884:refnum<class "NI_report.lvclass">, "left edge output cluster"=w1887:cluster{"row":i32, "column":i32})  [unwired: 5 in, 1 out]
                n761 = flat-sequence {
                  tunnel: w1886 -> [w1900]
                  tunnel: [w1893] -> _
                  tunnel: w1887 -> [w1898]
                  tunnel: [w1897] -> w1885
                  tunnel: [w1896] -> _
                  tunnel: [w1895] -> w1883
                  tunnel: w1888 -> [w1893]
                  frame #0 {
                    n762 = local read "Current Sample Sheet"() -> (w1892:string)
                    n763 = Array Subset(array=w1893, index (col)=2 ("index")) -> ()  [unwired: 3 in, 1 out]
                    n764 = call "find last occupied cell.vi"("data"=w1893, "Active Sheet"=w1892, "Header Rows to remove"=3, "sub array start"=w1898, "error in (no error)"=w1900) -> ("row max value"=w1896:i32, "column max value"=w1891:i32, 13:"start of last occupied row"=w1895:cluster{"row":i32, "column":i32}, 14:"start of last occupied row"=w1890:string, "error out"=w1897:errorcluster)  [unwired: 4 in, 2 out]
                    n765 = local write "last occupied cell's name"(w1890) -> ()
                    n766 = local write "row max value"(w1891) -> ()
                  }
                }
              }
            }
            n767 = local read "Found Quanta Sonde Com Port"() -> (w1867:refnum<visa-resource-name>)
            n768 = Equal?(x=w1867, y=refnum<visa-resource-name> refnum ("RS232 Port Out")) -> (x = y?=w1869:bool)
            n769 = case shown="False" w1869 {
              tunnel: w1867 -> [w1935 _]
              tunnel: [w1942 w1966] -> w1870
              tunnel: w1877 -> [w1937 w1969]
              tunnel: [w1945 w1969] -> w1874
              tunnel: w1859 -> [w1941 w1968]
              tunnel: [w1940 w1956] -> w1858
              tunnel: [w1939 w1955] -> w1857
              tunnel: w1856 -> [w1938 w1967]
              tunnel: w1855 -> [_ w1952]
              frame False {
                n770 = call "Calibrate DO Sensor2.vi"("Calibration Standard"="DO \nReference", "Error In (No Error)"=w1937, "Sensor Address In"="0", "RS232 Port In"=w1935) -> ("Error Out"=w1936:errorcluster, "RS232 Port Out"=w1934:refnum<visa-resource-name>, "Calibration Response"=→"DO Reference Calibration Response":T16)  [unwired: 2 in, 3 out]
                n771 = control-ref of="Sonde Data Display"() -> (w1946:refnum<vi>)
                n772 = call "SDI-12 Single Operation with output cluster.vi"("RS232 Port In"=w1934, "Sensor Address In"="0", "Sonde Data Ctl Refnum"=w1946, "Error In (No Error)"=w1936, "Time Array In"=w1941, "Measurement Array In"=w1938) -> ("time array out"=w1940:dbl[], "Measurement  array Out"=w1939:dbl[][], "output cluster"=w1944:T3, "Temperature"=w1948:cluster{"Y":dbl[], "Y":dbl[]}[], "Sonde Data Display"=w1947:T14, "Error Out"=w1945:errorcluster)  [unwired: 12 in, 4 out]
                n773 = local read "Sample Sheet Data Row Cluster 2"() -> (w1943:T2)
                n774 = local write "Temperature"(w1948) -> ()
                n775 = local write "Sonde Data Display"(w1947) -> ()
                n776 = Bundle By Name(cluster=w1943, "Sonde Data Cluster"=w1944) -> (w1942:T2)
              }
              frame True {
                n777 = Get Date/Time In Seconds() -> (seconds since 1Jan1904=w1958:timestamp)
                n778 = To Double Precision Float(number=w1958) -> (double precision float=w1957:dbl)
                n779 = local read "Sample Sheet Data Row Cluster 2"() -> (w1966:T2)
                n780 = Subtract(x=w1957, y=w1952) -> (x-y=w1950:dbl)
                n781 = local write "Current Time (s)"(w1950) -> ()
                n782 = Unbundle By Name(w1966) -> ("Sonde Data Cluster.Temp deg C"=w1951:dbl, "Sonde Data Cluster.pH"=w1965:dbl, "Sonde Data Cluster.Specific\nCond (mS)"=w1964:dbl, "Sonde Data Cluster.Salinity"=w1963:dbl, "Sonde Data Cluster.Dissolved\nOxygen mg/L"=w1962:dbl, "Sonde Data Cluster.ORP"=w1961:dbl)  [unwired: 1 out]
                n783 = Build Array(w1951, w1965, w1964, w1963, w1962, 0.0 ("element"), w1961) -> (w1959:dbl[])
                n784 = Build Array (concatenate)(w1967, w1959) -> (w1955:dbl[][])
                n785 = Build Array (concatenate)(w1968, w1950) -> (w1956:dbl[])
                n786 = call "format into Sonde Vertical Graph Data Input.vi"("Sonde Measurement Array"=w1955, "Time Array"=w1956) -> ("Sonde Data Display"=w1954:T14, "Temperature"=w1953:cluster{"X":dbl[], "Y":dbl[]}[])  [unwired: 8 in]
                n787 = local write "Temperature"(w1953) -> ()
                n788 = local write "Sonde Data Display"(w1954) -> ()
              }
            }
            n789 = local write "Sample Sheet Data Row Cluster 2"(w1870) -> ()
            n790 = case shown="False" FALSE {
              tunnel: w1876 -> [_ w1917]
              tunnel: w1875 -> [_ w1916]
              tunnel: w1874 -> [w1903 w1915]
              tunnel: w1873 -> [w1904 w1914]
              tunnel: w1871 -> [w1902 w1913]
              tunnel: w1870 -> [_ w1912]
              tunnel: [w1904 w1909] -> w1866
              tunnel: [w1903 w1908] -> w1863
              tunnel: [w1902 w1907] -> w1862
              tunnel: w1861 -> [w1901 w1906]
              tunnel: [w1901 w1905] -> w1860
              frame False {
              }
              frame True {
                n791 = call "write out sonde row.vi"("NI_report in"=w1914, "Columns"=w1917, "Column of Volume"=w1916, "Sample Sheet Data Row Cluster"=w1912, "row index"=w1906, "error in (no error)"=w1915, "start of last occupied row"=w1913) -> ("NI_report out"=w1910:refnum<class "NI_report.lvclass">, "row index out"=w1905:i32, "error out"=w1911:errorcluster)  [unwired: 6 in]
                n792 = flat-sequence {
                  tunnel: w1911 -> [w1930]
                  tunnel: w1910 -> [w1929]
                  tunnel: [w1928] -> w1909
                  tunnel: [w1924] -> w1908
                  tunnel: [w1922] -> w1907
                  frame #0 {
                    n793 = call <vilib>:"Clear Errors.vi"("error in (no error)"=w1930) -> ("error out"=w1918:errorcluster)  [unwired: 5 in, 1 out]
                    n794 = local read "Current Sample Sheet"() -> (w1920:string)
                    n795 = call "get sample sheet data cells.vi"("error in (no error)"=w1918, "NI_report in"=w1929) -> ("error out"=w1925:errorcluster, "data"=w1926:string[][], "NI_report out"=w1928:refnum<class "NI_report.lvclass">, "left edge output cluster"=w1923:cluster{"row":i32, "column":i32})  [unwired: 5 in, 1 out]
                    n796 = call "find last occupied cell.vi"("data"=w1926, "Active Sheet"=w1920, "Header Rows to remove"=3, "sub array start"=w1923, "error in (no error)"=w1925) -> ("row max value"=w1921:i32, 13:"start of last occupied row"=w1922:cluster{"row":i32, "column":i32}, 14:"start of last occupied row"=w1919:string, "error out"=w1924:errorcluster)  [unwired: 4 in, 3 out]
                    n797 = local write "row max value"(w1921) -> ()
                    n798 = local write "last occupied cell's name"(w1919) -> ()
                  }
                }
              }
            }
          }
          frame "SC Calibration Standard" {
            n799 = invoke on="Record Single Sample" class="Bool" method="Reinit To Default"(error in=w1993) -> (error out=w1992:errorcluster)  [unwired: 2 in, 2 out]
            n800 = call <vilib>:"Clear Errors.vi"("error in (no error)"=w1992) -> ("error out"=w1980:errorcluster)  [unwired: 5 in, 1 out]
            n801 = case shown="True" FALSE {
              tunnel: w2006 -> [w2009 w2017]
              tunnel: [w2008 w2013] -> w2005
              tunnel: [w2009 w2012] -> w2001
              tunnel: [w2007 w2011] -> w1999
              tunnel: w1980 -> [w2008 w2010]
              tunnel: w1970 -> [w2007 _]
              frame False {
              }
              frame True {
                n802 = call "get sample sheet data cells.vi"("error in (no error)"=w2010, "NI_report in"=w2017) -> ("error out"=w2014:errorcluster, "data"=w2016:string[][], "NI_report out"=w2012:refnum<class "NI_report.lvclass">, "left edge output cluster"=w2015:cluster{"row":i32, "column":i32})  [unwired: 5 in, 1 out]
                n803 = flat-sequence {
                  tunnel: w2014 -> [w2027]
                  tunnel: w2015 -> [w2025]
                  tunnel: [w2024] -> w2013
                  tunnel: [w2023] -> _
                  tunnel: [w2022] -> w2011
                  tunnel: w2016 -> [w2021]
                  frame #0 {
                    n804 = local read "Current Sample Sheet"() -> (w2020:string)
                    n805 = call "find last occupied cell.vi"("data"=w2021, "Active Sheet"=w2020, "Header Rows to remove"=3, "sub array start"=w2025, "error in (no error)"=w2027) -> ("row max value"=w2023:i32, "column max value"=w2019:i32, 13:"start of last occupied row"=w2022:cluster{"row":i32, "column":i32}, 14:"start of last occupied row"=w2018:string, "error out"=w2024:errorcluster)  [unwired: 4 in, 2 out]
                    n806 = local write "last occupied cell's name"(w2018) -> ()
                    n807 = local write "row max value"(w2019) -> ()
                  }
                }
              }
            }
            n808 = local read "Found Quanta Sonde Com Port"() -> (w1995:refnum<visa-resource-name>)
            n809 = Equal?(x=w1995, y=refnum<visa-resource-name> refnum ("RS232 Port Out")) -> (x = y?=w1997:bool)
            n810 = case shown="False" w1997 {
              tunnel: w1995 -> [w2064 _]
              tunnel: [w2070 w2094] -> w1998
              tunnel: w2005 -> [w2062 w2097]
              tunnel: [w2073 w2097] -> w2002
              tunnel: w1987 -> [w2069 w2096]
              tunnel: [w2068 w2084] -> w1986
              tunnel: [w2067 w2083] -> w1985
              tunnel: w1984 -> [w2066 w2095]
              tunnel: w1983 -> [_ w2080]
              frame False {
                n811 = call "Calibrate SC Sensor2.vi"("Calibration Standard"="SC \nReference", "Error In (No Error)"=w2062, "Sensor Address In"="0", "RS232 Port In"=w2064) -> ("Error Out"=w2061:errorcluster, "RS232 Port Out"=w2063:refnum<visa-resource-name>, "Calibration Response"=→"SC Reference Calibration Response":T16)  [unwired: 2 in, 3 out]
                n812 = control-ref of="Sonde Data Display"() -> (w2074:refnum<vi>)
                n813 = local read "Sample Sheet Data Row Cluster 2"() -> (w2071:T2)
                n814 = call <vilib>:"Clear Errors.vi"("error in (no error)"=w2061) -> ("error out"=w2059:errorcluster)  [unwired: 5 in, 1 out]
                n815 = call "SDI-12 Single Operation with output cluster.vi"("RS232 Port In"=w2063, "Sensor Address In"="0", "Sonde Data Ctl Refnum"=w2074, "Error In (No Error)"=w2059, "Time Array In"=w2069, "Measurement Array In"=w2066) -> ("time array out"=w2068:dbl[], "Measurement  array Out"=w2067:dbl[][], "output cluster"=w2072:T3, "Temperature"=w2076:cluster{"Y":dbl[], "Y":dbl[]}[], "Sonde Data Display"=w2075:T14, "Error Out"=w2073:errorcluster)  [unwired: 12 in, 4 out]
                n816 = local write "Temperature"(w2076) -> ()
                n817 = local write "Sonde Data Display"(w2075) -> ()
                n818 = Bundle By Name(cluster=w2071, "Sonde Data Cluster"=w2072) -> (w2070:T2)
              }
              frame True {
                n819 = Get Date/Time In Seconds() -> (seconds since 1Jan1904=w2086:timestamp)
                n820 = To Double Precision Float(number=w2086) -> (double precision float=w2085:dbl)
                n821 = local read "Sample Sheet Data Row Cluster 2"() -> (w2094:T2)
                n822 = Subtract(x=w2085, y=w2080) -> (x-y=w2078:dbl)
                n823 = local write "Current Time (s)"(w2078) -> ()
                n824 = Unbundle By Name(w2094) -> ("Sonde Data Cluster.Temp deg C"=w2079:dbl, "Sonde Data Cluster.pH"=w2093:dbl, "Sonde Data Cluster.Specific\nCond (mS)"=w2092:dbl, "Sonde Data Cluster.Salinity"=w2091:dbl, "Sonde Data Cluster.Dissolved\nOxygen mg/L"=w2090:dbl, "Sonde Data Cluster.ORP"=w2089:dbl)  [unwired: 1 out]
                n825 = Build Array(w2079, w2093, w2092, w2091, w2090, 0.0 ("element"), w2089) -> (w2087:dbl[])
                n826 = Build Array (concatenate)(w2095, w2087) -> (w2083:dbl[][])
                n827 = Build Array (concatenate)(w2096, w2078) -> (w2084:dbl[])
                n828 = call "format into Sonde Vertical Graph Data Input.vi"("Sonde Measurement Array"=w2083, "Time Array"=w2084) -> ("Sonde Data Display"=w2082:T14, "Temperature"=w2081:cluster{"X":dbl[], "Y":dbl[]}[])  [unwired: 8 in]
                n829 = local write "Temperature"(w2081) -> ()
                n830 = local write "Sonde Data Display"(w2082) -> ()
              }
            }
            n831 = local write "Sample Sheet Data Row Cluster 2"(w1998) -> ()
            n832 = case shown="False" FALSE {
              tunnel: w2004 -> [_ w2044]
              tunnel: w2003 -> [_ w2043]
              tunnel: w2002 -> [w2030 w2042]
              tunnel: w2001 -> [w2029 w2041]
              tunnel: w1999 -> [w2028 w2040]
              tunnel: w1998 -> [_ w2039]
              tunnel: [w2029 w2036] -> w1994
              tunnel: [w2030 w2035] -> w1991
              tunnel: [w2028 w2034] -> w1990
              tunnel: w1989 -> [w2031 w2033]
              tunnel: [w2031 w2032] -> w1988
              frame False {
              }
              frame True {
                n833 = call "write out sonde row.vi"("NI_report in"=w2041, "Columns"=w2044, "Column of Volume"=w2043, "Sample Sheet Data Row Cluster"=w2039, "row index"=w2033, "error in (no error)"=w2042, "start of last occupied row"=w2040) -> ("NI_report out"=w2037:refnum<class "NI_report.lvclass">, "row index out"=w2032:i32, "error out"=w2038:errorcluster)  [unwired: 6 in]
                n834 = flat-sequence {
                  tunnel: w2038 -> [w2057]
                  tunnel: w2037 -> [w2056]
                  tunnel: [w2055] -> w2036
                  tunnel: [w2051] -> w2035
                  tunnel: [w2049] -> w2034
                  frame #0 {
                    (unwired) 2 ("index")
                    n835 = call <vilib>:"Clear Errors.vi"("error in (no error)"=w2057) -> ("error out"=w2045:errorcluster)  [unwired: 5 in, 1 out]
                    n836 = local read "Current Sample Sheet"() -> (w2047:string)
                    n837 = call "get sample sheet data cells.vi"("error in (no error)"=w2045, "NI_report in"=w2056) -> ("error out"=w2052:errorcluster, "data"=w2053:string[][], "NI_report out"=w2055:refnum<class "NI_report.lvclass">, "left edge output cluster"=w2050:cluster{"row":i32, "column":i32})  [unwired: 5 in, 1 out]
                    n838 = call "find last occupied cell.vi"("data"=w2053, "Active Sheet"=w2047, "Header Rows to remove"=3, "sub array start"=w2050, "error in (no error)"=w2052) -> ("row max value"=w2048:i32, 13:"start of last occupied row"=w2049:cluster{"row":i32, "column":i32}, 14:"start of last occupied row"=w2046:string, "error out"=w2051:errorcluster)  [unwired: 4 in, 3 out]
                    n839 = local write "row max value"(w2048) -> ()
                    n840 = local write "last occupied cell's name"(w2046) -> ()
                  }
                }
              }
            }
          }
          frame "Write Sonde Sample Sheet" {
            n841 = flat-sequence {
              tunnel: w2124 -> [w2143]
              tunnel: w2123 -> [w2130]
              tunnel: w2121 -> [w2140]
              tunnel: w2120 -> [w2139]
              tunnel: w2119 -> [w2138]
              tunnel: [w2137] -> w2118
              tunnel: w2117 -> [w2136]
              tunnel: w2116 -> [w2135]
              tunnel: w2098 -> [w2133]
              tunnel: [w2132] -> w2114
              tunnel: [w2131] -> w2113
              tunnel: [w2126] -> w2112
              tunnel: w2101 -> [w2128]
              frame #0 {
                n842 = call <vilib>:"Clear Errors.vi"("error in (no error)"=w2130) -> ("error out"=w2125:errorcluster)  [unwired: 5 in, 1 out]
                n843 = Not Equal?(x=w2136, y=w2135) -> (x != y?=w2134:bool)
                n844 = invoke on="Update Sonde" class="Bool (strict)" method="Reinit To Default"(error in=w2125) -> (error out=w2129:errorcluster)  [unwired: 2 in, 2 out]
                n845 = case shown="True" w2134 {
                  tunnel: w2143 -> [w2157 w2179]
                  tunnel: w2133 -> [_ w2178]
                  tunnel: w2129 -> [w2156 w2177]
                  tunnel: [w2156 w2165] -> w2142
                  tunnel: [w2157 w2176] -> w2141
                  tunnel: w2138 -> [w2155 w2161]
                  tunnel: [w2155 w2160] -> w2137
                  tunnel: w2128 -> [w2154 w2159]
                  tunnel: [w2154 w2164] -> w2126
                  frame False {
                  }
                  frame True {
                    n846 = local read "Sonde Data Array"() -> (w2163:T13)
                    n847 = Decrement(x=w2159) -> (x-1=w2158:i32)
                    "Sonde Array Size" <- w2158
                    n848 = flat-sequence {
                      tunnel: [w2193] -> w2176
                      tunnel: w2179 -> [w2192]
                      tunnel: w2178 -> [w2191]
                      tunnel: w2177 -> [w2190]
                      tunnel: [w2189] -> w2170
                      frame #0 {
                        n849 = case shown="False" FALSE {
                          tunnel: [w2195 w2202] -> w2193
                          tunnel: w2192 -> [w2195 w2201]
                          tunnel: w2191 -> [_ w2198]
                          tunnel: w2190 -> [w2194 w2197]
                          tunnel: [w2194 w2196] -> w2189
                          frame False {
                          }
                          frame True {
                            n850 = call "write comment cell with column offset.vi"("Column Relative?"=TRUE, "comment string"="done", "error in (no error)"=w2197, "start of last occupied row"=w2198, "NI_report in"=w2201) -> ("error out"=w2196:errorcluster, "NI_report out"=w2202:refnum<class "NI_report.lvclass">)  [unwired: 5 in]
                          }
                        }
                      }
                    }
                    n851 = Index Array(array=w2163, index=w2158) -> (element=w2175:T27)
                    n852 = Bundle By Name(cluster=w2175, "Final"=TRUE) -> (w2174:T27)
                    n853 = Replace Array Subset(array=w2163, new element=w2174, index=w2158) -> (w2172:T13)
                    n854 = local write "Sonde Data Array"(w2172) -> ()
                    n855 = for {
                      tunnel: w2172 -> [w2187] mode=indexing
                      tunnel: w2161 -> [w2186]
                      tunnel: [w2185] -> w2171 mode=indexing
                      n856 = call "convert sonde cluster to spreadsheet array.vi"("Cluster"=w2187, "Sheet"=w2186) -> ("Sonde Data Array (String)"=w2185:string[])  [unwired: 6 in, 3 out]
                    }
                    n857 = local read "Sonde Output File Path"() -> (w2167:path)
                    n858 = call <vilib>:"Clear Errors.vi"("error in (no error)"=w2170) -> ("error out"=w2162:errorcluster)  [unwired: 5 in, 1 out]
                    n859 = flat-sequence {
                      tunnel: w2166 -> [w2184]
                      tunnel: [w2183] -> w2165
                      tunnel: [0 ("row index")] -> w2164
                      tunnel: w2161 -> [w2181]
                      tunnel: [w2180] -> w2160
                      tunnel: w2158 -> [_]
                      frame #0 {
                        n860 = invoke on="Sonde Data Array" class="Arr (strict)" method="Reinit To Default"(error in=w2184) -> (error out=w2183:errorcluster)  [unwired: 2 in, 2 out]
                        n861 = Increment(x=w2181) -> (x+1=w2180:i32)
                      }
                    }
                    n862 = call-poly <vilib>:"Write Delimited Spreadsheet.vi"("file path (dialog if empty)"=w2167, "2D data"=w2171, "append to file? (new file:F)"=TRUE, "error in (no error)"=w2162, "delimiter (\\t)"="," ("delimiter (\\t)")) -> ("error out"=w2166:errorcluster)  [unwired: 9 in, 1 out]
                  }
                }
                n863 = case shown="False" FALSE {
                  tunnel: w2142 -> [w2145 w2153]
                  tunnel: w2141 -> [w2144 w2152]
                  tunnel: w2140 -> [_ w2151]
                  tunnel: w2139 -> [_ w2150]
                  tunnel: w2137 -> [_ w2149]
                  tunnel: [w2145 w2147] -> w2132
                  tunnel: [w2144 w2146] -> w2131
                  frame False {
                  }
                  frame True {
                    n864 = call "open select sample sheet.vi"("Number of Sample Sheets"=w2150, "error in (no error)"=w2153, "Worksheet Names"=w2151, "input 1"=w2149, "NI_report in"=w2152) -> ("error out"=w2147:errorcluster, "Current Sample Sheet"=w2148:string, "NI_report out"=w2146:refnum<class "NI_report.lvclass">)  [unwired: 4 in]
                    n865 = local write "Current Sample Sheet"(w2148) -> ()
                  }
                }
              }
            }
            n866 = flat-sequence {
              tunnel: w2101 -> [w2226]
              frame #0 {
                n867 = local read "Sonde Data Array"() -> (w2229:T13)
                n868 = Index Array(array=w2229, index=w2226) -> (element=w2231:T27)
                n869 = Bundle By Name(cluster=w2231, "Final"=TRUE) -> (w2227:T27)
                n870 = Replace Array Subset(array=w2229, new element=w2227, index=w2226) -> (w2228:T13)
                n871 = local write "Sonde Data Array"(w2228) -> ()
              }
            }
            n872 = flat-sequence {
              tunnel: [w2205] -> w2122
              tunnel: [w2209] -> w2115
              tunnel: w2114 -> [w2208]
              tunnel: w2113 -> [w2207]
              tunnel: [w2206] -> w2107
              tunnel: w2098 -> [w2203]
              frame #0 {
                n873 = case shown="False" FALSE {
                  tunnel: [w2212 w2224] -> w2209
                  tunnel: w2208 -> [w2210 w2223]
                  tunnel: w2207 -> [w2211 w2222]
                  tunnel: [w2210 w2214] -> w2206
                  tunnel: [w2211 w2213] -> w2205
                  tunnel: w2203 -> [w2212 _]
                  frame False {
                  }
                  frame True {
                    n874 = local read "Current Sample Sheet"() -> (w2216:string)
                    n875 = call "get sample sheet data cells.vi"("error in (no error)"=w2223, "NI_report in"=w2222) -> ("error out"=w2225:errorcluster, "data"=w2220:string[][], "NI_report out"=w2213:refnum<class "NI_report.lvclass">, "left edge output cluster"=w2218:cluster{"row":i32, "column":i32})  [unwired: 5 in, 1 out]
                    n876 = Array Subset(array=w2220, index (col)=2 ("index")) -> ()  [unwired: 3 in, 1 out]
                    n877 = call "find last occupied cell.vi"("Active Sheet"=w2216, "Header Rows to remove"=3, "sub array start"=w2218, "error in (no error)"=w2225) -> ("row max value"=w2217:i32, 13:"start of last occupied row"=w2224:cluster{"row":i32, "column":i32}, 14:"start of last occupied row"=w2215:string, "error out"=w2214:errorcluster)  [unwired: 5 in, 3 out]
                    n878 = local write "row max value"(w2217) -> ()
                    n879 = local write "last occupied cell's name"(w2215) -> ()
                  }
                }
              }
            }
          }
          frame "Init" {
            n880 = flat-sequence {
              tunnel: w2255 -> [w2619]
              tunnel: [w2606] -> w2245
              tunnel: [w2605] -> w2244
              frame #0 {
                n881 = call "create DAQ strings.vi"("error in (no error)"=w2619, "MCC USB-DAQ Setup"="MCC USB-DAQ Setup") -> ("error IO"=w2612:errorcluster, "Descriptions"=w2610:string[], "delimited string"=w2613:string, "Array"=w2611:string[], "Voltage Range"=w2618:dbl[])  [unwired: 5 in]
                "delimited string" <- w2613
                "Active Channel Array" <- w2611
                "Voltage Range" <- w2618
                "Descriptions" <- w2610
                n882 = call "Physical Channels to Number of channels.vi"("error in (no error)"=w2612, "Physical Channel in"=w2613) -> ("error out"=w2614:errorcluster, "Number of Channels"=w2616:i32)  [unwired: 7 in, 1 out]
                "Number \nof Channels" <- w2616
                n883 = call "Calculate Rate from Num Channels and Max Rate.vi"("error in (no error)"=w2614, "Channel Data Rate S/s"="DAQ \nData Rate S/s", "Number of Channels"=w2616) -> ("error out"=w2609:errorcluster, "Rate"=→"Rate":dbl)  [unwired: 7 in]
                n884 = for {
                  tunnel: w2611 -> [w2632] mode=indexing
                  tunnel: w2618 -> [w2631] mode=indexing
                  tunnel: [w2628] -> w2608 mode=indexing
                  shift-right: [w2629] -> w2607
                  shift-left: w2609 -> [w2627]
                  n885 = Negate(x=w2631) -> (-x=w2630:dbl)
                  n886 = call-poly <vilib>:"ULx Create Virtual Channel.vi"("maximum value"=w2631, "minimum value"=w2630, "physical channels"=w2632, "error in"=w2627) -> ("task out"=w2628:refnum<k24>, "error out"=w2629:errorcluster)  [unwired: 10 in]
                }
                n887 = call "get 9V monitor voltage.vi"("error in (no error)"=w2607, "Descriptions"=w2610, "Array"=w2611, "Array 2"=w2608) -> ("error out"=w2606:errorcluster, "9V Voltage Monitor"=w2604:dbl)  [unwired: 6 in]
                "DAQ Error" <- w2606
                "9V Voltage Monitor" <- w2604
                n888 = Greater Or Equal?(x=w2604, y=8.75) -> (x >= y?=→"DAQ":bool)
                n889 = flat-sequence {
                  tunnel: [w2625] -> w2605
                  tunnel: w2608 -> [w2623]
                  tunnel: w2606 -> [w2622]
                  frame #0 {
                    n890 = local read "Descriptions"() -> (w2626:string[])
                    n891 = call "Measure DAQ Voltages.vi"("error in (no error)"=w2622, "Descriptions"=w2626, "Array in"=w2623) -> ("Raw Voltages"=w2624:dbl[], "Array out"=w2625:refnum<k24>[], "Sensor Cluster"=w2621:T10)  [unwired: 6 in]
                    n892 = local write "Sensor Voltage Cluster"(w2621) -> ()
                    n893 = local write "Raw Voltages"(w2624) -> ()
                  }
                }
              }
            }
            n894 = local write "Initialization"(-1 ("Initialization")) -> ()
            n895 = invoke on="IK Reason array" class="Arr (strict)" method="Reinit To Default"() -> ()  [unwired: 3 in, 3 out]
            n896 = invoke on="Recording Reason Sonde array" class="Arr (strict)" method="Reinit To Default"() -> ()  [unwired: 3 in, 3 out]
            n897 = flat-sequence {
              tunnel: w2245 -> [w2595]
              tunnel: [w2595] -> w2253
              frame #0 {
                w2596 = T23."Enabled" ("Disabled")
                n898 = property on="Write Data to Spreadsheet" class="Bool"("DisabledEnum"=w2596) -> (error out=w2599:errorcluster)  [unwired: 2 in, 1 out]
                n899 = property on="Record Continuous Samples" class="Bool"(error in=w2599, "DisabledEnum"=T23."Disabled and Grayed Out" ("Disabled")) -> (error out=w2598:errorcluster)  [unwired: 1 in, 1 out]
                n900 = local write "Sonde Data Array"(T13 [{"Head"=1.0, "Depth"=-5.5, "Time"="17:08:31", "Cumulative\nVolume"=100.0, "Sp. Conductance"={"Value"=2.0, "%"=0.0, "Tol."=TRUE}, "Dissolved Oxygen"={"Value"=3.0, "%"=0.0, "Tol."=TRUE}, "pH"={"Value"=4.0, "%"=0.0, "Tol."=TRUE}, "ORP"={"Value"=5.0, "%"=0.0, "Tol."=TRUE}, "Temperature"={"Value"=26.0, "%"=0.0, "Tol."=TRUE}, "Salinity"={"Value"=7.0, "%"=0.0, "Tol."=TRUE}, "Final Tol."=TRUE, "Final"=FALSE, "Time 2"=timestamp(3588613711.7180486 s since 1904-01-01), "Aux 1"=0.0, "Aux 2"=0.0, "Aux 3"=0.0}, {"Head"=1.0, "Depth"=-5.5, "Time"="17:08:34", "Cumulative\nVolume"=100.0, "Sp. Conductance"={"Value"=2.0, "%"=0.0, "Tol."=TRUE}, "Dissolved Oxygen"={"Value"=3.0, "%"=0.0, "Tol."=TRUE}, "pH"={"Value"=4.0, "%"=0.0, "Tol."=TRUE}, "ORP"={"Value"=5.0, "%"=0.0, "Tol."=TRUE}, "Temperature"={"Value"=26.0, "%"=0.0, "Tol."=TRUE}, "Salinity"={"Value"=7.0, "%"=0.0, "Tol."=TRUE}, "Final Tol."=TRUE, "Final"=FALSE, "Time 2"=timestamp(3588613714.1021852 s since 1904-01-01), "Aux 1"=0.0, "Aux 2"=0.0, "Aux 3"=0.0}, {"Head"=1.0, "Depth"=-5.5, "Time"="17:08:35", "Cumulative\nVolume"=100.0, "Sp. Conductance"={"Value"=2.0, "%"=0.0, "Tol."=TRUE}, "Dissolved Oxygen"={"Value"=3.0, "%"=0.0, "Tol."=TRUE}, "pH"={"Value"=4.0, "%"=0.0, "Tol."=TRUE}, "ORP"={"Value"=5.0, "%"=0.0, "Tol."=TRUE}, "Temperature"={"Value"=26.0, "%"=0.0, "Tol."=TRUE}, "Salinity"={"Value"=7.0, "%"=0.0, "Tol."=TRUE}, "Final Tol."=TRUE, "Final"=FALSE, "Time 2"=timestamp(3588613715.709277 s since 1904-01-01), "Aux 1"=0.0, "Aux 2"=0.0, "Aux 3"=0.0}, {"Head"=1.0, "Depth"=-5.5, "Time"="17:08:37", "Cumulative\nVolume"=100.0, "Sp. Conductance"={"Value"=2.0, "%"=0.0, "Tol."=TRUE}, "Dissolved Oxygen"={"Value"=3.0, "%"=0.0, "Tol."=TRUE}, "pH"={"Value"=4.0, "%"=0.0, "Tol."=TRUE}, "ORP"={"Value"=5.0, "%"=0.0, "Tol."=TRUE}, "Temperature"={"Value"=26.0, "%"=0.0, "Tol."=TRUE}, "Salinity"={"Value"=7.0, "%"=0.0, "Tol."=TRUE}, "Final Tol."=TRUE, "Final"=FALSE, "Time 2"=timestamp(3588613717.7793956 s since 1904-01-01), "Aux 1"=0.0, "Aux 2"=0.0, "Aux 3"=0.0}, {"Head"=1.0, "Depth"=-5.5, "Time"="17:08:39", "Cumulative\nVolume"=100.0, "Sp. Conductance"={"Value"=2.0, "%"=0.0, "Tol."=TRUE}, "Dissolved Oxygen"={"Value"=3.0, "%"=0.0, "Tol."=TRUE}, "pH"={"Value"=4.0, "%"=0.0, "Tol."=TRUE}, "ORP"={"Value"=5.0, "%"=0.0, "Tol."=TRUE}, "Temperature"={"Value"=26.0, "%"=0.0, "Tol."=TRUE}, "Salinity"={"Value"=7.0, "%"=0.0, "Tol."=TRUE}, "Final Tol."=TRUE, "Final"=FALSE, "Time 2"=timestamp(3588613719.696505 s since 1904-01-01), "Aux 1"=0.0, "Aux 2"=0.0, "Aux 3"=0.0}, {"Head"=1.0, "Depth"=-5.5, "Time"="17:09:28", "Cumulative\nVolume"=100.0, "Sp. Conductance"={"Value"=2.0, "%"=0.0, "Tol."=TRUE}, "Dissolved Oxygen"={"Value"=3.0, "%"=0.0, "Tol."=TRUE}, "pH"={"Value"=4.0, "%"=0.0, "Tol."=TRUE}, "ORP"={"Value"=5.0, "%"=0.0, "Tol."=TRUE}, "Temperature"={"Value"=26.0, "%"=0.0, "Tol."=TRUE}, "Salinity"={"Value"=7.0, "%"=0.0, "Tol."=TRUE}, "Final Tol."=TRUE, "Final"=FALSE, "Time 2"=timestamp(3588613768.340287 s since 1904-01-01), "Aux 1"=0.0, "Aux 2"=0.0, "Aux 3"=0.0}] ("Sonde Data Array")) -> ()
                n901 = property on="Record Single Sample" class="Bool"(error in=w2598, "DisabledEnum"=w2596) -> (error out=w2597:errorcluster)  [unwired: 1 in, 1 out]
                n902 = property on="Sample Not Collected" class="Bool"(error in=w2597, "DisabledEnum"=w2596) -> (error out=w2594:errorcluster)  [unwired: 1 in, 1 out]
                n903 = invoke on="Sonde Data Array" class="Arr (strict)" method="Reinit To Default"(error in=w2594) -> ()  [unwired: 2 in, 3 out]
                "Initialization Finished" <- TRUE
                "Zero Pressure\nIndicator" <- FALSE ("Zero Pressure\nIndicator")
              }
            }
            n904 = call <vilib>:"Clear Errors.vi"("error in (no error)"=w2245) -> ("error out"=w2232:errorcluster)  [unwired: 5 in, 1 out]
            n905 = local read "Descriptions"() -> (w2233:string[])
            n906 = stacked-sequence {
              seq-local: [w2262 _ _ _ _ _ _ _ _ _] -> [_ w2291 _ _ _ _ _ _ _ _]
              seq-local: [_ w2292 _ _ _ _ _ _ _ _] -> [_ _ w2313 _ _ _ _ _ _ _]
              seq-local: [_ _ w2312 _ _ _ _ _ _ _] -> [_ _ _ _ _ _ _ _ _ w2541]
              tunnel: [_ _ w2317 _ _ _ _ _ _ _] -> _
              tunnel: w2247 -> [_ _ _ _ _ _ _ _ _ w2544]
              tunnel: [_ _ _ _ _ _ _ _ _ w2543] -> w2246
              tunnel: w2232 -> [w2264 _ _ _ _ _ _ _ _ _]
              tunnel: w2244 -> [_ _ w2315 w2446 w2475 _ _ _ w2512 _]
              tunnel: w2233 -> [_ _ w2314 w2447 w2474 _ _ _ w2511 _]
              tunnel: [_ _ _ w2448 _ _ _ _ _ _] -> _
              tunnel: [_ _ _ _ _ _ _ _ _ w2541] -> w2248
              tunnel: w2236 -> [_ _ w2311 _ _ _ _ _ _ _]
              tunnel: [_ _ w2310 _ _ _ _ _ _ _] -> w2235
              frame #0 {
                n907 = flat-sequence {
                  tunnel: [w2269] -> w2262
                  tunnel: w2264 -> [w2270]
                  frame #0 {
                    n908 = local read "Groundwater Header"() -> (w2276:T11)
                    n909 = Unbundle By Name(w2276) -> ("Kpro box Serial"=w2266:string)
                    n910 = Scan From String(format string="%d", input string=w2266, error in=w2270, default 1=800.0 ("default value 1")) -> (error out=w2271:errorcluster, output 1=w2275:dbl)  [unwired: 1 in, 2 out]
                    n911 = Equal?(x=w2266, y="") -> (x = y?=w2267:bool)
                    n912 = case shown="True" w2267 {
                      tunnel: "KPRO Box Number\n\nEnter the number of the KPRO box you are using." ("prompt") -> [_ w2290]
                      tunnel: w2276 -> [w2280 w2289]
                      tunnel: w2275 -> [w2278 w2288]
                      tunnel: [w2278 w2287] -> w2274
                      tunnel: [w2280 w2285] -> w2272
                      tunnel: w2271 -> [w2279 w2283]
                      tunnel: [w2279 w2282] -> w2269
                      frame False {
                      }
                      frame True {
                        n913 = call "prompt_and_enter_value2.vi"("prompt_IN"=w2290, "Enter value"=w2288) -> ("Numeric"=w2287:dbl)  [unwired: 9 in]
                        n914 = call <vilib>:"Clear Errors.vi"("error in (no error)"=w2283) -> ("error out"=w2281:errorcluster)  [unwired: 5 in, 1 out]
                        n915 = Format Into String(format string="%d", error in=w2281, w2287) -> (resulting string=w2284:string, error out=w2282:errorcluster)  [unwired: 1 in]
                        n916 = Bundle By Name(cluster=w2289, "Kpro box Serial"=w2284) -> (w2285:T11)
                      }
                    }
                    n917 = global write "Kpro Globals.vi" "KPRO Box Number"(w2274) -> ()
                    n918 = local write "Groundwater Header"(w2272) -> ()
                  }
                }
                "Initialization" <- 0
              }
              frame #1 {
                n919 = local write "Initialization"(1 ("Initialization")) -> ()
                n920 = flat-sequence {
                  tunnel: w2291 -> [w2295]
                  tunnel: [w2294] -> w2292
                  frame #0 {
                    n921 = local read "Groundwater Header"() -> (w2303:T11)
                    n922 = local read "Temporary Data Files Directory"() -> (w2299:path)
                    n923 = Unbundle By Name(w2303) -> ("Profile ID"=w2302:string)
                    n924 = Equal?(x=w2302, y="") -> ()  [unwired: 1 out]
                    n925 = case shown="True" TRUE {
                      tunnel: "Profile ID\n\nEnter the profile ID.  This will create a directoryto store csv files and the excel file" ("prompt") -> [_ w2309]
                      tunnel: [w2306 w2308] -> w2298
                      tunnel: w2302 -> [w2306 w2307]
                      frame False {
                      }
                      frame True {
                        n926 = call "prompt_string.vi"("prompt_IN"=w2309, "Enter value"=w2307) -> ("String"=w2308:string)  [unwired: 9 in]
                        n927 = global write "Kpro Globals.vi" "Profile ID"(w2308) -> ()
                      }
                    }
                    n928 = Bundle By Name(cluster=w2303, "Profile ID"=w2298) -> (w2304:T11)
                    n929 = call-poly <userlib>:"Build Path__ogtk.vi"("name or relative path"=w2298, "base path"=w2299) -> ("appended path"=w2297:path)
                    n930 = local write "Groundwater Header"(w2304) -> ()
                    n931 = call <userlib>:"Create Dir if Non-Existant__ogtk.vi"("error in (no error)"=w2295, "Directory Path"=w2297) -> ("error out"=w2294:errorcluster, "dup Directory Path"=w2296:path)  [unwired: 7 in, 1 out]
                    n932 = local write "Output File Path"(w2296) -> ()
                  }
                }
              }
              frame #2 {
                n933 = flat-sequence {
                  tunnel: [w2340] -> w2317
                  tunnel: w2313 -> [w2347]
                  tunnel: w2315 -> [w2345]
                  tunnel: w2314 -> [w2344]
                  tunnel: [w2332] -> w2312
                  tunnel: w2311 -> [w2331]
                  tunnel: [w2330] -> w2310
                  frame #0 {
                    n934 = local read "Input Variables and Slopes"() -> (w2351:T1)
                    n935 = call <vilib>:"Clear Errors.vi"("error in (no error)"=w2347) -> ("error out"=w2333:errorcluster)  [unwired: 5 in, 1 out]
                    n936 = local read "Temporary Data Files Directory"() -> (w2346:path)
                    n937 = Unbundle By Name(w2351) -> ("Up Hole Pressure Slope"=w2354:dbl, "String Pot Slope"=w2353:dbl, "Flow Slope"=w2352:dbl)
                    n938 = call "FILE_DIALOG 2016.vi"("flow_slope_IN"=w2352, "pressure_slope_IN"=w2354, "string_pot_slope_IN"=w2353, "Descriptions"=w2344, "error in (no error)"=w2333, "start path"=w2346, "Array in"=w2345) -> ("Output path"=w2327:path, "exists"=w2343:bool, "flow_slope_OUT"=w2349:dbl, "pressure_slope_OUT"=w2348:dbl, "Record Output Slopes to  Record File"=w2328:path, "string_pot_slope_OUT"=w2350:dbl, "Record Output Slopes for slopes.csv File"=w2329:path, "error out"=w2339:errorcluster)  [unwired: 11 in, 2 out]
                    n939 = Path To String(path=w2327) -> (string=w2321:string)
                    n940 = Concatenate Strings(w2321, "\\" ("string")) -> (w2319:string)
                    n941 = String To Path(string=w2319) -> (path=w2320:path)
                    "Output File Path" <- w2320
                    n942 = local write "Slopes History File Path"(w2328) -> ()
                    n943 = global write "Kpro Globals.vi" "Flow Slope"(w2349) -> ()
                    n944 = Bundle By Name(cluster=w2351, "String Pot Slope"=w2350, "Flow Slope"=w2349, "Up Hole Pressure Slope"=w2348) -> (w2341:T1)
                    n945 = global write "Kpro Globals.vi" "Pressure \nSlope"(w2348) -> ()
                    n946 = global write "Kpro Globals.vi" "String Pot \nSlope"(w2350) -> ()
                    n947 = local write "Slopes File Path"(w2329) -> ()
                    n948 = call-poly <userlib>:"Strip Path__ogtk.vi"("path"=w2320) -> ("name"=w2325:string)  [unwired: 1 out]
                    n949 = String Length(string=w2325) -> (length=w2337:i32)
                    n950 = Concatenate Strings(w2319, w2325) -> (w2323:string)
                    n951 = Equal To 0?(x=w2337) -> (x = 0?=w2324:bool)
                    n952 = local write "Input Variables and Slopes"(w2341) -> ()
                    n953 = Or(x=w2324, y=w2324) -> ()  [unwired: 1 out]
                    n954 = String To Path(string=w2323) -> (path=w2322:path)
                    "appended path" <- w2322
                    n955 = stacked-sequence {
                      tunnel: w2322 -> [_ _ _ _ _ _ _ _ _]
                      frame #0 {
                        n956 = local read "appended path"() -> (w2360:path)
                        n957 = Path To String(path=w2360) -> (string=w2359:string)
                        n958 = Concatenate Strings(w2359, "_KPROcumulative.csv") -> (w2362:string)
                        n959 = String To Path(string=w2362) -> (path=w2356:path)
                        "KPRO Cumulative Output File Path" <- w2356
                        n960 = call-poly <vilib>:"Write Delimited Spreadsheet.vi"("file path (dialog if empty)"=w2356, "1D data"=string[] ["Measurement Time", "Current Absolute Depth", "Depth Rate", "Flow", "Feet of Stainless Steel Used", "In line Pressure Sensor", "IK", "Corrected Headloss", "Atmospheric Pressure (global)", "Depth to Water Table (global)", "Height of Box (global)", "Resevoir Pressure (global)", "Seconds since Jan 1 1904", "Downhole Pressure Sensor"], "append to file? (new file:F)"=TRUE, "delimiter (\\t)"="," ("delimiter (\\t)")) -> ()  [unwired: 10 in, 2 out]
                      }
                      frame #1 {
                        n961 = local read "KPRO SessionOutput File Path"() -> (w2363:path)
                        n962 = call-poly <vilib>:"Write Delimited Spreadsheet.vi"("file path (dialog if empty)"=w2363, "1D data"=string[] ["Measurement Time", "Current Absolute Depth", "Depth Rate", "Flow", "Feet of Stainless Steel Used", "In line Pressure Sensor", "IK", "Corrected Headloss", "Atmospheric Pressure (global)", "Depth to Water Table (global)", "Height of Box (global)", "Resevoir Pressure (global)", "Seconds since Jan 1 1904", "Downhole Pressure Sensor"], "append to file? (new file:F)"=TRUE, "delimiter (\\t)"="," ("delimiter (\\t)")) -> ()  [unwired: 10 in, 2 out]
                      }
                      frame #2 {
                        n963 = local read "appended path"() -> (w2370:path)
                        n964 = Path To String(path=w2370) -> (string=w2371:string)
                        n965 = Concatenate Strings(w2371, "_SondeData.csv" ("string")) -> (w2372:string)
                        n966 = String To Path(string=w2372) -> (path=w2367:path)
                        "Sonde Output File Path" <- w2367
                        n967 = local write "Sonde Output File Path"(w2367) -> ()
                        n968 = call "convert sonde cluster to spreadsheet array.vi"() -> ("sonde labels"=w2369:string[])  [unwired: 8 in, 3 out]
                        n969 = call-poly <vilib>:"Write Delimited Spreadsheet.vi"("file path (dialog if empty)"=w2367, "1D data"=w2369, "delimiter (\\t)"="," ("delimiter (\\t)")) -> ()  [unwired: 11 in, 2 out]
                      }
                      frame #3 {
                        n970 = local read "appended path"() -> (w2375:path)
                        n971 = Path To String(path=w2375) -> (string=w2376:string)
                        n972 = Concatenate Strings(w2376, "_Groundwater Profiling Log.xlsx" ("string")) -> (w2377:string)
                        n973 = String To Path(string=w2377) -> (path=w2374:path)
                        n974 = local write "Excel report file path"(w2374) -> ()
                      }
                      frame #4 {
                        n975 = local read "appended path"() -> (w2385:path)
                        n976 = Path To String(path=w2385) -> (string=w2379:string)
                        n977 = Concatenate Strings(w2379, "_Sample failure.csv" ("new ending (none)")) -> (w2383:string)
                        n978 = String To Path(string=w2383) -> (path=w2380:path)
                        "Sonde Recording Failure Path" <- w2380
                        "Sonde Recording Error file" <- w2380
                        n979 = call-poly <vilib>:"Write Delimited Spreadsheet.vi"("file path (dialog if empty)"=w2380, "1D data"=string[] ["Time", "Head Pressure", "Depth", "Select Entry Value", "Select Entry String"], "append to file? (new file:F)"=TRUE, "delimiter (\\t)"="," ("delimiter (\\t)")) -> ()  [unwired: 10 in, 2 out]
                      }
                      frame #5 {
                        n980 = local read "appended path"() -> (w2393:path)
                        n981 = Path To String(path=w2393) -> (string=w2388:string)
                        n982 = Concatenate Strings(w2388, "_IK failure.csv" ("new ending (none)")) -> (w2390:string)
                        n983 = String To Path(string=w2390) -> (path=w2387:path)
                        "IK Recording Error file" <- w2387
                        n984 = local write "Sonde IK Recording Failure Path"(w2387) -> ()
                        n985 = call-poly <vilib>:"Write Delimited Spreadsheet.vi"("file path (dialog if empty)"=w2387, "1D data"=string[] ["Time", "Head Pressure", "Depth", "Select Entry Value", "Select Entry String"], "append to file? (new file:F)"=TRUE, "delimiter (\\t)"="," ("delimiter (\\t)")) -> ()  [unwired: 10 in, 2 out]
                      }
                      frame #6 {
                        n986 = local read "appended path"() -> (w2398:path)
                        n987 = Path To String(path=w2398) -> (string=w2396:string)
                        n988 = Concatenate Strings(w2396, "_DHT Data.csv" ("new ending (none)")) -> (w2397:string)
                        n989 = String To Path(string=w2397) -> (path=→"Down hole Pressure Transducer CSV data  path":path)
                      }
                      frame #7 {
                        n990 = local read "appended path"() -> (w2400:path)
                        n991 = Path To String(path=w2400) -> (string=w2401:string)
                        n992 = Concatenate Strings(w2401, "_Static Ik.csv" ("string")) -> (w2403:string)
                        n993 = String To Path(string=w2403) -> (path=w2402:path)
                        n994 = local write "Static IK path"(w2402) -> ()
                      }
                      frame #8 {
                        n995 = Build Array("Profile ID   " ("string"), "Depth    " ("string"), "Flow " ("string"), "Ik    " ("string")) -> (w2406:string[])
                        n996 = call-poly <vilib>:"Write Delimited Spreadsheet.vi"("file path (dialog if empty)"="Static IK path", "1D data"=w2406, "append to file? (new file:F)"=TRUE, "delimiter (\\t)"="," ("delimiter (\\t)")) -> ()  [unwired: 10 in, 2 out]
                      }
                    }
                    n997 = Concatenate Strings(w2323, "_KPROsession.csv") -> (w2326:string)
                    n998 = String To Path(string=w2326) -> (path=w2342:path)
                    "KPRO SessionOutput File Path" <- w2342
                    n999 = call <vilib>:"Check if File or Folder Exists.vi"("path"=w2342) -> ("file or folder exists?"=w2334:bool, "dup path"=w2336:path)  [unwired: 8 in, 1 out]
                    n1000 = And(x=w2334, y=w2343) -> (x .and. y?=w2335:bool)
                    n1001 = case shown="True" w2335 {
                      selector: w2335 -> [_ w2419]
                      tunnel: w2336 -> [_ w2430]
                      tunnel: w2341 -> [w2415 w2425]
                      tunnel: [w2415 w2424] -> w2340
                      tunnel: w2339 -> [w2414 w2420]
                      tunnel: [w2414 w2420] -> w2332
                      tunnel: w2331 -> [w2413 w2418]
                      tunnel: [w2413 w2417] -> w2330
                      frame False {
                      }
                      frame True {
                        n1002 = local read "Culmulative Graph Cluster"() -> (w2429:T20)
                        n1003 = call "Get_KPRO_data_from_file 2016.vi"("Output File KPRO Test"=w2430) -> ("Last_height_of_box"=w2422:dbl, "Last_depth_to_water"=w2423:dbl, "Last_depth"=w2421:dbl, "Output_array"=w2416:sgl[][])  [unwired: 7 in]
                        "Cumulative_data_from_file" <- w2416
                        n1004 = Bundle By Name(cluster=w2425, "Depth to Water Table"=w2423, "Height of Sample Box"=w2422) -> (w2424:T1)
                        n1005 = Bundle By Name(cluster=w2418, "Absolute Depth In"=w2421, "Current Absolute Depth"=w2421) -> (w2417:T18)
                        n1006 = call "Array to Plot 2016.vi"("Input Cumulative Array"=w2416) -> ("Cumulative - Depth vs.Drive Rate"=w2426:cluster{dbl[], dbl[]}, "Cumulative - Depth vs. Ik"=w2427:cluster{dbl[], dbl[]})  [unwired: 3 in, 4 out]
                        n1007 = Bundle By Name(cluster=w2429, "Cumulative - Depth vs. Ik"=w2427, "Cumulative - Depth vs. Drive Rate"=w2426) -> (w2428:T20)
                        n1008 = local write "Culmulative Graph Cluster"(w2428) -> ()
                        n1009 = local write "Input Variables and Slopes"(w2424) -> ()
                        "Cumulative_data_ready" <- w2419
                      }
                    }
                  }
                }
                n1010 = local write "Initialization"(2 ("Initialization")) -> ()
              }
              frame #3 {
                # "Take offset and put\n into Pressure VI."
                n1011 = local write "Initialization"(3 ("Initialization")) -> ()
                n1012 = local read "Groundwater Header"() -> (w2438:T11)
                n1013 = global read "Kpro Globals.vi" "Pressure Offset"() -> (w2431:dbl)
                n1014 = local read "Input Variables and Slopes"() -> (w2436:T1)
                n1015 = Unbundle By Name(w2438) -> ("Atmospheric Pressure"=w2435:string)
                n1016 = case shown="False" TRUE {
                  tunnel: "ATMOSPHERIC PRESSURE READING\n\nHold Kpro effluent facing up and level with the pressure transducer.\nTurn on Kpro water, turn off when water flows with no air bubbles.\n\nPress OK when the reading equilibrates." ("message") -> [_ w2472]
                  tunnel: [w2463 w2471] -> w2453
                  tunnel: [w2462 w2465] -> w2450
                  tunnel: w2447 -> [_ w2470]
                  tunnel: w2446 -> [w2460 w2469]
                  tunnel: [w2461 w2468] -> w2445
                  tunnel: [w2457 w2467] -> w2440
                  tunnel: [w2460 w2466] -> w2439
                  tunnel: w2436 -> [w2462 w2465]
                  tunnel: w2435 -> [w2458 _]
                  tunnel: [w2456 w2464] -> w2432
                  tunnel: w2431 -> [w2456 w2464]
                  frame False {
                    n1017 = local read "Sensor Voltage Cluster"() -> (w2463:T10)
                    n1018 = Unbundle By Name(w2462) -> ("Up Hole Pressure Slope"=w2461:dbl)
                    n1019 = Scan From String(input string=w2458, default 1=35.0 ("default value 1")) -> (output 1=w2457:dbl)  [unwired: 3 in, 3 out]
                  }
                  frame True {
                    n1020 = local read "Sensor Voltage Cluster"() -> (w2471:T10)
                    n1021 = Unbundle By Name(w2465) -> ("Up Hole Pressure Slope"=w2468:dbl)
                    n1022 = call "Up Hole PRESSURE_CAL 2016.vi"("Pressure Offset"=w2464, "Descriptions"=w2470, "Array in"=w2469, "Pressure \nSlope"=w2468, "Sensor Cluster"=w2471, "Prompt_IN"=w2472) -> ("PRESSURE\nFt of water"=w2467:dbl, "Array out"=w2466:refnum<k24>[])  [unwired: 4 in]
                    "Up Hole Pressure Offset" <- w2464
                  }
                }
                n1023 = Equal?(x=w2435, y="") -> ()  [unwired: 1 out]
                n1024 = local read "Corrected\n Pressure \nCluster"() -> (w2452:T21)
                n1025 = Bundle By Name(cluster=w2450, "Atmospheric Pressure"=w2440, "Up Hole  Pressure Offset"=w2432) -> (w2449:T1)
                n1026 = global write "Kpro Globals.vi" "Atmospheric Pressure"(w2440) -> ()
                n1027 = Format Into String(w2440) -> (resulting string=w2441:string)  [unwired: 3 in, 1 out]
                n1028 = call "up hole Pressure 2016.vi"("Sensor Cluster"=w2453, "Pressure Offset"=w2440, "Array in"=w2439, "Pressure \nSlope"=w2445, "Descriptions"=w2447, "Zero Pressure\n(F = leave as is)"=TRUE) -> ("Array out"=w2448:refnum<k24>[], "Uphole Pressure"=w2433:dbl, "Sensor Cluster 2"=w2443:T10)  [unwired: 6 in, 1 out]
                n1029 = Bundle By Name(cluster=w2438, "Atmospheric Pressure"=w2441) -> (w2442:T11)
                n1030 = Bundle By Name(cluster=w2452, "Up hole Corrected Pressure"=w2433) -> (w2451:T21)
                n1031 = local write "Sensor Voltage Cluster"(w2443) -> ()
                n1032 = local write "Input Variables and Slopes"(w2449) -> ()
                n1033 = local write "Groundwater Header"(w2442) -> ()
                n1034 = local write "Corrected\n Pressure \nCluster"(w2451) -> ()
                n1035 = local write "Uphole Pressure"(w2433) -> ()
              }
              frame #4 {
                n1036 = flat-sequence {
                  tunnel: w2475 -> [w2484]
                  tunnel: w2474 -> [w2483]
                  frame #0 {
                    n1037 = local read "Input Variables and Slopes"() -> (w2482:T1)
                    n1038 = Unbundle By Name(w2482) -> ("Up Hole Pressure Slope"=w2481:dbl)
                    n1039 = local read "Sensor Voltage Cluster"() -> (w2487:T10)
                    n1040 = global read "Kpro Globals.vi" "Pressure Offset"() -> (w2480:dbl)
                    n1041 = call "Up Hole PRESSURE_CAL 2016.vi"("Pressure Offset"=w2480, "Descriptions"=w2483, "Array in"=w2484, "Pressure \nSlope"=w2481, "Sensor Cluster"=w2487, "Prompt_IN"="CHECK RESERVOIR PRESSURE\n\nTurn on Kpro. Unplug Kpro Out quick connect from sample box.\nReservoir pressure should be 69.2 +/- 5%(65.7 - 72.7).\n\nPress OK when the reading equilibrates within range." ("message")) -> ("PRESSURE\nFt of water"=w2477:dbl)  [unwired: 4 in, 1 out]
                    n1042 = local read "Groundwater Header"() -> (w2479:T11)
                    n1043 = Format Into String(w2477) -> (resulting string=w2476:string)  [unwired: 3 in, 1 out]
                    n1044 = global write "Kpro Globals.vi" "Reservoir Pressure"(w2477) -> ()
                    n1045 = Bundle By Name(cluster=w2482, "Reservoir Pressure"=w2477) -> (w2485:T1)
                    n1046 = Bundle By Name(cluster=w2479, "KPRO N2 Pressure"=w2476) -> (w2478:T11)
                    n1047 = local write "Input Variables and Slopes"(w2485) -> ()
                    n1048 = local write "Groundwater Header"(w2478) -> ()
                  }
                }
                n1049 = local write "Initialization"(5 ("Initialization")) -> ()
              }
              frame #5 {
                n1050 = flat-sequence {
                  frame #0 {
                    n1051 = local read "Input Depths \nand Parameters Cluster"() -> (w2492:T17)
                    n1052 = Unbundle By Name(w2492) -> ("Start Depth"=w2489:sgl)
                    n1053 = call "prompt_and_enter_value 2016.vi"("prompt_IN"="ENTER START DEPTH", "Enter value"=w2489) -> ("Numeric"=w2494:dbl)  [unwired: 9 in]
                    n1054 = Absolute Value(x=w2494) -> (abs(x)=w2493:dbl)
                    n1055 = Negate(x=w2493) -> (-x=w2490:dbl)
                    n1056 = Bundle By Name(cluster=w2492, "Start Depth"=w2490) -> (w2491:T17)
                    n1057 = local write "Input Depths \nand Parameters Cluster"(w2491) -> ()
                  }
                }
                n1058 = local write "Initialization"(6 ("Initialization")) -> ()
              }
              frame #6 {
                n1059 = local write "Initialization"(7 ("Initialization")) -> ()
                n1060 = local read "Input Variables and Slopes"() -> (w2500:T1)
                n1061 = Unbundle By Name(w2500) -> ("Height of Sample Box"=w2498:dbl)
                n1062 = call "prompt_and_enter_value 2016.vi"("prompt_IN"="HEIGHT FROM GROUND SURFACE TO SAMPLE BOX\n\nMeasure the vertical distance between the ground surface and the pressure transducer." ("prompt"), "Enter value"=w2498) -> ("Numeric"=w2497:dbl)  [unwired: 9 in]
                n1063 = Bundle By Name(cluster=w2500, "Height of Sample Box"=w2497) -> (w2499:T1)
                n1064 = global write "Kpro Globals.vi" "height_of_box"(w2497) -> ()
                n1065 = local write "Input Variables and Slopes"(w2499) -> ()
              }
              frame #7 {
                n1066 = local write "Initialization"(8 ("Initialization")) -> ()
                n1067 = flat-sequence {
                  frame #0 {
                    n1068 = local read "Input Variables and Slopes"() -> (w2505:T1)
                    n1069 = Unbundle By Name(w2505) -> ("Depth to Water Table"=w2506:dbl)
                    n1070 = call "prompt_and_enter_value 2016.vi"("prompt_IN"="DEPTH TO WATER TABLE\n\nEnter the depth to the water table." ("prompt"), "Enter value"=w2506) -> ("Numeric"=w2508:dbl)  [unwired: 9 in]
                    n1071 = Absolute Value(x=w2508) -> (abs(x)=w2507:dbl)
                    n1072 = Negate(x=w2507) -> (-x=w2504:dbl)
                    n1073 = global write "Kpro Globals.vi" "Depth to Water Table"(w2504) -> ()
                    n1074 = Bundle By Name(cluster=w2505, "Depth to Water Table"=w2504) -> (w2503:T1)
                    n1075 = local write "Input Variables and Slopes"(w2503) -> ()
                  }
                }
              }
              frame #8 {
                n1076 = stacked-sequence {
                  tunnel: [w2513 _] -> _
                  tunnel: w2511 -> [w2517 w2536]
                  tunnel: w2512 -> [w2516 w2533]
                  tunnel: w2511 -> [_ w2534]
                  frame #0 {
                    # "Set to raw pressure mode"
                    n1077 = local read "Input Variables and Slopes"() -> (w2514:T1)
                    n1078 = local read "Sensor Voltage Cluster"() -> (w2521:T10)
                    n1079 = Unbundle By Name(w2514) -> ("Up Hole Pressure Slope"=w2513:dbl)
                    n1080 = local read "Corrected\n Pressure \nCluster"() -> (w2519:T21)
                    n1081 = call "up hole Pressure 2016.vi"("Sensor Cluster"=w2521, "Pressure Offset"=0.0, "Array in"=w2516, "Pressure \nSlope"=w2513, "Descriptions"=w2517, "Zero Pressure\n(F = leave as is)"=TRUE) -> ("Uphole Pressure"=w2520:dbl)  [unwired: 6 in, 3 out]
                    n1082 = Bundle By Name(cluster=w2519, "Up hole Corrected Pressure"=w2520) -> (w2518:T21)
                    n1083 = local write "Corrected\n Pressure \nCluster"(w2518) -> ()
                    n1084 = local read "Input Variables and Slopes 2"() -> (w2515:T1)
                    n1085 = Unbundle By Name(w2515) -> ()  [unwired: 1 out]
                  }
                  frame #1 {
                    # "adjust for 1 foot head"
                    # "Take offset and put\n into Pressure VI."
                    n1086 = local read "Input Variables and Slopes"() -> (w2528:T1)
                    n1087 = Unbundle By Name(w2528) -> ("Up Hole Pressure Slope"=w2527:dbl)
                    n1088 = local read "Sensor Voltage Cluster"() -> (w2537:T10)
                    n1089 = global read "Kpro Globals.vi" "Pressure Offset"() -> (w2535:dbl)
                    n1090 = local read "Corrected\n Pressure \nCluster"() -> (w2525:T21)
                    n1091 = call "Up Hole PRESSURE_CAL 2016.vi"("Pressure Offset"=w2535, "Descriptions"=w2534, "Array in"=w2533, "Pressure \nSlope"=w2527, "Sensor Cluster"=w2537, "Prompt_IN"="ZERO TO GROUND SURFACE\n\nFill a grad cylinder to 750mL.\nPlace it on the ground at the profile location.\nImmerse the Kpro effluent and turn on Kpro flow.\nTurn off after water is flowing with no bubbles\nand the water has reached 800mL (1 foot).\n\nPress OK when the reading equilibrates." ("message")) -> ("PRESSURE\nFt of water"=w2538:dbl)  [unwired: 4 in, 1 out]
                    n1092 = Decrement(x=w2538) -> (x-1=w2532:dbl)
                    n1093 = call "up hole Pressure 2016.vi"("Sensor Cluster"=w2537, "Pressure Offset"=w2532, "Array in"=w2533, "Pressure \nSlope"=w2527, "Descriptions"=w2536, "Zero Pressure\n(F = leave as is)"=TRUE) -> ("Uphole Pressure"=w2524:dbl, "Pressure Offset 2"=w2529:dbl)  [unwired: 6 in, 2 out]
                    n1094 = Bundle By Name(cluster=w2525, "Up hole Corrected Pressure"=w2524) -> (w2526:T21)
                    n1095 = local read "Input Variables and Slopes"() -> (w2531:T1)
                    n1096 = Bundle By Name(cluster=w2531, "Up Hole  Pressure Offset"=w2529) -> (w2530:T1)
                    n1097 = local write "Input Variables and Slopes"(w2530) -> ()
                    n1098 = local write "Corrected\n Pressure \nCluster"(w2526) -> ()
                  }
                }
                n1099 = local write "Initialization"(9 ("Initialization")) -> ()
              }
              frame #9 {
                n1100 = local write "Initialization"(10 ("Initialization")) -> ()
                n1101 = local read "Cumulative_data_ready"() -> (w2545:bool)
                n1102 = case shown="True" w2545 {
                  tunnel: w2544 -> [w2546 _]
                  tunnel: [w2546 w2547] -> w2543
                  frame False {
                  }
                  frame True {
                    n1103 = local write "Cumulative_data_ready"(FALSE ("Get_KPRO_data")) -> ()
                    n1104 = local read "Cumulative_data_from_file"() -> (w2547:sgl[][])
                  }
                }
              }
            }
            n1105 = flat-sequence {
              tunnel: "Read String Pot" -> [_]
              tunnel: [w2586] -> w2241
              tunnel: w2248 -> [w2570]
              tunnel: w2244 -> [w2571]
              frame #0 {
                w2576 = 0.0
                w2577 = TRUE
                # "Initialize Incrementer if using hand incrementer,\nDon't use Debug,\nPut use string pot into shift register first pass to avoid allowing\na change in which method is the source of the depth reading."
                n1106 = global write "Global_SIM_switch.vi" "enable_kpro_file"("enable_kpro_file") -> ()
                n1107 = global write "Global_SIM_switch.vi" "Simulate AD6B"("Simulate AD6B") -> ()
                n1108 = global write "Global_SIM_switch.vi" "enable_slug_file"("enable_slug_file") -> ()
                n1109 = local read "Input Variables and Slopes"() -> (w2584:T1)
                n1110 = global write "Global_SIM_switch.vi" "enable_IKMGS_file"("enable_IKMGS_file") -> ()
                n1111 = Unbundle By Name(w2584) -> ("String Pot Slope"=w2583:dbl, "Up Hole Pressure Slope"=w2579:dbl)  [unwired: 1 out]
                n1112 = local read "Sensor Voltage Cluster"() -> (w2578:T10)
                n1113 = local read "Descriptions"() -> (w2569:string[])
                n1114 = local read "Sensor Voltage Cluster"() -> (w2585:T10)
                n1115 = call "In-Line-Pressure 2016.vi"("Zero Pressure\n(F = leave as is)"=w2577, "In-Line Pressure Slope"=w2579, "Sensor Voltages Cluster"=w2578, "In-Line Pressure Offset"=w2576) -> ("Pressure"=w2580:dbl)  [unwired: 7 in]
                n1116 = call "up hole Pressure 2016.vi"("Sensor Cluster"=w2578, "Pressure Offset"=w2576, "Array in"=w2571, "Pressure \nSlope"=w2579, "Descriptions"=w2569, "Zero Pressure\n(F = leave as is)"=w2577) -> ("Array out"=w2568:refnum<k24>[], "Uphole Pressure"=w2565:dbl)  [unwired: 6 in, 2 out]
                n1117 = Bundle By Name(cluster="Corrected\n Pressure \nCluster", "Up hole Corrected Pressure"=w2565, "Down hole Corrected Pressure"=w2580) -> (w2581:T21)
                n1118 = call "depth read from string pot 2016.vi"("Descriptions"=w2569, "error in (no error)"=w2570, "String Pot \nSlope"=w2583, "Array in"=w2568, "Sensor Cluster In"=w2585) -> ("Depth"=w2587:dbl)  [unwired: 11 in, 3 out]
                n1119 = local read "Sample Sheet Data Row Cluster 2"() -> (w2567:T2)
                n1120 = local write "Corrected\n Pressure \nCluster"(w2581) -> ()
                n1121 = flat-sequence {
                  tunnel: w2587 -> [w2589]
                  tunnel: [w2588] -> w2586
                  frame #0 {
                    w2590 = 15  # Filter Size
                    # "Functional Global in \nBoxcar Integrator\nInitialize filter array to \ncurrent string pot value"
                    n1122 = call "Boxcar filter2016.vi"("Initialize"=TRUE, "Filter Size"=w2590, "Filter Input"=w2589) -> ("Filter Output"=w2588:dbl)
                  }
                }
                n1123 = Bundle By Name(cluster=w2567, "Head\nPressure"=w2565) -> (w2566:T2)
                n1124 = local write "Sample Sheet Data Row Cluster 2"(w2566) -> ()
              }
            }
            n1125 = flat-sequence {
              tunnel: [w2552] -> w2249
              tunnel: [w2551] -> w2242
              tunnel: w2241 -> [w2549]
              tunnel: [w2549] -> w2238
              frame #0 {
                n1126 = local read "Input Depths \nand Parameters Cluster"() -> (w2550:T17)
                n1127 = Unbundle By Name(w2550) -> ("Start Depth"=w2553:sgl)
                n1128 = Less Or Equal To 0?(x=w2553) -> (x <= 0?=w2555:bool)
                n1129 = Negate(x=w2553) -> (-x=w2554:sgl)
                n1130 = Select(t=w2553, s=w2555, f=w2554) -> (s? t:f=w2551:sgl)
                n1131 = Bundle By Name(cluster=w2550, "Abs Start Depth"=w2551, "Current Depth"=w2549) -> (w2552:T17)
                n1132 = local write "Input Depths \nand Parameters Cluster"(w2552) -> ()
              }
            }
            n1133 = flat-sequence {
              tunnel: [w2562] -> w2251
              frame #0 {
                n1134 = Tick Count (ms)() -> (millisecond timer value=w2564:u32)
                n1135 = Divide(x=w2564, y=u32 1000) -> (x/y=w2562:dbl)
              }
            }
            n1136 = flat-sequence {
              tunnel: [w2557] -> w2250
              tunnel: w2251 -> [w2560]
              tunnel: [w2559] -> _
              tunnel: w2242 -> [w2559]
              tunnel: w2238 -> [w2558]
              tunnel: w2235 -> [w2556]
              frame #0 {
                n1137 = Bundle By Name(cluster=w2556, "Absolute Depth In"=w2559, "Previous Relative Depth"=w2558, "Current Relative Depth"=w2558, "First Relative Depth"=w2558, "Current Absolute Depth"=w2559, "Last Filed Depth"=0.0, "Current Measurement Time"=w2560, "Previous Measurement Time"=w2560, "First Absolute Depth"=w2559) -> (w2557:T18)
              }
            }
          }
          frame "Acq. DAQ data" {
            n1138 = flat-sequence {
              tunnel: w2642 -> [w2659]
              tunnel: w2641 -> [w2658]
              tunnel: [w2655] -> w2640
              frame #0 {
                n1139 = local read "Descriptions"() -> (w2656:string[])
                n1140 = local read "Sensor  Real \nMeasurements"() -> (w2654:T7)
                n1141 = local read "Input Variables and Slopes"() -> (w2652:T1)
                n1142 = call "Measure DAQ Voltages.vi"("error in (no error)"=w2658, "Descriptions"=w2656, "Array in"=w2659) -> ("Raw Voltages"=→"Raw Voltages":dbl[], "Array out"=w2655:refnum<k24>[], "Sensor Cluster"=w2651:T10)  [unwired: 6 in]
                "Sensor Voltage Cluster" <- w2651
                n1143 = call "convert sensor voltage to real measurements.vi"("Input Variables and Slopes"=w2652, "Sensor  Real Measurements in"=w2654, "Sensor Cluster"=w2651) -> ("Sensor  Real Measurements out"=w2653:T10)  [unwired: 8 in]
                n1144 = local write "Sensor  Real \nMeasurements"(w2653) -> ()
              }
            }
          }
          frame "Exit" {
            n1145 = case shown="No Error" w2673 {
              tunnel: w2669 -> [w2706 _]
              tunnel: w2673 -> [w2705 w2717]
              tunnel: [w2704 w2717] -> w2671
              frame No Error {
                n1146 = for {
                  shift-right: [w2708] -> w2704
                  shift-left: w2705 -> [w2709]
                  tunnel: w2706 -> [w2707] mode=indexing
                  n1147 = while {
                    shift-right: [w2716] -> w2711
                    shift-left: w2709 -> [w2714]
                    shift-right: [w2715] -> w2710
                    shift-left: w2707 -> [w2713]
                    stop <- w2712 stop-if-true
                    n1148 = call <vilib>:"ULx Is Task Done.vi"("task in"=w2713, "error in"=w2714) -> ("task out"=w2715:refnum<k24>, "task done?"=w2712:bool, "error out"=w2716:errorcluster)  [unwired: 11 in]
                  }
                  n1149 = call <vilib>:"ULx Clear Task.vi"("task in"=w2710, "error in"=w2711) -> ("error out"=w2708:errorcluster)  [unwired: 13 in]
                }
              }
              frame Error {
              }
            }
            n1150 = flat-sequence {
              tunnel: [w2723] -> w2680
              tunnel: [w2722] -> w2681
              tunnel: w2661 -> [w2720]
              tunnel: w2660 -> [w2719]
              frame #0 {
                n1151 = local read "Excel report file path"() -> (w2718:path)
                n1152 = call-dynamic "Save Report to File.vi"("report in"=w2719, "report file path"=w2718, "prompt to replace? (F)"=FALSE, "error in (no error)"=w2720) -> ("report out"=w2723:refnum<class "NI_report.lvclass">, "error out"=w2722:errorcluster)  [unwired: 10 in]
              }
            }
            n1153 = call <userlib>:"Wait (ms)__ogtk.vi"("error in (no error)"=w2681, "milliseconds to wait"=u32 5) -> ("error out"=w2682:errorcluster)  [unwired: 8 in, 1 out]
            n1154 = flat-sequence {
              tunnel: w2682 -> [w2692]
              tunnel: w2680 -> [w2690]
              tunnel: [w2688] -> w2674
              frame #0 {
                (unwired) FALSE ("Write Ini")
                n1155 = call-dynamic "Dispose Report.vi"("report in"=w2690, "save changes? (F)"=FALSE, "error in (no error)"=w2692) -> ("error out"=w2687:errorcluster)  [unwired: 12 in]
                n1156 = case shown="False" "Save Configuration File?" {
                  tunnel: [errorcluster {"status"=FALSE, "code"=0, "source"=""} ("error IO") w2701] -> w2689
                  frame False {
                  }
                  frame True {
                    n1157 = local read "Config File Path"() -> (w2700:path)
                    n1158 = call <vilib>:"Open Config Data.vi"("create file if necessary (T)"=TRUE ("Read Ini"), "configuration file path"=w2700) -> ("error out"=w2698:errorcluster, "refnum"=w2695:T22)  [unwired: 7 in, 1 out]
                    n1159 = control-ref of="This VI"() -> (w2694:refnum<vi>)
                    n1160 = call <userlib>:"Write Panel to INI__ogtk.vi"("error in (no error)"=w2698, "VI ref"=w2694, "refnum"=w2695) -> ("error out"=w2697:errorcluster, "refnum out"=w2696:T22)  [unwired: 7 in]
                    n1161 = call <vilib>:"Clear Errors.vi"("error in (no error)"=w2697) -> ("error out"=w2703:errorcluster)  [unwired: 5 in, 1 out]
                    n1162 = call <vilib>:"Close Config Data.vi"("error in (no error)"=w2703, "refnum"=w2696) -> ("error out"=w2702:errorcluster)  [unwired: 8 in, 1 out]
                    n1163 = Merge Errors(w2702, w2697) -> (w2701:errorcluster)
                  }
                }
                n1164 = Merge Errors(w2689, w2687) -> (w2688:errorcluster)
              }
            }
            n1165 = flat-sequence {
              tunnel: [w2684] -> w2672
              tunnel: [w2685] -> w2670
              tunnel: w2671 -> [w2685]
              frame #0 {
                w2684 = TRUE ("aborted?")
                "Stop 2" <- w2684
              }
            }
          }
          frame "Create Excel Files" {
            n1166 = flat-sequence {
              tunnel: [w2800] -> _
              tunnel: [w2799] -> _
              tunnel: [w2786] -> _
              tunnel: [w2797] -> _
              tunnel: [w2796] -> w2729
              tunnel: [w2795] -> w2728
              tunnel: [w2793] -> _
              tunnel: w2730 -> [w2784]
              frame #0 {
                n1167 = control-ref of="last occupied cell's name"() -> (w2792:refnum<vi>)
                n1168 = control-ref of="Current Sample Sheet"() -> (w2790:refnum<vi>)
                n1169 = control-ref of="row max value"() -> (w2791:refnum<vi>)
                n1170 = call "setup excel worksheet.vi"("Last Occupied cell Name reference"=w2792, "Row Max Value Reference"=w2791, "Current Sample Sheet Reference"=w2790, "template file path"="template file path", "Excel report file path"="Excel report file path", "error in (no error)"=w2784, "Header path"="Header path", "Open Excel Files"=TRUE) -> ("subarray"=→"subarray":string[][], "column max value"=→"column max value":i32, "row max value"=→"row max value":i32, "Column of Volume"=w2793:i32, "Worksheet Names"=w2786:string[], "NI_report out"=w2796:refnum<class "NI_report.lvclass">, "Columns"=w2799:i32[], "Number of Sample Sheets"=w2800:i32, "Select Worksheet Index"=w2797:i32, "error out"=w2795:errorcluster)  [unwired: 2 in]
                "Worksheet Names" <- w2786
                "NI_report out" <- w2796
                "Number of Sample Sheets" <- w2800
                "Select Worksheet Index" <- w2797
                "Columns" <- w2799
                "Column of Volume" <- w2793
              }
            }
            n1171 = flat-sequence {
              tunnel: [w2782] -> w2725
              tunnel: w2728 -> [w2776]
              tunnel: [w2775] -> w2727
              tunnel: w2729 -> [w2774]
              frame #0 {
                w2781 = "Groundwater Profile Log" ("Worksheet Name in")
                n1172 = local read "Worksheet Names"() -> (w2779:string[])
                n1173 = local write "Current Sample Sheet"(w2781) -> ()
                n1174 = call "find and open select worksheet.vi"("Worksheet Names"=w2779, "error in (no error)"=w2776, "milliseconds to wait"=u32 100, "Worksheet Name in"=w2781, "NI_report in"=w2774) -> ("error out"=w2778:errorcluster, "NI_report out"=w2777:refnum<class "NI_report.lvclass">)  [unwired: 4 in, 1 out]
                n1175 = call "groundwater log header.vi"("Worksheet Names"=w2779, "Groundwater Header"="Groundwater Header", "error in (no error)"=w2778, "NI_report in"=w2777) -> ("error out"=w2775:errorcluster, "NI_report out"=w2782:refnum<class "NI_report.lvclass">)  [unwired: 6 in]
              }
            }
            n1176 = flat-sequence {
              tunnel: w2727 -> [w2759]
              tunnel: [w2758] -> w2726
              tunnel: w2725 -> [w2757]
              tunnel: [w2756] -> w2724
              frame #0 {
                # "Disabled"
                n1177 = call "open select sample sheet.vi"("error in (no error)"=w2759, "input 1"=0 ("Active Sample Sheet"), "NI_report in"=w2757) -> ("error out"=w2755:errorcluster, "Current Sample Sheet"=w2754:string, "NI_report out"=w2753:refnum<class "NI_report.lvclass">)  [unwired: 6 in]
                n1178 = flat-sequence {
                  tunnel: [w2772] -> w2756
                  tunnel: [w2771] -> _
                  tunnel: w2755 -> [w2770]
                  tunnel: [w2763] -> w2758
                  tunnel: w2754 -> [w2761]
                  tunnel: w2753 -> [w2760]
                  frame #0 {
                    n1179 = call "get sample sheet data cells.vi"("error in (no error)"=w2770, "NI_report in"=w2760) -> ("error out"=w2773:errorcluster, "data"=w2768:string[][], "NI_report out"=w2772:refnum<class "NI_report.lvclass">, "left edge output cluster"=w2766:cluster{"row":i32, "column":i32})  [unwired: 5 in, 1 out]
                    n1180 = Array Subset(array=w2768, index (col)=2 ("index")) -> ()  [unwired: 3 in, 1 out]
                    n1181 = call "find last occupied cell.vi"("Active Sheet"=w2761, "Header Rows to remove"=3, "sub array start"=w2766, "error in (no error)"=w2773) -> ("row max value"=w2765:i32, 13:"start of last occupied row"=w2771:cluster{"row":i32, "column":i32}, 14:"start of last occupied row"=w2764:string, "error out"=w2763:errorcluster)  [unwired: 5 in, 3 out]
                    n1182 = local write "row max value"(w2765) -> ()
                    n1183 = local write "last occupied cell's name"(w2764) -> ()
                    n1184 = local write "Sonde Data Array"(T26[] [{"Head"=0.0, "Depth"=0.0, "Time"="19:00", "Cumulative\nVolume"=0.0, "Sp. Conductance"={"Value"=0.506, "%"=0.0, "Tol."=TRUE}, "Dissolved Oxygen"={"Value"=35.14, "%"=0.0, "Tol."=TRUE}, "pH"={"Value"=4.81, "%"=0.0, "Tol."=TRUE}, "ORP"={"Value"=390.0, "%"=0.0, "Tol."=TRUE}, "Temperature"={"Value"=23.86, "%"=0.0, "Tol."=TRUE}, "Salinity"={"Value"=0.24, "%"=0.0, "Tol."=TRUE}, "Final Tol."=TRUE, "Final"=FALSE, "Time 2"=timestamp(0 s since 1904-01-01), "Aux 1"=0.0, "Aux 2"=0.0, "Aux 3"=0.0}, {"Head"=0.0, "Depth"=0.0, "Time"="19:00", "Cumulative\nVolume"=0.0, "Sp. Conductance"={"Value"=0.506, "%"=0.0, "Tol."=TRUE}, "Dissolved Oxygen"={"Value"=35.12, "%"=0.0, "Tol."=TRUE}, "pH"={"Value"=4.81, "%"=0.0, "Tol."=TRUE}, "ORP"={"Value"=390.0, "%"=0.0, "Tol."=TRUE}, "Temperature"={"Value"=23.89, "%"=0.0, "Tol."=TRUE}, "Salinity"={"Value"=0.24, "%"=0.0, "Tol."=TRUE}, "Final Tol."=TRUE, "Final"=FALSE, "Time 2"=timestamp(0 s since 1904-01-01), "Aux 1"=0.0, "Aux 2"=0.0, "Aux 3"=0.0}, {"Head"=0.0, "Depth"=0.0, "Time"="19:00", "Cumulative\nVolume"=0.0, "Sp. Conductance"={"Value"=0.506, "%"=0.0, "Tol."=TRUE}, "Dissolved Oxygen"={"Value"=35.14, "%"=0.0, "Tol."=TRUE}, "pH"={"Value"=4.81, "%"=0.0, "Tol."=TRUE}, "ORP"={"Value"=390.0, "%"=0.0, "Tol."=TRUE}, "Temperature"={"Value"=23.86, "%"=0.0, "Tol."=TRUE}, "Salinity"={"Value"=0.24, "%"=0.0, "Tol."=TRUE}, "Final Tol."=TRUE, "Final"=FALSE, "Time 2"=timestamp(0 s since 1904-01-01), "Aux 1"=0.0, "Aux 2"=0.0, "Aux 3"=0.0}, {"Head"=0.0, "Depth"=0.0, "Time"="", "Cumulative\nVolume"=0.0, "Sp. Conductance"={"Value"=0.0, "%"=0.0, "Tol."=FALSE}, "Dissolved Oxygen"={"Value"=0.0, "%"=0.0, "Tol."=FALSE}, "pH"={"Value"=0.0, "%"=0.0, "Tol."=FALSE}, "ORP"={"Value"=0.0, "%"=0.0, "Tol."=FALSE}, "Temperature"={"Value"=0.0, "%"=0.0, "Tol."=FALSE}, "Salinity"={"Value"=0.0, "%"=0.0, "Tol."=FALSE}, "Final Tol."=FALSE, "Final"=FALSE, "Time 2"=timestamp(0 s since 1904-01-01), "Aux 1"=0.0, "Aux 2"=0.0, "Aux 3"=0.0}, {"Head"=0.0, "Depth"=0.0, "Time"="", "Cumulative\nVolume"=0.0, "Sp. Conductance"={"Value"=0.0, "%"=0.0, "Tol."=FALSE}, "Dissolved Oxygen"={"Value"=0.0, "%"=0.0, "Tol."=FALSE}, "pH"={"Value"=0.0, "%"=0.0, "Tol."=FALSE}, "ORP"={"Value"=0.0, "%"=0.0, "Tol."=FALSE}, "Temperature"={"Value"=0.0, "%"=0.0, "Tol."=FALSE}, "Salinity"={"Value"=0.0, "%"=0.0, "Tol."=FALSE}, "Final Tol."=FALSE, "Final"=FALSE, "Time 2"=timestamp(0 s since 1904-01-01), "Aux 1"=0.0, "Aux 2"=0.0, "Aux 3"=0.0}, {"Head"=0.0, "Depth"=0.0, "Time"="", "Cumulative\nVolume"=0.0, "Sp. Conductance"={"Value"=0.0, "%"=0.0, "Tol."=FALSE}, "Dissolved Oxygen"={"Value"=0.0, "%"=0.0, "Tol."=FALSE}, "pH"={"Value"=0.0, "%"=0.0, "Tol."=FALSE}, "ORP"={"Value"=0.0, "%"=0.0, "Tol."=FALSE}, "Temperature"={"Value"=0.0, "%"=0.0, "Tol."=FALSE}, "Salinity"={"Value"=0.0, "%"=0.0, "Tol."=FALSE}, "Final Tol."=FALSE, "Final"=FALSE, "Time 2"=timestamp(0 s since 1904-01-01), "Aux 1"=0.0, "Aux 2"=0.0, "Aux 3"=0.0}, {"Head"=0.0, "Depth"=0.0, "Time"="", "Cumulative\nVolume"=0.0, "Sp. Conductance"={"Value"=0.0, "%"=0.0, "Tol."=FALSE}, "Dissolved Oxygen"={"Value"=0.0, "%"=0.0, "Tol."=FALSE}, "pH"={"Value"=0.0, "%"=0.0, "Tol."=FALSE}, "ORP"={"Value"=0.0, "%"=0.0, "Tol."=FALSE}, "Temperature"={"Value"=0.0, "%"=0.0, "Tol."=FALSE}, "Salinity"={"Value"=0.0, "%"=0.0, "Tol."=FALSE}, "Final Tol."=FALSE, "Final"=FALSE, "Time 2"=timestamp(0 s since 1904-01-01), "Aux 1"=0.0, "Aux 2"=0.0, "Aux 3"=0.0}, {"Head"=0.0, "Depth"=0.0, "Time"="", "Cumulative\nVolume"=0.0, "Sp. Conductance"={"Value"=0.0, "%"=0.0, "Tol."=FALSE}, "Dissolved Oxygen"={"Value"=0.0, "%"=0.0, "Tol."=FALSE}, "pH"={"Value"=0.0, "%"=0.0, "Tol."=FALSE}, "ORP"={"Value"=0.0, "%"=0.0, "Tol."=FALSE}, "Temperature"={"Value"=0.0, "%"=0.0, "Tol."=FALSE}, "Salinity"={"Value"=0.0, "%"=0.0, "Tol."=FALSE}, "Final Tol."=FALSE, "Final"=FALSE, "Time 2"=timestamp(0 s since 1904-01-01), "Aux 1"=0.0, "Aux 2"=0.0, "Aux 3"=0.0}, {"Head"=0.0, "Depth"=0.0, "Time"="", "Cumulative\nVolume"=0.0, "Sp. Conductance"={"Value"=0.0, "%"=0.0, "Tol."=FALSE}, "Dissolved Oxygen"={"Value"=0.0, "%"=0.0, "Tol."=FALSE}, "pH"={"Value"=0.0, "%"=0.0, "Tol."=FALSE}, "ORP"={"Value"=0.0, "%"=0.0, "Tol."=FALSE}, "Temperature"={"Value"=0.0, "%"=0.0, "Tol."=FALSE}, "Salinity"={"Value"=0.0, "%"=0.0, "Tol."=FALSE}, "Final Tol."=FALSE, "Final"=FALSE, "Time 2"=timestamp(0 s since 1904-01-01), "Aux 1"=0.0, "Aux 2"=0.0, "Aux 3"=0.0}] ("Sonde Data Array")) -> ()
                  }
                }
              }
            }
            n1185 = flat-sequence {
              tunnel: [w2814] -> w2748
              tunnel: [w2813] -> w2749
              tunnel: w2726 -> [w2811]
              tunnel: w2724 -> [w2810]
              frame #0 {
                n1186 = local read "Excel report file path"() -> (w2809:path)
                n1187 = call-dynamic "Save Report to File.vi"("report in"=w2810, "report file path"=w2809, "prompt to replace? (F)"=FALSE, "error in (no error)"=w2811) -> ("report out"=w2814:refnum<class "NI_report.lvclass">, "error out"=w2813:errorcluster)  [unwired: 10 in]
              }
            }
            n1188 = flat-sequence {
              tunnel: w2750 -> [w2808]
              tunnel: w2748 -> [w2806]
              tunnel: [w2805] -> w2742
              frame #0 {
                n1189 = call-dynamic "Dispose Report.vi"("report in"=w2806, "save changes? (F)"=FALSE, "error in (no error)"=w2808) -> ("error out"=w2804:errorcluster)  [unwired: 12 in]
                n1190 = Merge Errors(w2804, w2804) -> (w2805:errorcluster)
              }
            }
            n1191 = call <userlib>:"Wait (ms)__ogtk.vi"("error in (no error)"=w2749, "milliseconds to wait"=u32 5) -> ("error out"=w2750:errorcluster)  [unwired: 8 in, 1 out]
            n1192 = flat-sequence {
              tunnel: [FALSE ("aborted?")] -> w2741
              tunnel: [w2803] -> w2740
              tunnel: w2731 -> [w2803]
              frame #0 {
              }
            }
          }
        }
        n1193 = local write "Depth Cluster"(w431) -> ()
      }
    }
  }
  n1194 = Merge Errors(w17, w16) -> (→"error out":errorcluster)
